vi "Results_file_Plotter.vi"() -> ()   [LabVIEW 2016]
uses:
  Anemometry/Anemometry Sub Vis/Data_plotting_vis/Plot_Slice.ctl
  Anemometry/Anemometry Sub Vis/Data_plotting_vis/Plotter_Mode.ctl
  Anemometry/Anemometry Sub Vis/Data_plotting_vis/Data_File_Type.ctl
  subVIs/PlotProperty.ctl
  Anemometry/Anemometry Sub Vis/File/Setup_Filetype.ctl
  Anemometry/Anemometry Sub Vis/Controls/Global_mode.ctl
  Anemometry/Anemometry Sub Vis/Data_plotting_vis/Error_bars_index.ctl
  Anemometry/Anemometry Sub Vis/Data_plotting_vis/Results_plotter_Global.vi
  Instance           1 28Saved   Results_file_Plotter .vi
  Anemometry/Anemometry Sub Vis/Globals/Constants_global.vi
  Anemometry/Anemometry Sub Vis/Globals/Trav_pos_global.vi
panel:
  out "Index when last displayed":i32
  out "Index when last plotted":i32
  in  "Tab Control":T1(tab)=enum."Cursor"
  in  "Template":path
  in  "Empty":bool
  in  "Result files to read":path[](array[path])
  in  "Add results file":bool
  in  "File Types to Read":T2
  in  "Dot Plot?":bool
  in  "Vector Plot?":bool
  out "2nd Add label":string
  out "First Add label":string
  in  "Additional X Values":dbl[](array[numeric]) format="%.2f"
  in  "Additional Y Values":dbl[](array[numeric]) format="%.2f"
  in  "Show Results Space Analysis":bool
  in  "Show Plot Space Analysis":bool
  in  "Multi Ordinate":i32[](listbox)
  in  "Multi Ordinate?":bool
  in  "Ordinate":u16(ring) items=["File", "Date", "Time", "Comments", "Uref", "Screens_Downstream of Heaters", "Spires", "Spires Used", "Roughness", "Roughness Used", "Roughness Elements 1st Row X(m)", "Start of Cooled Floor X(m)", "Chilled Water Temp", "Inlet_Temp Average", "Av Floor Temp", "Max deltaT", "X (mm)", "Y (mm)", "Z (mm)", "Z (m)", "U/Uref", "V/Uref", "W/Uref", "u^2/Uref^2", "v^2/Uref^2", "w^2/Uref^2", "uv/Uref^2", "-uw/Uref^2", "Corr wt", "Inlet Profile", "DeltaT", "t^2", "ut", "Corr ut", "wt", "Grad Ri", "Flux Ri", "B-V Freq N", "Inlet DeltaT", "DeltaT/DeltaTmax", "T thermistor", "dT/dZ", "dU/dZ", "Inlet Delta_Set", "u'/U", "w'/U", "W/U", "Location XY", "Location XZ", "U m/s", "V m/s", "W m/s", "u^2", "v^2", "w^2", "Speed/Uref", "T cw", "Flow Meas Time", "Profile", "t'/T", "t'", "uv", "uw", "EnFlo Lab Hygrometry Dew Point temp", "EnFlo Lab Hygrometry Dew Point temp_PN", "Multi Run Start Time", "T cw Offset A", "T cw Grad B", "LDA (U) Standard Error in Mean", "LDA (U) Standard Error in Variance", "LDA (V) Standard Error in Mean", "LDA (V) Standard Error in Variance", "LDA (W) Standard Error in Mean", "LDA (W) Standard Error in Variance", "U/Uref Err", "u^2/Uref^2 Err", "V/Uref Err", "v^2/Uref^2 Err", "W/Uref Err", "w^2/Uref^2 Err", "Inlet Temp", "Inlet Setpoint", "Inlet Temp Error", "Seconds since 1st Jan", "Uni Chilled Water Temp", "Raw Data Filename", "Inlet Temp Z=1450", "Inlet Temp Z=1350", "Inlet Temp Z=1250", "Inlet Temp Z=1150", "Inlet Temp Z=1050", "Inlet Temp Z=950", "Inlet Temp Z=850", "Inlet Temp Z=750", "Inlet Temp Z=650", "Inlet Temp Z=550", "Inlet Temp Z=450", "Inlet Temp Z=350", "Inlet Temp Z=250", "Inlet Temp Z=150", "Inlet Temp Z=50", "Inlet Setpoint Z=1450", "Inlet Setpoint Z=1350", "Inlet Setpoint Z=1250", "Inlet Setpoint Z=1150", "Inlet Setpoint Z=950", "Inlet Setpoint Z=850", "Inlet Setpoint Z=1050", "Inlet Setpoint Z=750", "Inlet Setpoint Z=650", "Inlet Setpoint Z=550", "Inlet Setpoint Z=450", "Inlet Setpoint Z=350", "Inlet Setpoint Z=250", "Inlet Setpoint Z=150", "Inlet Setpoint Z=50", "Temp Floor_Near 1", "Temp Floor_Far 1", "Temp Floor_Near 2", "Temp Floor_Far 2", "Temp Floor_Near 3", "Temp Floor_Far 3", "Temp Floor_Near 4", "Temp Floor_Far 4", "Temp Floor_Near 5", "Temp Floor_Far 5", "Temp Floor_Near 6", "Temp Floor_Far 6", "Temp Floor_Near 7", "Temp Floor_Far 7", "Temp Floor_Near 8", "Temp Floor_Far 8", "Temp Floor_Near 9", "Temp Floor_Far 9", "Temp Floor_Near 10", "Temp Floor_Far 10", "Temp Floor_Near 11", "Temp Floor_Far 11", "Temp Floor_Near 12", "Temp Floor_Far 12", "LDA (U) E(f)", "LDA (W) E(f)", "CW (T) f.E(f)", "LDA (U) f.E(f)", "LDA (W) f.E(f)", "Folder", "Inst", "EnFlo_Tunnel Usonic_Ref_3 Velocity", "EnFlo_Tunnel Usonic Y+ve Duct Velocity", "EnFlo_Tunnel Usonic Y-ve Duct Velocity", "EnFlo_Tunnel Shaft rpm", "U/Uref3", "U/U_y+ve", "U/U_y-ve", "EnFlo_Tunnel Inlet K_Factor", "LDA U SamplingRate", "LDA W SamplingRate", "EnFlo_Tunnel Chilled Water Valve Dem Pos", "EnFlo_Tunnel Temp Y+ve_Side_Top", "EnFlo_Tunnel Temp Y+ve_Side_Middle", "EnFlo_Tunnel Temp Y+ve_Side_Bottom", "EnFlo_Tunnel Temp Y-ve_Side_Top", "EnFlo_Tunnel Temp Y-ve_Side_Middle", "EnFlo_Tunnel Temp Y-ve_Side_Bottom", "EnFlo Lab labstrat1 Delta T", "University Outside Temp", "EnFlo Lab Hygrometry Rel Humidity", "EnFlo_Tunnel Temp LDA Probe", "Pre Inlet Average Temp", "Inlet Temp At LDA (U) Z", "Hydrosonic Transducer Setting", "EnFlo_Tunnel Pressure Static", "EnFlo_Tunnel Trav1 Pos Z", "EnFlo_Tunnel Trav1 Pos Y", "EnFlo_Tunnel Trav1 Pos X", "speed/Uref", "Turbine", "EnFlo_Tunnel Metadata Hub_1 Xpos", "X/D", "EnFlo_Tunnel Therm 25mm Below Cold Wire", "WT_RPM", "WT_rpm^2", "WT_rpmSkewness", "WT_rpmKurtosis", "WT_rpm'_%", "LDA Laser Green LDD current (A)", "LDA Laser Blue LDD current (A)", "Cold Wire Displacement_X_(mm)", "Aero_Tunnel Speed Meas Velocity", "LDA (U) Timescale Estimate Integrated to 25%", "LDA (W) Timescale Estimate Integrated to 25%", "Frequency (Hz)", "Green LDA (U) E(f)", "EnFlo_Tunnel Ref Pitot Velocity", "Upitot/Uref", "CW (T) Mean Voltage", "K Factor 1st Honeycomb", "K Factor 1st Screen", "K Factor 2nd_Screen", "K Factor 2nd Honeycomb Heaters Screen", "LDA (U) & LDA (W) Standard Error uw", "-uw/Uref^2 Err", "Multi Run Row Number", "EnFlo_Tunnel Exit Duct Top Temp", "EnFlo_Tunnel Exit Duct Temp", "Av Exit Duct Temp", "Heat Ex Div Valve Dem Pos", "EnFlo_Tunnel Exit Duct Dem Temp", "Inlet Temp St Deviation", "Inlet Door Heaters Dem Power%"]
  in  "Intensity Plot?":bool
  in  "Absisca":u16(ring) items=["File", "Date", "Time", "Comments", "Uref", "Screens_Downstream of Heaters", "Spires", "Spires Used", "Roughness", "Roughness Used", "Roughness Elements 1st Row X(m)", "Start of Cooled Floor X(m)", "Chilled Water Temp", "Inlet_Temp Average", "Av Floor Temp", "Max deltaT", "X (mm)", "Y (mm)", "Z (mm)", "Z (m)", "U/Uref", "V/Uref", "W/Uref", "u^2/Uref^2", "v^2/Uref^2", "w^2/Uref^2", "uv/Uref^2", "-uw/Uref^2", "Corr wt", "Inlet Profile", "DeltaT", "t^2", "ut", "Corr ut", "wt", "Grad Ri", "Flux Ri", "B-V Freq N", "Inlet DeltaT", "DeltaT/DeltaTmax", "T thermistor", "dT/dZ", "dU/dZ", "Inlet Delta_Set", "u'/U", "w'/U", "W/U", "Location XY", "Location XZ", "U m/s", "V m/s", "W m/s", "u^2", "v^2", "w^2", "Speed/Uref", "T cw", "Flow Meas Time", "Profile", "t'/T", "t'", "uv", "uw", "EnFlo Lab Hygrometry Dew Point temp", "EnFlo Lab Hygrometry Dew Point temp_PN", "Multi Run Start Time", "T cw Offset A", "T cw Grad B", "LDA (U) Standard Error in Mean", "LDA (U) Standard Error in Variance", "LDA (V) Standard Error in Mean", "LDA (V) Standard Error in Variance", "LDA (W) Standard Error in Mean", "LDA (W) Standard Error in Variance", "U/Uref Err", "u^2/Uref^2 Err", "V/Uref Err", "v^2/Uref^2 Err", "W/Uref Err", "w^2/Uref^2 Err", "Inlet Temp", "Inlet Setpoint", "Inlet Temp Error", "Seconds since 1st Jan", "Uni Chilled Water Temp", "Raw Data Filename", "Inlet Temp Z=1450", "Inlet Temp Z=1350", "Inlet Temp Z=1250", "Inlet Temp Z=1150", "Inlet Temp Z=1050", "Inlet Temp Z=950", "Inlet Temp Z=850", "Inlet Temp Z=750", "Inlet Temp Z=650", "Inlet Temp Z=550", "Inlet Temp Z=450", "Inlet Temp Z=350", "Inlet Temp Z=250", "Inlet Temp Z=150", "Inlet Temp Z=50", "Inlet Setpoint Z=1450", "Inlet Setpoint Z=1350", "Inlet Setpoint Z=1250", "Inlet Setpoint Z=1150", "Inlet Setpoint Z=950", "Inlet Setpoint Z=850", "Inlet Setpoint Z=1050", "Inlet Setpoint Z=750", "Inlet Setpoint Z=650", "Inlet Setpoint Z=550", "Inlet Setpoint Z=450", "Inlet Setpoint Z=350", "Inlet Setpoint Z=250", "Inlet Setpoint Z=150", "Inlet Setpoint Z=50", "Temp Floor_Near 1", "Temp Floor_Far 1", "Temp Floor_Near 2", "Temp Floor_Far 2", "Temp Floor_Near 3", "Temp Floor_Far 3", "Temp Floor_Near 4", "Temp Floor_Far 4", "Temp Floor_Near 5", "Temp Floor_Far 5", "Temp Floor_Near 6", "Temp Floor_Far 6", "Temp Floor_Near 7", "Temp Floor_Far 7", "Temp Floor_Near 8", "Temp Floor_Far 8", "Temp Floor_Near 9", "Temp Floor_Far 9", "Temp Floor_Near 10", "Temp Floor_Far 10", "Temp Floor_Near 11", "Temp Floor_Far 11", "Temp Floor_Near 12", "Temp Floor_Far 12", "LDA (U) E(f)", "LDA (W) E(f)", "CW (T) f.E(f)", "LDA (U) f.E(f)", "LDA (W) f.E(f)", "Folder", "Inst", "EnFlo_Tunnel Usonic_Ref_3 Velocity", "EnFlo_Tunnel Usonic Y+ve Duct Velocity", "EnFlo_Tunnel Usonic Y-ve Duct Velocity", "EnFlo_Tunnel Shaft rpm", "U/Uref3", "U/U_y+ve", "U/U_y-ve", "EnFlo_Tunnel Inlet K_Factor", "LDA U SamplingRate", "LDA W SamplingRate", "EnFlo_Tunnel Chilled Water Valve Dem Pos", "EnFlo_Tunnel Temp Y+ve_Side_Top", "EnFlo_Tunnel Temp Y+ve_Side_Middle", "EnFlo_Tunnel Temp Y+ve_Side_Bottom", "EnFlo_Tunnel Temp Y-ve_Side_Top", "EnFlo_Tunnel Temp Y-ve_Side_Middle", "EnFlo_Tunnel Temp Y-ve_Side_Bottom", "EnFlo Lab labstrat1 Delta T", "University Outside Temp", "EnFlo Lab Hygrometry Rel Humidity", "EnFlo_Tunnel Temp LDA Probe", "Pre Inlet Average Temp", "Inlet Temp At LDA (U) Z", "Hydrosonic Transducer Setting", "EnFlo_Tunnel Pressure Static", "EnFlo_Tunnel Trav1 Pos Z", "EnFlo_Tunnel Trav1 Pos Y", "EnFlo_Tunnel Trav1 Pos X", "speed/Uref", "Turbine", "EnFlo_Tunnel Metadata Hub_1 Xpos", "X/D", "EnFlo_Tunnel Therm 25mm Below Cold Wire", "WT_RPM", "WT_rpm^2", "WT_rpmSkewness", "WT_rpmKurtosis", "WT_rpm'_%", "LDA Laser Green LDD current (A)", "LDA Laser Blue LDD current (A)", "Cold Wire Displacement_X_(mm)", "Aero_Tunnel Speed Meas Velocity", "LDA (U) Timescale Estimate Integrated to 25%", "LDA (W) Timescale Estimate Integrated to 25%", "Frequency (Hz)", "Green LDA (U) E(f)", "EnFlo_Tunnel Ref Pitot Velocity", "Upitot/Uref", "CW (T) Mean Voltage", "K Factor 1st Honeycomb", "K Factor 1st Screen", "K Factor 2nd_Screen", "K Factor 2nd Honeycomb Heaters Screen", "LDA (U) & LDA (W) Standard Error uw", "-uw/Uref^2 Err", "Multi Run Row Number", "EnFlo_Tunnel Exit Duct Top Temp", "EnFlo_Tunnel Exit Duct Temp", "Av Exit Duct Temp", "Heat Ex Div Valve Dem Pos", "EnFlo_Tunnel Exit Duct Dem Temp", "Inlet Temp St Deviation", "Inlet Door Heaters Dem Power%"]
  in  "Job Directory":path
  in  "Save Averaged rows":bool
  in  "Save Surface Fit":bool
  in  "Output Filename":path
  in  "Save Data in Rows":bool
  in  "Save Plot data":bool
  in  "Header":string
  in  "Process Point":bool
  in  "Kill Point":bool
  out "Table":string[][](table)
  in  "ShowPix":bool
  in  "Post Process Plotted Data":bool
  in  "...using routine":string
  in  "Calculate new metadata":bool
  in  "Add /Edit metadata":bool
  in  "Delete Plotted data from file":bool
  in  "Raw DF in Orig Pos?":bool
  in  "Edit Raw Data Files?":bool
  in  "Save Setup":bool
  in  "Load Setup":bool
  in  "Save Setup Interval (s)":dbl=600.0
  out "Uadvec":dbl
  in  "Ordinate Name":string
  in  "Filter 6":u16(ring)
  in  "Add Inlet Temperature offset":bool
  in  "Plot EnFlo Tunnel Display":bool
  in  "SeriesColouring":T4={"PlotVariable"=enum."Symbol", "YellowSelector"=enum."Colour", "RedSelector"=enum."Shade"}
  in  "InterpolationStyle":T5(ring)=enum."Line"
  in  "TinyPoints?":bool
  in  "stop":bool
  out "Current":string="Graph Scales"
  in  "Single Series":i32[](listbox)=[0]
  in  "Edit Template File":bool
  out "nRows":i32
  in  "Filter Bins 2":i32[](listbox)=[0]
  in  "Filter 5":u16(ring) items=["Show All (33)", "03-Jan-17 (33)", "NOT 03-Jan-17 (0)"]
  in  "Filter 4":u16(ring) items=["Show All (33)", "BLANK (33)", "NOT BLANK (0)"]
  in  "Filter 3":u16(ring) items=["Show All (33)", "#DIV/0! (2)", "Single Measurement (31)", "NOT #DIV/0! (31)", "NOT Single Measurement (2)"]
  in  "Filter Array":u16[](array[ring])=[0, 0, 0, 0, 0, 0] items=["Don't Filter", "File", "Date", "Time", "Comments", "Uref", "Screens_Downstream of Heaters", "Spires", "Spires Used", "Roughness", "Roughness Used", "Roughness Elements 1st Row X(m)", "Start of Cooled Floor X(m)", "Chilled Water Temp", "Inlet_Temp Average", "Av Floor Temp", "Max deltaT", "X (mm)", "Y (mm)", "Z (mm)", "Z (m)", "U/Uref", "V/Uref", "W/Uref", "u^2/Uref^2", "v^2/Uref^2", "w^2/Uref^2", "uv/Uref^2", "-uw/Uref^2", "Corr wt", "Inlet Profile", "DeltaT", "t^2", "ut", "Corr ut", "wt", "Grad Ri", "Flux Ri", "B-V Freq N", "Inlet DeltaT", "DeltaT/DeltaTmax", "T thermistor", "dT/dZ", "dU/dZ", "Inlet Delta_Set", "u'/U", "w'/U", "W/U", "Location XY", "Location XZ", "U m/s", "V m/s", "W m/s", "u^2", "v^2", "w^2", "Speed/Uref", "T cw", "Flow Meas Time", "Profile", "t'/T", "t'", "uv", "uw", "EnFlo Lab Hygrometry Dew Point temp", "EnFlo Lab Hygrometry Dew Point temp_PN", "Multi Run Start Time", "T cw Offset A", "T cw Grad B", "LDA (U) Standard Error in Mean", "LDA (U) Standard Error in Variance", "LDA (V) Standard Error in Mean", "LDA (V) Standard Error in Variance", "LDA (W) Standard Error in Mean", "LDA (W) Standard Error in Variance", "U/Uref Err", "u^2/Uref^2 Err", "V/Uref Err", "v^2/Uref^2 Err", "W/Uref Err", "w^2/Uref^2 Err", "Inlet Temp", "Inlet Setpoint", "Inlet Temp Error", "Seconds since 1st Jan", "Uni Chilled Water Temp", "Raw Data Filename", "Inlet Temp Z=1450", "Inlet Temp Z=1350", "Inlet Temp Z=1250", "Inlet Temp Z=1150", "Inlet Temp Z=1050", "Inlet Temp Z=950", "Inlet Temp Z=850", "Inlet Temp Z=750", "Inlet Temp Z=650", "Inlet Temp Z=550", "Inlet Temp Z=450", "Inlet Temp Z=350", "Inlet Temp Z=250", "Inlet Temp Z=150", "Inlet Temp Z=50", "Inlet Setpoint Z=1450", "Inlet Setpoint Z=1350", "Inlet Setpoint Z=1250", "Inlet Setpoint Z=1150", "Inlet Setpoint Z=950", "Inlet Setpoint Z=850", "Inlet Setpoint Z=1050", "Inlet Setpoint Z=750", "Inlet Setpoint Z=650", "Inlet Setpoint Z=550", "Inlet Setpoint Z=450", "Inlet Setpoint Z=350", "Inlet Setpoint Z=250", "Inlet Setpoint Z=150", "Inlet Setpoint Z=50", "Temp Floor_Near 1", "Temp Floor_Far 1", "Temp Floor_Near 2", "Temp Floor_Far 2", "Temp Floor_Near 3", "Temp Floor_Far 3", "Temp Floor_Near 4", "Temp Floor_Far 4", "Temp Floor_Near 5", "Temp Floor_Far 5", "Temp Floor_Near 6", "Temp Floor_Far 6", "Temp Floor_Near 7", "Temp Floor_Far 7", "Temp Floor_Near 8", "Temp Floor_Far 8", "Temp Floor_Near 9", "Temp Floor_Far 9", "Temp Floor_Near 10", "Temp Floor_Far 10", "Temp Floor_Near 11", "Temp Floor_Far 11", "Temp Floor_Near 12", "Temp Floor_Far 12", "LDA (U) E(f)", "LDA (W) E(f)", "CW (T) f.E(f)", "LDA (U) f.E(f)", "LDA (W) f.E(f)", "Folder", "Inst", "EnFlo_Tunnel Usonic_Ref_3 Velocity", "EnFlo_Tunnel Usonic Y+ve Duct Velocity", "EnFlo_Tunnel Usonic Y-ve Duct Velocity", "EnFlo_Tunnel Shaft rpm", "U/Uref3", "U/U_y+ve", "U/U_y-ve", "EnFlo_Tunnel Inlet K_Factor", "LDA U SamplingRate", "LDA W SamplingRate", "EnFlo_Tunnel Chilled Water Valve Dem Pos", "EnFlo_Tunnel Temp Y+ve_Side_Top", "EnFlo_Tunnel Temp Y+ve_Side_Middle", "EnFlo_Tunnel Temp Y+ve_Side_Bottom", "EnFlo_Tunnel Temp Y-ve_Side_Top", "EnFlo_Tunnel Temp Y-ve_Side_Middle", "EnFlo_Tunnel Temp Y-ve_Side_Bottom", "EnFlo Lab labstrat1 Delta T", "University Outside Temp", "EnFlo Lab Hygrometry Rel Humidity", "EnFlo_Tunnel Temp LDA Probe", "Pre Inlet Average Temp", "Inlet Temp At LDA (U) Z", "Hydrosonic Transducer Setting", "EnFlo_Tunnel Pressure Static", "EnFlo_Tunnel Trav1 Pos Z", "EnFlo_Tunnel Trav1 Pos Y", "EnFlo_Tunnel Trav1 Pos X", "speed/Uref", "Turbine", "EnFlo_Tunnel Metadata Hub_1 Xpos", "X/D", "EnFlo_Tunnel Therm 25mm Below Cold Wire", "WT_RPM", "WT_rpm^2", "WT_rpmSkewness", "WT_rpmKurtosis", "WT_rpm'_%", "LDA Laser Green LDD current (A)", "LDA Laser Blue LDD current (A)", "Cold Wire Displacement_X_(mm)", "Aero_Tunnel Speed Meas Velocity", "LDA (U) Timescale Estimate Integrated to 25%", "LDA (W) Timescale Estimate Integrated to 25%", "Frequency (Hz)", "Green LDA (U) E(f)", "EnFlo_Tunnel Ref Pitot Velocity", "Upitot/Uref", "CW (T) Mean Voltage", "K Factor 1st Honeycomb", "K Factor 1st Screen", "K Factor 2nd_Screen", "K Factor 2nd Honeycomb Heaters Screen", "LDA (U) & LDA (W) Standard Error uw", "-uw/Uref^2 Err", "Multi Run Row Number", "EnFlo_Tunnel Exit Duct Top Temp", "EnFlo_Tunnel Exit Duct Temp", "Av Exit Duct Temp", "Heat Ex Div Valve Dem Pos", "EnFlo_Tunnel Exit Duct Dem Temp", "Inlet Temp St Deviation", "Inlet Door Heaters Dem Power%"]
  in  "Filter Bins 1":i32[](listbox)=[0]
  in  "Create picture Vi Name":string caption="Picture VI:"
  in  "Save Plot as jpg":bool
  in  "Reload Files":bool
  in  "color and symbol":bool
  out "Selected Row":i32
  out "Selected Row?":bool
  out "Warning!":string
  out "XY Plot":cluster{dbl[], dbl[]}[](graph)
  out "Edit Raw Data Header Info":bool
  out "Intensity Graph":dbl[][](graph)
  in  "Bkgnd Value":dbl
  in  "Update":bool
  in  "Plot Resolution":bool
  in  "Point Size":i32(slide)=1 scale=0.0..10.0
  in  "No of Contours":i32=20
  in  "Slice mode":T6
  in  "Z Ch Name":u16(ring) items=["File", "Date", "Time", "Comments", "Uref", "Screens_Downstream of Heaters", "Spires", "Spires Used", "Roughness", "Roughness Used", "Roughness Elements 1st Row X(m)", "Start of Cooled Floor X(m)", "Chilled Water Temp", "Inlet_Temp Average", "Av Floor Temp", "Max deltaT", "X (mm)", "Y (mm)", "Z (mm)", "Z (m)", "U/Uref", "V/Uref", "W/Uref", "u^2/Uref^2", "v^2/Uref^2", "w^2/Uref^2", "uv/Uref^2", "-uw/Uref^2", "Corr wt", "Inlet Profile", "DeltaT", "t^2", "ut", "Corr ut", "wt", "Grad Ri", "Flux Ri", "B-V Freq N", "Inlet DeltaT", "DeltaT/DeltaTmax", "T thermistor", "dT/dZ", "dU/dZ", "Inlet Delta_Set", "u'/U", "w'/U", "W/U", "Location XY", "Location XZ", "U m/s", "V m/s", "W m/s", "u^2", "v^2", "w^2", "Speed/Uref", "T cw", "Flow Meas Time", "Profile", "t'/T", "t'", "uv", "uw", "EnFlo Lab Hygrometry Dew Point temp", "EnFlo Lab Hygrometry Dew Point temp_PN", "Multi Run Start Time", "T cw Offset A", "T cw Grad B", "LDA (U) Standard Error in Mean", "LDA (U) Standard Error in Variance", "LDA (V) Standard Error in Mean", "LDA (V) Standard Error in Variance", "LDA (W) Standard Error in Mean", "LDA (W) Standard Error in Variance", "U/Uref Err", "u^2/Uref^2 Err", "V/Uref Err", "v^2/Uref^2 Err", "W/Uref Err", "w^2/Uref^2 Err", "Inlet Temp", "Inlet Setpoint", "Inlet Temp Error", "Seconds since 1st Jan", "Uni Chilled Water Temp", "Raw Data Filename", "Inlet Temp Z=1450", "Inlet Temp Z=1350", "Inlet Temp Z=1250", "Inlet Temp Z=1150", "Inlet Temp Z=1050", "Inlet Temp Z=950", "Inlet Temp Z=850", "Inlet Temp Z=750", "Inlet Temp Z=650", "Inlet Temp Z=550", "Inlet Temp Z=450", "Inlet Temp Z=350", "Inlet Temp Z=250", "Inlet Temp Z=150", "Inlet Temp Z=50", "Inlet Setpoint Z=1450", "Inlet Setpoint Z=1350", "Inlet Setpoint Z=1250", "Inlet Setpoint Z=1150", "Inlet Setpoint Z=950", "Inlet Setpoint Z=850", "Inlet Setpoint Z=1050", "Inlet Setpoint Z=750", "Inlet Setpoint Z=650", "Inlet Setpoint Z=550", "Inlet Setpoint Z=450", "Inlet Setpoint Z=350", "Inlet Setpoint Z=250", "Inlet Setpoint Z=150", "Inlet Setpoint Z=50", "Temp Floor_Near 1", "Temp Floor_Far 1", "Temp Floor_Near 2", "Temp Floor_Far 2", "Temp Floor_Near 3", "Temp Floor_Far 3", "Temp Floor_Near 4", "Temp Floor_Far 4", "Temp Floor_Near 5", "Temp Floor_Far 5", "Temp Floor_Near 6", "Temp Floor_Far 6", "Temp Floor_Near 7", "Temp Floor_Far 7", "Temp Floor_Near 8", "Temp Floor_Far 8", "Temp Floor_Near 9", "Temp Floor_Far 9", "Temp Floor_Near 10", "Temp Floor_Far 10", "Temp Floor_Near 11", "Temp Floor_Far 11", "Temp Floor_Near 12", "Temp Floor_Far 12", "LDA (U) E(f)", "LDA (W) E(f)", "CW (T) f.E(f)", "LDA (U) f.E(f)", "LDA (W) f.E(f)", "Folder", "Inst", "EnFlo_Tunnel Usonic_Ref_3 Velocity", "EnFlo_Tunnel Usonic Y+ve Duct Velocity", "EnFlo_Tunnel Usonic Y-ve Duct Velocity", "EnFlo_Tunnel Shaft rpm", "U/Uref3", "U/U_y+ve", "U/U_y-ve", "EnFlo_Tunnel Inlet K_Factor", "LDA U SamplingRate", "LDA W SamplingRate", "EnFlo_Tunnel Chilled Water Valve Dem Pos", "EnFlo_Tunnel Temp Y+ve_Side_Top", "EnFlo_Tunnel Temp Y+ve_Side_Middle", "EnFlo_Tunnel Temp Y+ve_Side_Bottom", "EnFlo_Tunnel Temp Y-ve_Side_Top", "EnFlo_Tunnel Temp Y-ve_Side_Middle", "EnFlo_Tunnel Temp Y-ve_Side_Bottom", "EnFlo Lab labstrat1 Delta T", "University Outside Temp", "EnFlo Lab Hygrometry Rel Humidity", "EnFlo_Tunnel Temp LDA Probe", "Pre Inlet Average Temp", "Inlet Temp At LDA (U) Z", "Hydrosonic Transducer Setting", "EnFlo_Tunnel Pressure Static", "EnFlo_Tunnel Trav1 Pos Z", "EnFlo_Tunnel Trav1 Pos Y", "EnFlo_Tunnel Trav1 Pos X", "speed/Uref", "Turbine", "EnFlo_Tunnel Metadata Hub_1 Xpos", "X/D", "EnFlo_Tunnel Therm 25mm Below Cold Wire", "WT_RPM", "WT_rpm^2", "WT_rpmSkewness", "WT_rpmKurtosis", "WT_rpm'_%", "LDA Laser Green LDD current (A)", "LDA Laser Blue LDD current (A)", "Cold Wire Displacement_X_(mm)", "Aero_Tunnel Speed Meas Velocity", "LDA (U) Timescale Estimate Integrated to 25%", "LDA (W) Timescale Estimate Integrated to 25%", "Frequency (Hz)", "Green LDA (U) E(f)", "EnFlo_Tunnel Ref Pitot Velocity", "Upitot/Uref", "CW (T) Mean Voltage", "K Factor 1st Honeycomb", "K Factor 1st Screen", "K Factor 2nd_Screen", "K Factor 2nd Honeycomb Heaters Screen", "LDA (U) & LDA (W) Standard Error uw", "-uw/Uref^2 Err", "Multi Run Row Number", "EnFlo_Tunnel Exit Duct Top Temp", "EnFlo_Tunnel Exit Duct Temp", "Av Exit Duct Temp", "Heat Ex Div Valve Dem Pos", "EnFlo_Tunnel Exit Duct Dem Temp", "Inlet Temp St Deviation", "Inlet Door Heaters Dem Power%"]
  in  "Y Ch Name":u16(ring) items=["File", "Date", "Time", "Comments", "Uref", "Screens_Downstream of Heaters", "Spires", "Spires Used", "Roughness", "Roughness Used", "Roughness Elements 1st Row X(m)", "Start of Cooled Floor X(m)", "Chilled Water Temp", "Inlet_Temp Average", "Av Floor Temp", "Max deltaT", "X (mm)", "Y (mm)", "Z (mm)", "Z (m)", "U/Uref", "V/Uref", "W/Uref", "u^2/Uref^2", "v^2/Uref^2", "w^2/Uref^2", "uv/Uref^2", "-uw/Uref^2", "Corr wt", "Inlet Profile", "DeltaT", "t^2", "ut", "Corr ut", "wt", "Grad Ri", "Flux Ri", "B-V Freq N", "Inlet DeltaT", "DeltaT/DeltaTmax", "T thermistor", "dT/dZ", "dU/dZ", "Inlet Delta_Set", "u'/U", "w'/U", "W/U", "Location XY", "Location XZ", "U m/s", "V m/s", "W m/s", "u^2", "v^2", "w^2", "Speed/Uref", "T cw", "Flow Meas Time", "Profile", "t'/T", "t'", "uv", "uw", "EnFlo Lab Hygrometry Dew Point temp", "EnFlo Lab Hygrometry Dew Point temp_PN", "Multi Run Start Time", "T cw Offset A", "T cw Grad B", "LDA (U) Standard Error in Mean", "LDA (U) Standard Error in Variance", "LDA (V) Standard Error in Mean", "LDA (V) Standard Error in Variance", "LDA (W) Standard Error in Mean", "LDA (W) Standard Error in Variance", "U/Uref Err", "u^2/Uref^2 Err", "V/Uref Err", "v^2/Uref^2 Err", "W/Uref Err", "w^2/Uref^2 Err", "Inlet Temp", "Inlet Setpoint", "Inlet Temp Error", "Seconds since 1st Jan", "Uni Chilled Water Temp", "Raw Data Filename", "Inlet Temp Z=1450", "Inlet Temp Z=1350", "Inlet Temp Z=1250", "Inlet Temp Z=1150", "Inlet Temp Z=1050", "Inlet Temp Z=950", "Inlet Temp Z=850", "Inlet Temp Z=750", "Inlet Temp Z=650", "Inlet Temp Z=550", "Inlet Temp Z=450", "Inlet Temp Z=350", "Inlet Temp Z=250", "Inlet Temp Z=150", "Inlet Temp Z=50", "Inlet Setpoint Z=1450", "Inlet Setpoint Z=1350", "Inlet Setpoint Z=1250", "Inlet Setpoint Z=1150", "Inlet Setpoint Z=950", "Inlet Setpoint Z=850", "Inlet Setpoint Z=1050", "Inlet Setpoint Z=750", "Inlet Setpoint Z=650", "Inlet Setpoint Z=550", "Inlet Setpoint Z=450", "Inlet Setpoint Z=350", "Inlet Setpoint Z=250", "Inlet Setpoint Z=150", "Inlet Setpoint Z=50", "Temp Floor_Near 1", "Temp Floor_Far 1", "Temp Floor_Near 2", "Temp Floor_Far 2", "Temp Floor_Near 3", "Temp Floor_Far 3", "Temp Floor_Near 4", "Temp Floor_Far 4", "Temp Floor_Near 5", "Temp Floor_Far 5", "Temp Floor_Near 6", "Temp Floor_Far 6", "Temp Floor_Near 7", "Temp Floor_Far 7", "Temp Floor_Near 8", "Temp Floor_Far 8", "Temp Floor_Near 9", "Temp Floor_Far 9", "Temp Floor_Near 10", "Temp Floor_Far 10", "Temp Floor_Near 11", "Temp Floor_Far 11", "Temp Floor_Near 12", "Temp Floor_Far 12", "LDA (U) E(f)", "LDA (W) E(f)", "CW (T) f.E(f)", "LDA (U) f.E(f)", "LDA (W) f.E(f)", "Folder", "Inst", "EnFlo_Tunnel Usonic_Ref_3 Velocity", "EnFlo_Tunnel Usonic Y+ve Duct Velocity", "EnFlo_Tunnel Usonic Y-ve Duct Velocity", "EnFlo_Tunnel Shaft rpm", "U/Uref3", "U/U_y+ve", "U/U_y-ve", "EnFlo_Tunnel Inlet K_Factor", "LDA U SamplingRate", "LDA W SamplingRate", "EnFlo_Tunnel Chilled Water Valve Dem Pos", "EnFlo_Tunnel Temp Y+ve_Side_Top", "EnFlo_Tunnel Temp Y+ve_Side_Middle", "EnFlo_Tunnel Temp Y+ve_Side_Bottom", "EnFlo_Tunnel Temp Y-ve_Side_Top", "EnFlo_Tunnel Temp Y-ve_Side_Middle", "EnFlo_Tunnel Temp Y-ve_Side_Bottom", "EnFlo Lab labstrat1 Delta T", "University Outside Temp", "EnFlo Lab Hygrometry Rel Humidity", "EnFlo_Tunnel Temp LDA Probe", "Pre Inlet Average Temp", "Inlet Temp At LDA (U) Z", "Hydrosonic Transducer Setting", "EnFlo_Tunnel Pressure Static", "EnFlo_Tunnel Trav1 Pos Z", "EnFlo_Tunnel Trav1 Pos Y", "EnFlo_Tunnel Trav1 Pos X", "speed/Uref", "Turbine", "EnFlo_Tunnel Metadata Hub_1 Xpos", "X/D", "EnFlo_Tunnel Therm 25mm Below Cold Wire", "WT_RPM", "WT_rpm^2", "WT_rpmSkewness", "WT_rpmKurtosis", "WT_rpm'_%", "LDA Laser Green LDD current (A)", "LDA Laser Blue LDD current (A)", "Cold Wire Displacement_X_(mm)", "Aero_Tunnel Speed Meas Velocity", "LDA (U) Timescale Estimate Integrated to 25%", "LDA (W) Timescale Estimate Integrated to 25%", "Frequency (Hz)", "Green LDA (U) E(f)", "EnFlo_Tunnel Ref Pitot Velocity", "Upitot/Uref", "CW (T) Mean Voltage", "K Factor 1st Honeycomb", "K Factor 1st Screen", "K Factor 2nd_Screen", "K Factor 2nd Honeycomb Heaters Screen", "LDA (U) & LDA (W) Standard Error uw", "-uw/Uref^2 Err", "Multi Run Row Number", "EnFlo_Tunnel Exit Duct Top Temp", "EnFlo_Tunnel Exit Duct Temp", "Av Exit Duct Temp", "Heat Ex Div Valve Dem Pos", "EnFlo_Tunnel Exit Duct Dem Temp", "Inlet Temp St Deviation", "Inlet Door Heaters Dem Power%"]
  in  "X Ch Name":u16(ring) items=["File", "Date", "Time", "Comments", "Uref", "Screens_Downstream of Heaters", "Spires", "Spires Used", "Roughness", "Roughness Used", "Roughness Elements 1st Row X(m)", "Start of Cooled Floor X(m)", "Chilled Water Temp", "Inlet_Temp Average", "Av Floor Temp", "Max deltaT", "X (mm)", "Y (mm)", "Z (mm)", "Z (m)", "U/Uref", "V/Uref", "W/Uref", "u^2/Uref^2", "v^2/Uref^2", "w^2/Uref^2", "uv/Uref^2", "-uw/Uref^2", "Corr wt", "Inlet Profile", "DeltaT", "t^2", "ut", "Corr ut", "wt", "Grad Ri", "Flux Ri", "B-V Freq N", "Inlet DeltaT", "DeltaT/DeltaTmax", "T thermistor", "dT/dZ", "dU/dZ", "Inlet Delta_Set", "u'/U", "w'/U", "W/U", "Location XY", "Location XZ", "U m/s", "V m/s", "W m/s", "u^2", "v^2", "w^2", "Speed/Uref", "T cw", "Flow Meas Time", "Profile", "t'/T", "t'", "uv", "uw", "EnFlo Lab Hygrometry Dew Point temp", "EnFlo Lab Hygrometry Dew Point temp_PN", "Multi Run Start Time", "T cw Offset A", "T cw Grad B", "LDA (U) Standard Error in Mean", "LDA (U) Standard Error in Variance", "LDA (V) Standard Error in Mean", "LDA (V) Standard Error in Variance", "LDA (W) Standard Error in Mean", "LDA (W) Standard Error in Variance", "U/Uref Err", "u^2/Uref^2 Err", "V/Uref Err", "v^2/Uref^2 Err", "W/Uref Err", "w^2/Uref^2 Err", "Inlet Temp", "Inlet Setpoint", "Inlet Temp Error", "Seconds since 1st Jan", "Uni Chilled Water Temp", "Raw Data Filename", "Inlet Temp Z=1450", "Inlet Temp Z=1350", "Inlet Temp Z=1250", "Inlet Temp Z=1150", "Inlet Temp Z=1050", "Inlet Temp Z=950", "Inlet Temp Z=850", "Inlet Temp Z=750", "Inlet Temp Z=650", "Inlet Temp Z=550", "Inlet Temp Z=450", "Inlet Temp Z=350", "Inlet Temp Z=250", "Inlet Temp Z=150", "Inlet Temp Z=50", "Inlet Setpoint Z=1450", "Inlet Setpoint Z=1350", "Inlet Setpoint Z=1250", "Inlet Setpoint Z=1150", "Inlet Setpoint Z=950", "Inlet Setpoint Z=850", "Inlet Setpoint Z=1050", "Inlet Setpoint Z=750", "Inlet Setpoint Z=650", "Inlet Setpoint Z=550", "Inlet Setpoint Z=450", "Inlet Setpoint Z=350", "Inlet Setpoint Z=250", "Inlet Setpoint Z=150", "Inlet Setpoint Z=50", "Temp Floor_Near 1", "Temp Floor_Far 1", "Temp Floor_Near 2", "Temp Floor_Far 2", "Temp Floor_Near 3", "Temp Floor_Far 3", "Temp Floor_Near 4", "Temp Floor_Far 4", "Temp Floor_Near 5", "Temp Floor_Far 5", "Temp Floor_Near 6", "Temp Floor_Far 6", "Temp Floor_Near 7", "Temp Floor_Far 7", "Temp Floor_Near 8", "Temp Floor_Far 8", "Temp Floor_Near 9", "Temp Floor_Far 9", "Temp Floor_Near 10", "Temp Floor_Far 10", "Temp Floor_Near 11", "Temp Floor_Far 11", "Temp Floor_Near 12", "Temp Floor_Far 12", "LDA (U) E(f)", "LDA (W) E(f)", "CW (T) f.E(f)", "LDA (U) f.E(f)", "LDA (W) f.E(f)", "Folder", "Inst", "EnFlo_Tunnel Usonic_Ref_3 Velocity", "EnFlo_Tunnel Usonic Y+ve Duct Velocity", "EnFlo_Tunnel Usonic Y-ve Duct Velocity", "EnFlo_Tunnel Shaft rpm", "U/Uref3", "U/U_y+ve", "U/U_y-ve", "EnFlo_Tunnel Inlet K_Factor", "LDA U SamplingRate", "LDA W SamplingRate", "EnFlo_Tunnel Chilled Water Valve Dem Pos", "EnFlo_Tunnel Temp Y+ve_Side_Top", "EnFlo_Tunnel Temp Y+ve_Side_Middle", "EnFlo_Tunnel Temp Y+ve_Side_Bottom", "EnFlo_Tunnel Temp Y-ve_Side_Top", "EnFlo_Tunnel Temp Y-ve_Side_Middle", "EnFlo_Tunnel Temp Y-ve_Side_Bottom", "EnFlo Lab labstrat1 Delta T", "University Outside Temp", "EnFlo Lab Hygrometry Rel Humidity", "EnFlo_Tunnel Temp LDA Probe", "Pre Inlet Average Temp", "Inlet Temp At LDA (U) Z", "Hydrosonic Transducer Setting", "EnFlo_Tunnel Pressure Static", "EnFlo_Tunnel Trav1 Pos Z", "EnFlo_Tunnel Trav1 Pos Y", "EnFlo_Tunnel Trav1 Pos X", "speed/Uref", "Turbine", "EnFlo_Tunnel Metadata Hub_1 Xpos", "X/D", "EnFlo_Tunnel Therm 25mm Below Cold Wire", "WT_RPM", "WT_rpm^2", "WT_rpmSkewness", "WT_rpmKurtosis", "WT_rpm'_%", "LDA Laser Green LDD current (A)", "LDA Laser Blue LDD current (A)", "Cold Wire Displacement_X_(mm)", "Aero_Tunnel Speed Meas Velocity", "LDA (U) Timescale Estimate Integrated to 25%", "LDA (W) Timescale Estimate Integrated to 25%", "Frequency (Hz)", "Green LDA (U) E(f)", "EnFlo_Tunnel Ref Pitot Velocity", "Upitot/Uref", "CW (T) Mean Voltage", "K Factor 1st Honeycomb", "K Factor 1st Screen", "K Factor 2nd_Screen", "K Factor 2nd Honeycomb Heaters Screen", "LDA (U) & LDA (W) Standard Error uw", "-uw/Uref^2 Err", "Multi Run Row Number", "EnFlo_Tunnel Exit Duct Top Temp", "EnFlo_Tunnel Exit Duct Temp", "Av Exit Duct Temp", "Heat Ex Div Valve Dem Pos", "EnFlo_Tunnel Exit Duct Dem Temp", "Inlet Temp St Deviation", "Inlet Door Heaters Dem Power%"]
  in  "Resolution":dbl=1.0 min=0.0 format="%.4f"
  out "Surface Area":dbl format="%^_6g"
  out "Surface Integral":dbl format="%^_6g"
  out "Surface Average":dbl format="%^#.6g"
  in  "Full_Res_Results_Folder":path
  out "Last used Template":path
  out "Cursor index":i32
  out "Choosen Path":path
  in  "VI Refnum Calculation":refnum<vi>
  out "Filetype":string[](array[string])
  out "Mode":T7
  out "Plotted rows only?":bool
  in  "type specifier VI Refnum (for type only) 2":refnum<vi>
  in  "type specifier VI Refnum (for type only)":refnum<vi>
  out "Accept Array":bool[][](array[boolean])
  out "Previous slice mode":T6
  out "Slice mode Change?":bool
  out "Non-Blank Rows":bool[](array[boolean])
  out "File Index":i32
  out "Tolerances":dbl[](array[numeric]) format="%.2f"
  in  "Results files choosen":path[](array[path])
  in  "Transpose":bool
  out "Plotted Series":bool[][](array[boolean])
  in  "Results file":path
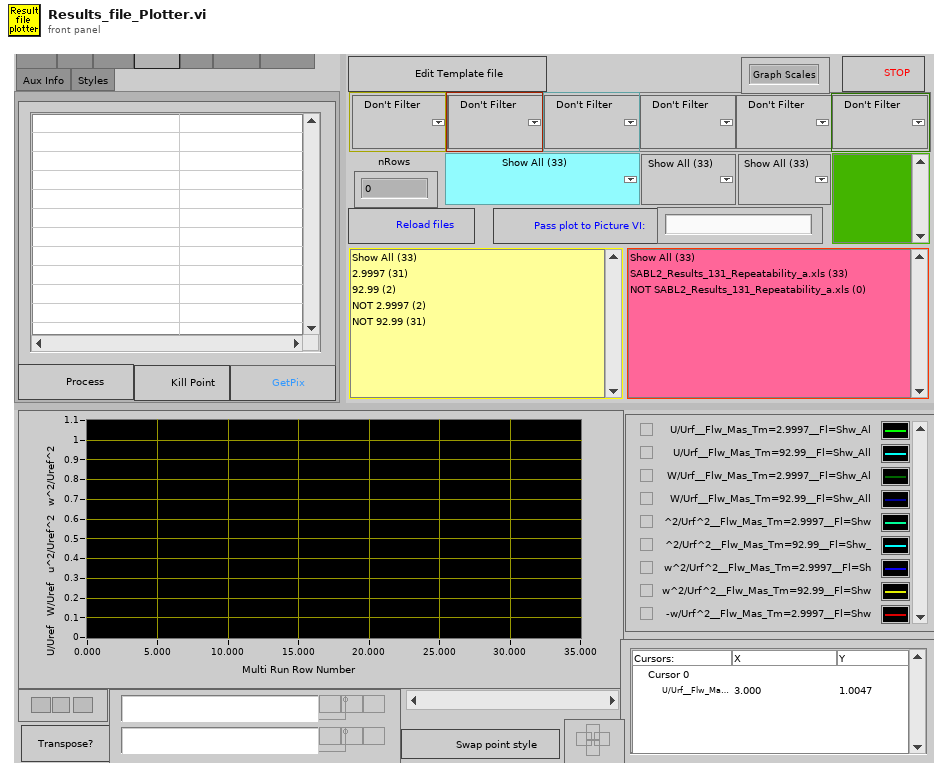
[diagram p1: front panel]
types:
  T1 = enum32{"Load ", "Plot ", "Save ", "Cursor", "Edit", "Setups", "Orphans", "Aux Info", "Styles"}
  T2 = typedef "Data_File_Type.ctl" = enum16{"Read All File Types", "Results Files Only", "Raw Data Files Only", "Calibration Files Only", "Gas Desk Files Only", "Old Results Files Only", "Tabulated Data Files Only"}
  T3 = typedef "PlotProperty.ctl" = enum16{"Colour", "Symbol", "Shade", "Size"}
  T4 = cluster{"PlotVariable":T3, "YellowSelector":T3, "RedSelector":T3}
  T5 = enum16{"Points", "StepLeft", "Line", "StepRight", "StepCentre", "StepEdge"}
  T6 = typedef "Plot_Slice.ctl" = enum16{"XY Slice (Plan)", "YX Slice (Plan)", "YZ Slice (Cross)", "ZY Slice (Cross)", "XZ Slice (Side)", "ZX Slice (Side)"}
  T7 = typedef "Plotter_Mode.ctl" = enum16{"Save file", "Delete unwanted rows", "Edit Values with constants", "Edit values per row", "Edit Raw Data file header", "Post Process Plotted Rows", "Plot EnFlo Tunnel Display", "Add Inlet Temperature Offset"}
  T8 = enum16{"Zero or one", "One", "Zero or more", "One or more"}
  T9 = enum32{"Load ", "Plot ", "Save ", "Cursor", "Edit", "Setups"}
  T10 = typedef "Global_mode.ctl" = enum16{"Read Global", "Load Global From File", "Write Global to File"}
  T11 = enum16{"Edit Existing Template File", "Create New Template File"}
  T12 = enum16{"Show only data summary", "Show data summary", "No data summary"}
  T13 = typedef "Setup_Filetype.ctl" = enum16{"Measurement Setups", "Calibration Setups", "General", "Results File Plotter Setups", "Speed Calib Tweaks"}
  T14 = typedef "All_Setup.ctl" = cluster{"Result files to read":path[], "Template":path, "Transpose":bool, "Additional X Values":dbl[], "Additional Y Values":dbl[], "Ordinate":u16, "Absisca":u16, "Filter Array":u16[], "color and symbol":bool, "Output Filename":path, "Jpg Vi Name":string, "Intensity Plot?":bool, "Multi Ordinate?":bool, "Filter Bins 1":i32[], "Filter Bins 2":i32[], "Multi Ordinate":i32[]}
  T15 = enum16{"Left Button", "Center Button", "Right Button", "Window Close"}
  T16 = enum32{"existing file", "new file", "new or existing file", "existing dir", "new dir", "new or existing dir", "existing file (use LLBs)", "new file (use LLBs)", "new or existing file (use LLBs)", "new or existing file or directory (use LLBs)"}
  T17 = typedef "Error_bars_index.ctl" = cluster{"Upper":i32, "Lower":i32, "St Error":i32}
  T18 = cluster{"Plot Color":u32, "Plot Interpolation":u8, "Point Style":u8, "Line Style":u8, "Fill/Pt. Color":u32, "Line Width":u8, "Bar Plot Style":u8, "Fill To":i16}[]
  T19 = cluster{"X Max":dbl, "Y Max ":dbl, "X Scale":cluster{"Xo":dbl, "delta X":dbl}, "Y Scale":cluster{"Xo":dbl, "delta X":dbl}, "X Values":dbl[], "Y Values":dbl[], "Z Max":dbl, "Z Min":dbl}
  T20 = typedef "Group_Binning.ctl" = cluster{"Index":i32, "Tolerance":dbl, "Precision":string}
  T21 = typedef "LVRectTypeDef.ctl" = cluster{"Left":i16, "Top":i16, "Right":i16, "Bottom":i16}
  T22 = typedef "LVPointTypeDef.ctl" = cluster{"Horizontal":i16, "Vertical":i16}
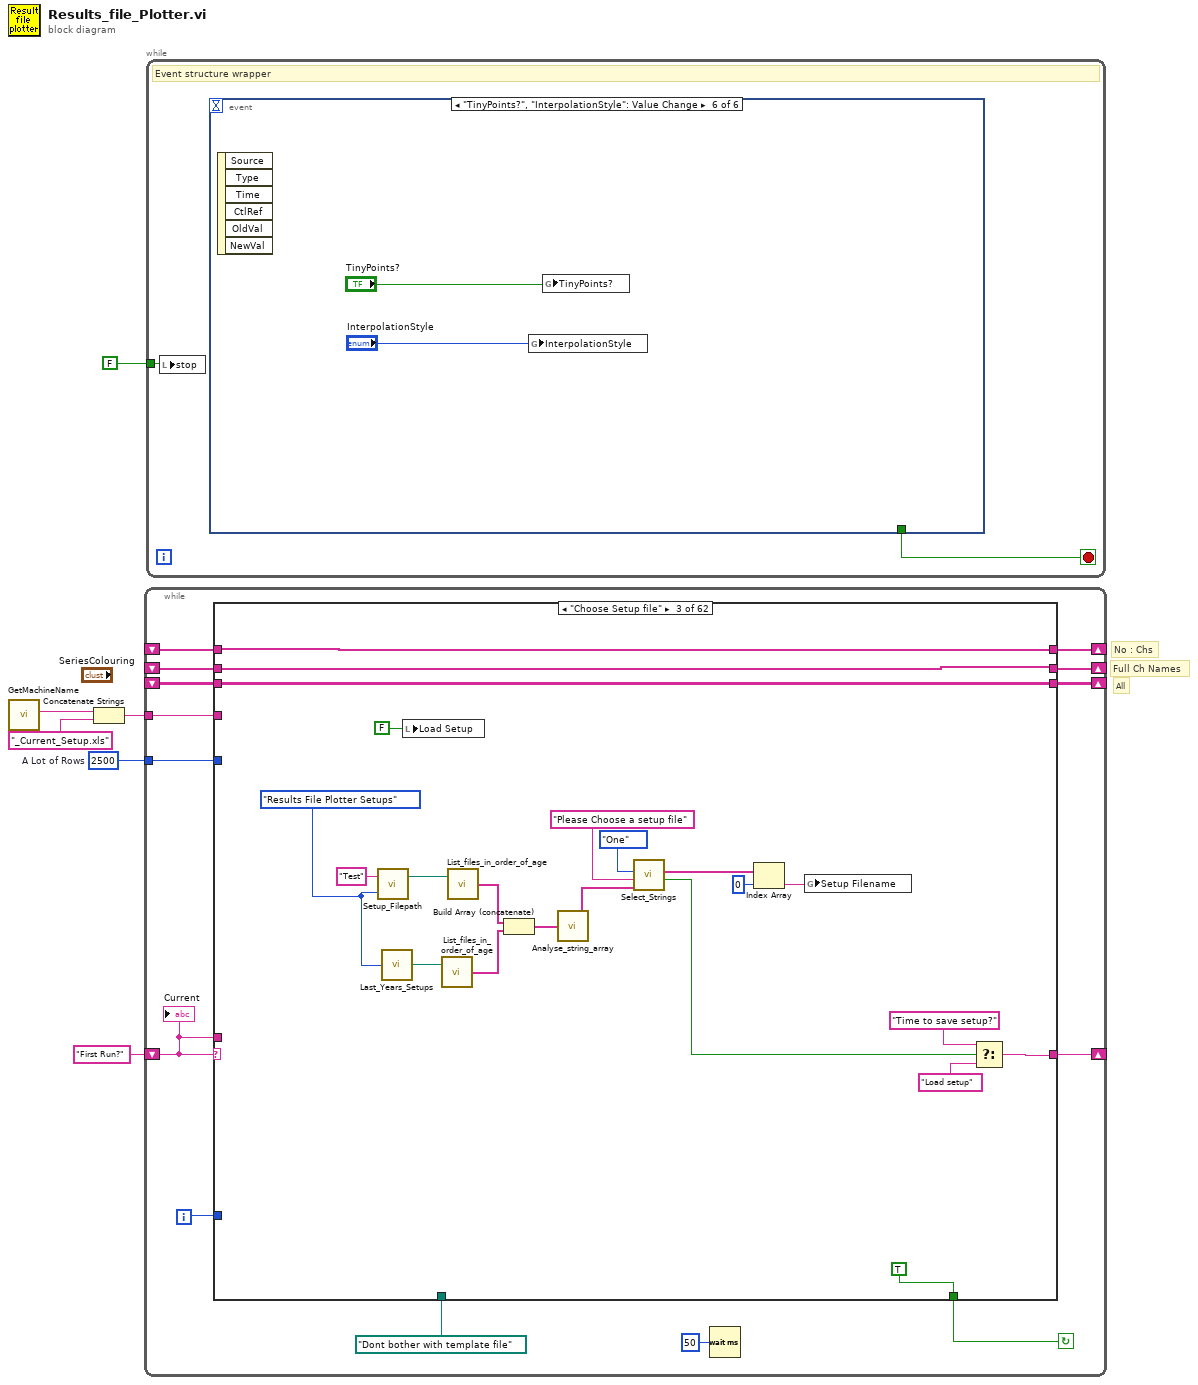
[diagram p0: block diagram]
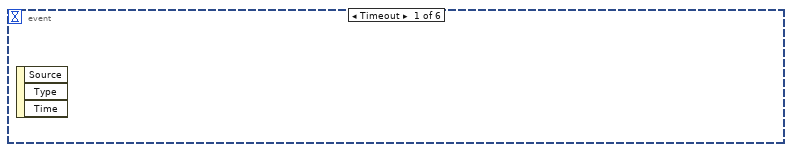
[diagram p2: hidden frame]
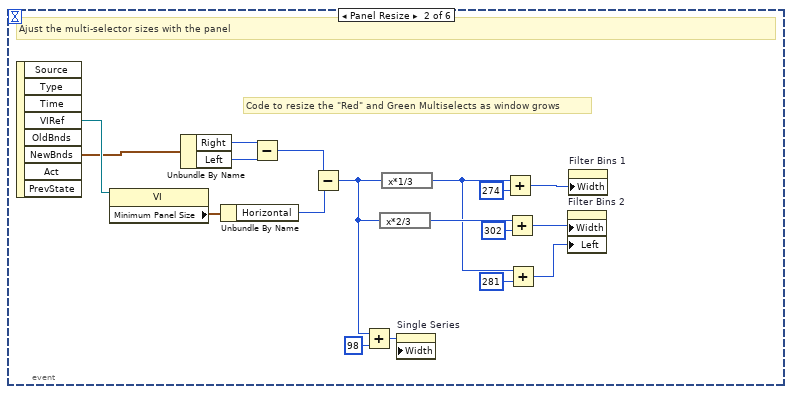
[diagram p3: hidden frame]
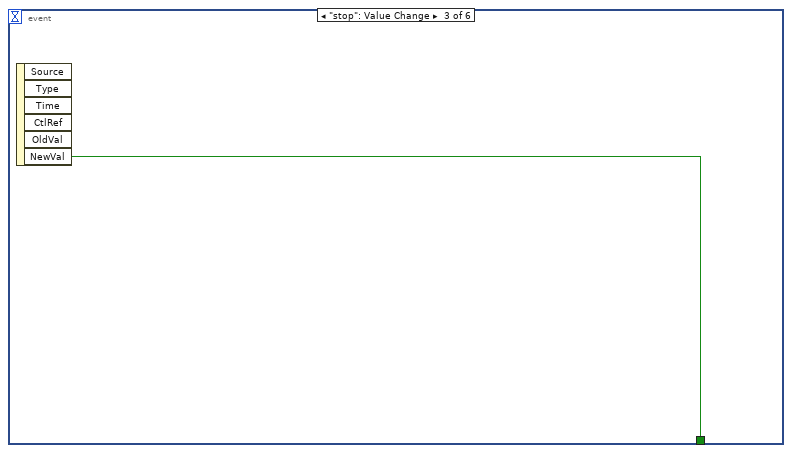
[diagram p4: hidden frame]
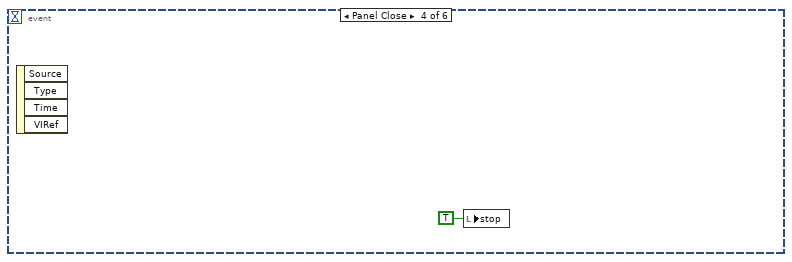
[diagram p5: hidden frame]
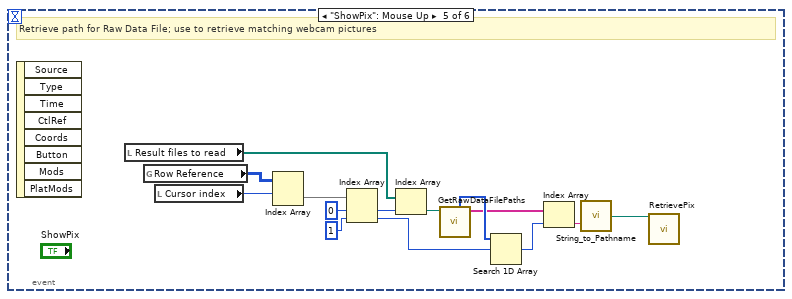
[diagram p6: hidden frame]
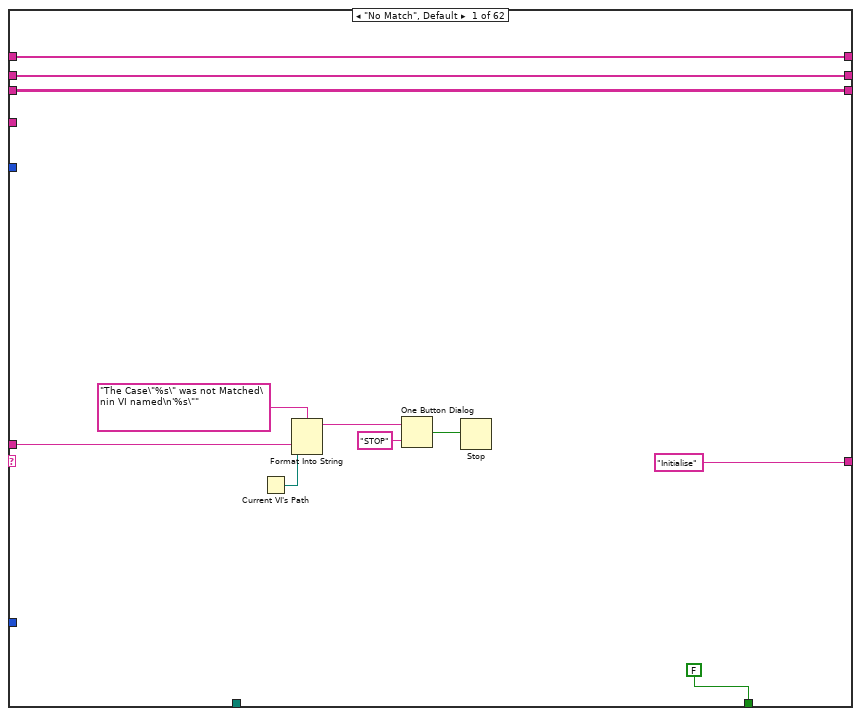
[diagram p7: hidden frame]
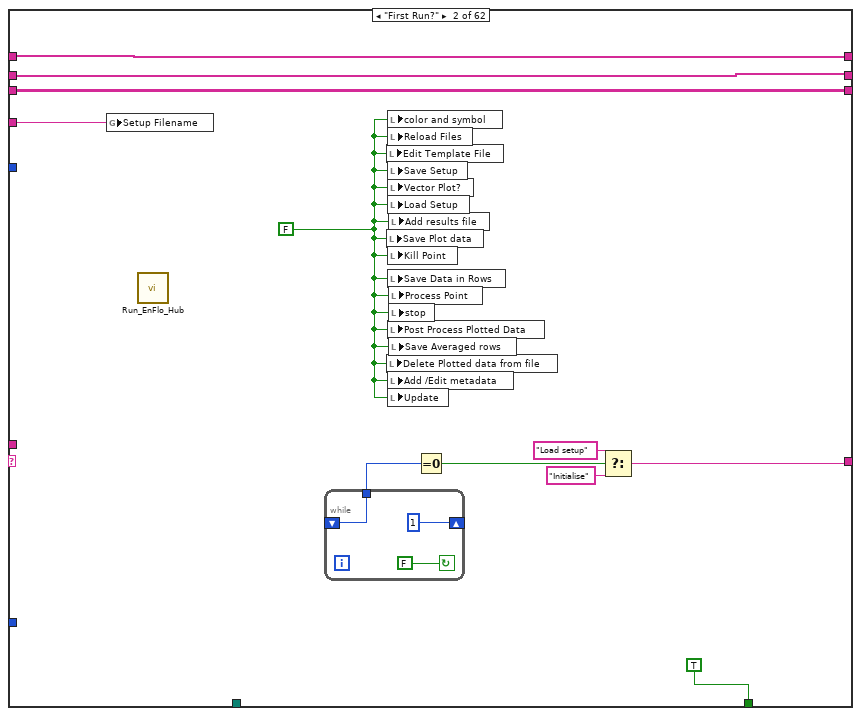
[diagram p8: hidden frame]
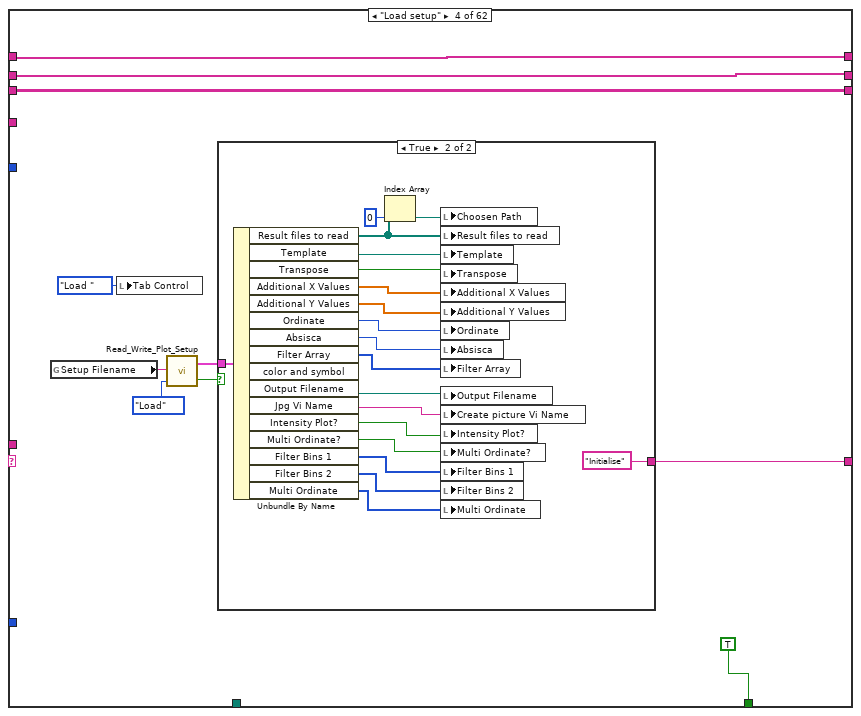
[diagram p9: hidden frame]
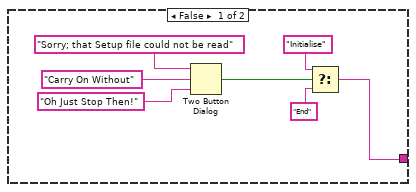
[diagram p10: hidden frame]
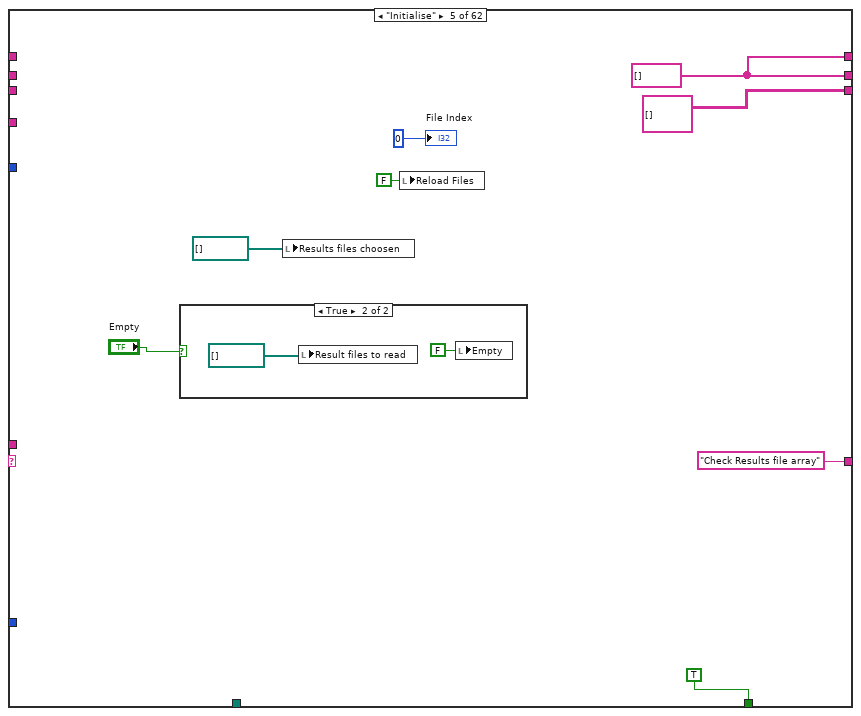
[diagram p11: hidden frame]
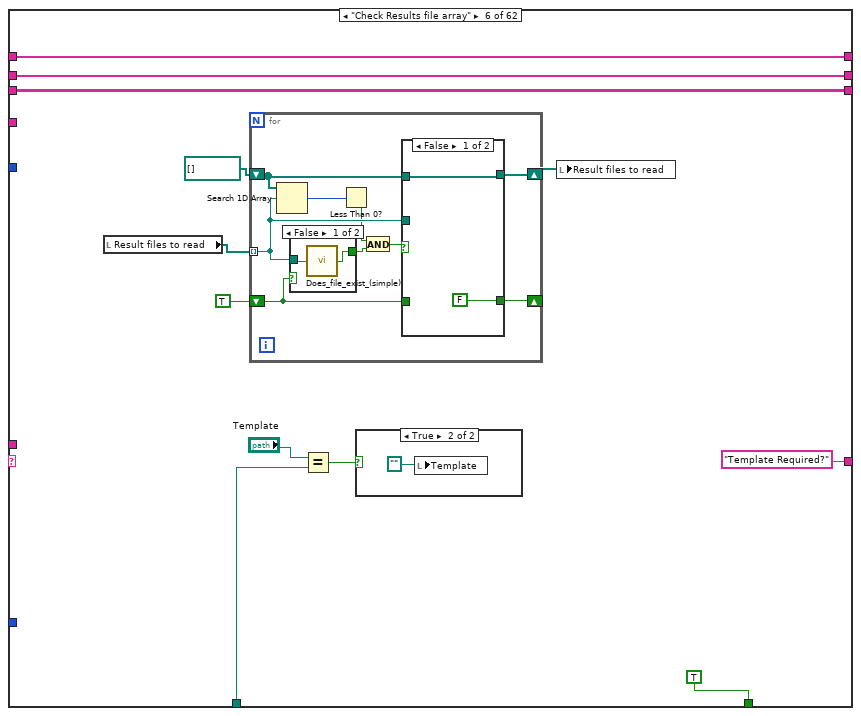
[diagram p13: hidden frame]
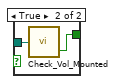
[diagram p15: hidden frame]
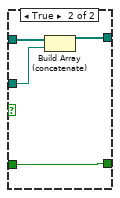
[diagram p16: hidden frame]
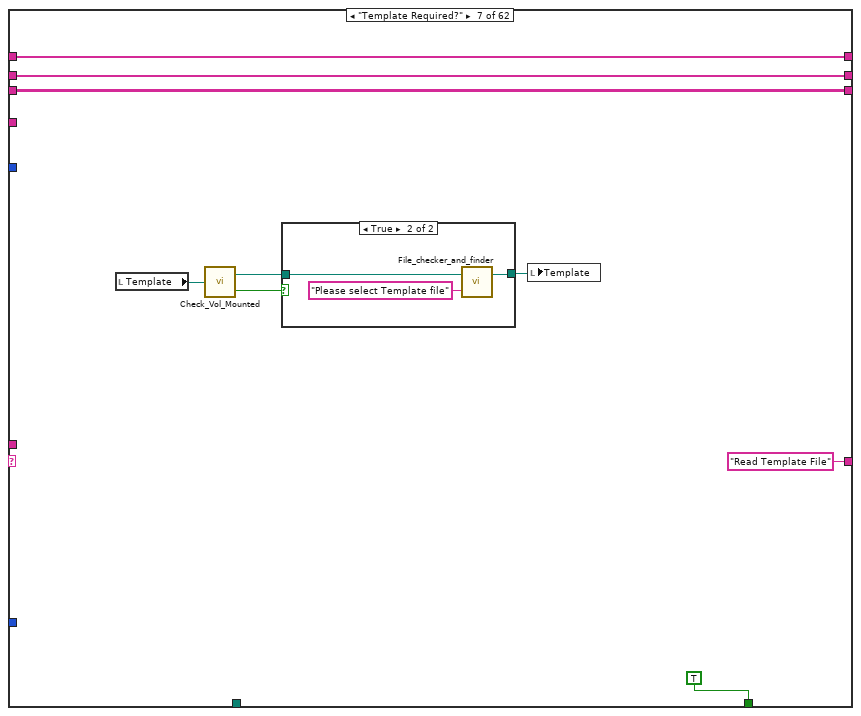
[diagram p17: hidden frame]
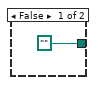
[diagram p18: hidden frame]
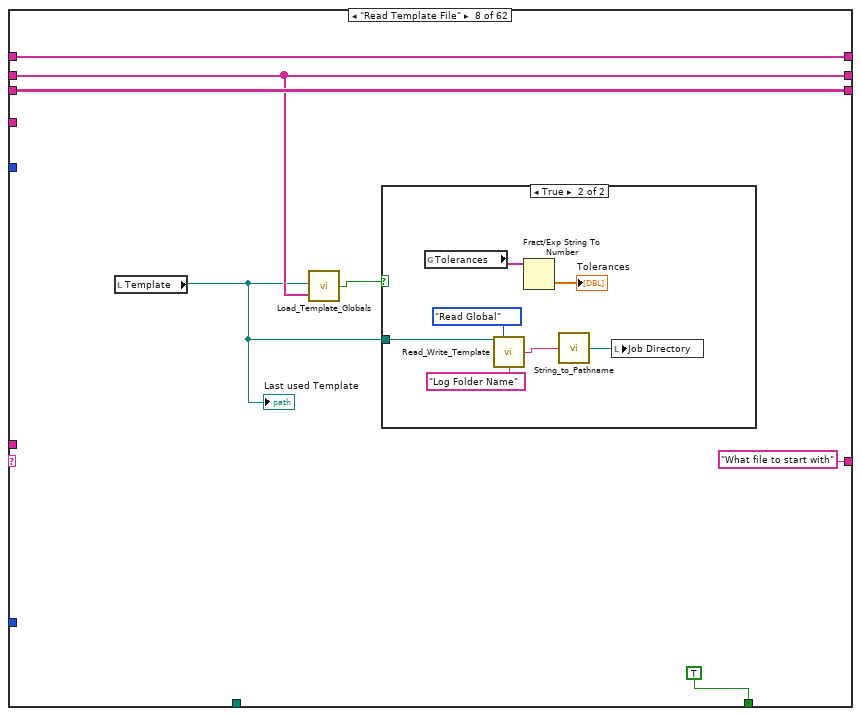
[diagram p19: hidden frame]
diagram:
  w5 = 2500  # A Lot of Rows
  # "No : Chs"
  # "Full Ch Names"
  # "All"
  n1 = call "GetMachineName.vi"() -> ("ComputerName"=w2:string)  [unwired: 11 in]
  n2 = Concatenate Strings(w2, "_Current_Setup.xls" ("Setup filename")) -> (w3:string)
  n3 = while {
    shift-left: _ -> [w13]
    shift-right: [w14] -> _
    shift-left: "First Run?" -> [w17]
    shift-right: [w10] -> _
    shift-left: _ -> [w15]
    shift-right: [w20] -> _
    shift-left: _ -> [w18]
    shift-right: [w11] -> _
    tunnel: w5 -> [w9]
    tunnel: w3 -> [w7]
    i -> [w12]
    stop <- w19 continue-if-true
    n4 = case shown="\"Choose Setup file\"" w17 {
      tunnel: w15 -> [w31 w41 w66 w76 _ w124 w152 w161 w182 w192 w204 w218 w249 w276 w299 w422 w444 w470 w495 w521 w575 w589 w626 w936 w1007 w1062 w1087 w1107 w1233 w1288 w1318 w1618 w1634 w1646 w1678 w1708 w1780 w1818 w1828 w1897 w1920 w1953 w1994 w2053 w2079 w2288 w2300 w2325 w2410 w2554 w2588 w2603 w2628 w2673 w2691 w2734 w2833 w2867 w3277 w3320 w3333 w3343]
      tunnel: [w31 w41 w66 w76 w109 w124 w152 w161 w182 w192 w204 w218 w249 w276 w297 w422 w444 w470 w495 w521 w575 w589 w626 w936 w1007 w1062 w1087 w1107 w1233 w1288 w1316 w1618 w1634 w1646 w1678 w1708 w1780 w1818 w1828 w1897 w1920 w1953 w1994 w2053 w2077 w2288 w2300 w2323 w2403 w2554 w2588 w2603 w2628 w2673 w2691 w2734 w2833 w2867 w3277 w3320 w3333 w3343] -> w20
      tunnel: ["Initialise" w34 w61 w69 "Check Results file array" ("t") "Template Required?" "Read Template File" "What file to start with" w173 w188 "Which file to read next" "Which file to read next" "Which file to read next" w272 w294 w413 "What is present?" "Ordinate Selector Type" w492 "Which rows are Non-Blank?" w568 "Create Selectors" w615 "Re Plot Data?" w1003 "Prepare Filter2 strings" "Plot Data" w1104 "Add Axis names" "Analyse Plot Space" w1319 "What to do next?" "What to do next?" ("t") "What to do next?" ("t") w1660 w1701 w1756 w1814 w1826 w1892 w1916 "Ordinate Selector Type" w1993 "Initialise" w2080 w2279 "Create Selectors" w2326 w2411 w2552 w2586 w2593 w2613 "Create Selectors" w2688 w2737 w2817 w2872 "Initialise" ("t") w3289 "Time to save setup?" ""] -> w10
      tunnel: [FALSE TRUE TRUE TRUE ("T button?") TRUE TRUE TRUE TRUE TRUE TRUE TRUE TRUE TRUE w267 w301 TRUE TRUE TRUE TRUE TRUE TRUE TRUE TRUE TRUE TRUE TRUE TRUE w1105 TRUE TRUE w1320 TRUE TRUE ("OK?") TRUE ("OK?") TRUE TRUE ("OK?") TRUE ("OK?") TRUE ("OK?") TRUE ("OK?") TRUE TRUE TRUE w1992 TRUE w2081 TRUE ("OK?") TRUE ("OK?") w2327 w2412 TRUE TRUE TRUE TRUE TRUE TRUE TRUE TRUE TRUE TRUE TRUE ("OK?") TRUE ("OK?") FALSE] -> w19
      tunnel: w18 -> [w30 w40 w65 w75 _ w123 w151 w163 w181 w191 w203 w217 w248 w275 w300 w418 w443 w471 w496 w522 w574 w587 w621 w938 w997 w1064 w1089 w1106 w1235 w1290 w1317 w1617 w1633 w1645 w1677 w1719 w1779 w1817 w1827 w1896 w1919 w1952 w1991 w2052 w2078 w2287 w2297 w2324 w2409 w2555 w2587 w2602 w2632 w2672 w2690 w2733 w2832 w2866 w3276 w3319 w3332 w3342]
      tunnel: w17 -> [w22 _ _ _ _ _ _ _ _ _ _ _ _ _ _ _ _ _ _ _ _ _ _ _ _ _ _ _ _ _ _ _ _ _ _ _ _ _ _ _ _ _ _ _ _ _ _ _ _ _ _ _ _ _ _ _ _ _ _ _ _ _]
      tunnel: path "Dont bother with template file" ("Template File") -> [_ _ _ _ _ w117 _ _ _ _ _ _ _ _ _ _ _ _ _ _ _ _ _ _ _ _ _ _ _ _ _ _ _ _ _ _ _ _ _ _ _ _ _ _ _ _ _ _ _ _ _ _ _ _ _ _ _ _ w3271 _ _ w3341]
      tunnel: [w21 w39 w64 w77 w109 w122 w150 w162 w179 w189 w201 w215 w246 w274 w296 w406 w442 w472 w494 w520 w566 w588 w619 w935 w999 w1055 w1082 w1103 w1227 w1283 w1312 w1614 w1635 w1647 w1676 w1709 w1781 w1819 w1829 w1895 w1918 w1951 w1990 w2051 w2071 w2289 w2305 w2317 w2406 w2564 w2589 w2604 w2629 w2674 w2692 w2738 w2834 w2873 w3278 w3321 w3334 w3344] -> w14
      tunnel: w13 -> [w21 w39 w64 w77 _ w122 w150 w162 w179 w189 w201 w215 w246 w274 w295 w406 w442 w472 w494 w520 w566 w588 w619 w935 w999 w1055 w1082 w1103 w1227 w1283 w1311 w1614 w1635 w1647 w1676 w1709 w1781 w1819 w1829 w1895 w1918 w1951 w1990 w2051 w2070 w2289 w2305 w2320 w2405 w2564 w2589 w2604 w2629 w2674 w2692 w2738 w2834 w2873 w3278 w3321 w3334 w3344]
      tunnel: w12 -> [_ _ _ _ _ _ _ _ _ _ _ _ _ _ _ _ _ _ _ _ _ _ _ _ _ _ _ w1102 _ _ _ _ _ _ _ _ _ _ w1825 _ _ _ _ _ _ _ _ _ _ _ _ _ _ _ _ _ _ _ _ _ _ _]
      tunnel: [w30 w40 w65 w75 string[][] [] w123 w151 w163 w181 w191 w203 w217 w248 w275 w298 w418 w443 w471 w496 w522 w574 w587 w621 w938 w997 w1064 w1089 w1106 w1235 w1290 w1315 w1617 w1633 w1645 w1677 w1719 w1779 w1817 w1827 w1896 w1919 w1952 w1991 w2052 w2076 w2287 w2297 w2322 w2402 w2555 w2587 w2602 w2632 w2672 w2690 w2733 w2832 w2866 w3276 w3319 w3332 w3342] -> w11
      tunnel: w9 -> [_ _ _ _ _ _ _ _ _ _ _ _ _ _ _ _ _ _ _ _ _ _ _ _ _ _ _ _ _ _ _ _ _ _ _ _ _ _ _ _ w1914 _ w1989 _ _ _ _ _ _ _ _ _ _ _ w2687 w2732 _ w2865 _ _ _ _]
      tunnel: w7 -> [_ w32 _ _ _ _ _ _ _ _ _ _ _ _ _ _ _ _ _ _ _ _ _ _ _ _ _ _ _ _ _ _ _ _ _ _ _ _ _ _ _ _ _ _ _ _ _ _ _ _ _ _ _ _ _ _ _ _ _ w3296 _ _]
      frame "No Match", Default {
        n5 = Current VI's Path() -> (path=w23:path)
        n6 = Format Into String(format string="The Case\"%s\" was not Matched\nin VI named\n'%s\"" ("Format String"), w22, w23) -> (resulting string=w26:string)  [unwired: 2 in, 1 out]
        n7 = One Button Dialog(message=w26, button name ("OK")="STOP") -> (true=w24:bool)
        n8 = Stop(stop? (T)=w24) -> ()
      }
      frame "First Run?" {
        w33 = FALSE ("Save Plot data")
        n9 = global write "Results_plotter_Global.vi" "Setup Filename"(w32) -> ()
        n10 = call "Run_EnFlo_Hub.vi"() -> ()  [unwired: 1 in, 7 out]
        n11 = while {
          shift-right: [1] -> _
          shift-left: _ -> [w44]
          tunnel: [w44] -> w36
          stop <- FALSE continue-if-true
        }
        n12 = local write "Edit Template File"(w33) -> ()
        n13 = local write "Save Plot data"(w33) -> ()
        n14 = local write "Delete Plotted data from file"(w33) -> ()
        n15 = local write "color and symbol"(w33) -> ()
        n16 = local write "Reload Files"(w33) -> ()
        n17 = local write "Save Setup"(w33) -> ()
        n18 = local write "Vector Plot?"(w33) -> ()
        n19 = local write "Load Setup"(w33) -> ()
        n20 = local write "Kill Point"(w33) -> ()
        n21 = local write "Save Data in Rows"(w33) -> ()
        n22 = local write "Post Process Plotted Data"(w33) -> ()
        n23 = local write "Add /Edit metadata"(w33) -> ()
        n24 = local write "Update"(w33) -> ()
        n25 = local write "Add results file"(w33) -> ()
        n26 = local write "Process Point"(w33) -> ()
        n27 = local write "stop"(w33) -> ()
        n28 = local write "Save Averaged rows"(w33) -> ()
        n29 = Equal To 0?(x=w36) -> (x = 0?=w35:bool)
        n30 = Select(t="Load setup", s=w35, f="Initialise") -> (s? t:f=w34:string)
      }
      frame "Choose Setup file" {
        w47 = Setup_Filetype."Results File Plotter Setups" ("Setup File Type")
        n31 = call "Setup_Filepath.vi"("Setup File Type"=w47, "Filename in"="Test") -> ("Directory"=w49:path)  [unwired: 1 out]
        n32 = call "Last_Years_Setups.vi"("Setup File Type"=w47) -> ("Directory"=w48:path)
        n33 = local write "Load Setup"(FALSE ("Save Setup")) -> ()
        n34 = call "List_files_in_order_of_age.vi"("Folder"=w48) -> ("file names"=w51:string[])  [unwired: 1 in]
        n35 = call "List_files_in_order_of_age.vi"("Folder"=w49) -> ("file names"=w50:string[])  [unwired: 1 in]
        n36 = Build Array (concatenate)(w50, w51) -> (w53:string[])
        n37 = call "Analyse_string_array.vi"("String array"=w53) -> ("Unique strings"=w46:string[])  [unwired: 1 in, 1 out]
        n38 = call "Select_Strings.vi"("Available Ch names"=w46, "Message"="Please Choose a setup file", "Selector mode"=T8."One") -> ("Cancel"=w55:bool, "Selected Channel Names"=w58:string[])  [unwired: 2 in, 2 out]
        n39 = Index Array(array=w58, index=0) -> (element=w56:string)
        n40 = global write "Results_plotter_Global.vi" "Setup Filename"(w56) -> ()
        n41 = Select(t="Time to save setup?", s=w55, f="Load setup") -> (s? t:f=w61:string)
      }
      frame "Load setup" {
        n42 = global read "Results_plotter_Global.vi" "Setup Filename"() -> (w72:string)
        n43 = local write "Tab Control"(T9."Load " ("Tab Control")) -> ()
        n44 = call "Read_Write_Plot_Setup.vi"("Mode"=enum16{"Load", "Save"}."Load", "Setup filename"=w72) -> ("OK?"=w70:bool, "Cluster 2"=w73:T14)  [unwired: 1 in]
        n45 = case shown="True" w70 {
          tunnel: w73 -> [_ w103]
          tunnel: [w80 "Initialise" ("t")] -> w69
          frame False {
            n46 = Two Button Dialog(message="Sorry; that Setup file could not be read", 1:"Oh Just Stop Then!" ("F button name (\"Cancel\")"), 2:"Carry On Without" ("T button name (\"OK\")")) -> (T button?=w78:bool)
            n47 = Select(t="Initialise", s=w78, f="End" ("t")) -> (s? t:f=w80:string)
          }
          frame True {
            n48 = Unbundle By Name(w103) -> ("Result files to read"=w88:path[], "Template"=w86:path, "Transpose"=w93:bool, "Additional X Values"=w94:dbl[], "Additional Y Values"=w95:dbl[], "Ordinate"=w96:u16, "Absisca"=w97:u16, "Filter Array"=w98:u16[], "Output Filename"=w99:path, "Jpg Vi Name"=w100:string, "Intensity Plot?"=w101:bool, "Multi Ordinate?"=w102:bool, "Filter Bins 1"=w92:i32[], "Filter Bins 2"=w91:i32[], "Multi Ordinate"=w90:i32[])  [unwired: 1 out]
            n49 = Index Array(array=w88, index=0) -> (element=w87:path)
            n50 = local write "Choosen Path"(w87) -> ()
            n51 = local write "Result files to read"(w88) -> ()
            n52 = local write "Template"(w86) -> ()
            n53 = local write "Transpose"(w93) -> ()
            n54 = local write "Additional X Values"(w94) -> ()
            n55 = local write "Additional Y Values"(w95) -> ()
            n56 = local write "Ordinate"(w96) -> ()
            n57 = local write "Absisca"(w97) -> ()
            n58 = local write "Filter Array"(w98) -> ()
            n59 = local write "Output Filename"(w99) -> ()
            n60 = local write "Create picture Vi Name"(w100) -> ()
            n61 = local write "Intensity Plot?"(w101) -> ()
            n62 = local write "Multi Ordinate?"(w102) -> ()
            n63 = local write "Filter Bins 1"(w92) -> ()
            n64 = local write "Filter Bins 2"(w91) -> ()
            n65 = local write "Multi Ordinate"(w90) -> ()
          }
        }
      }
      frame "Initialise" {
        w109 = string[] [] ("Channel names")
        n66 = case shown="True" "Empty" {
          frame False {
          }
          frame True {
            n67 = local write "Result files to read"(path[] [] ("Result files to read")) -> ()
            n68 = local write "Empty"(FALSE ("Empty")) -> ()
          }
        }
        n69 = local write "Results files choosen"(path[] [] ("Results file choosen")) -> ()
        n70 = local write "Reload Files"(FALSE ("Reload Files")) -> ()
        "File Index" <- 0
      }
      frame "Check Results file array" {
        n71 = local read "Result files to read"() -> (w121:path[])
        n72 = for {
          shift-right: [w135] -> w119
          shift-left: path[] [] -> [w134]
          tunnel: w121 -> [w133] mode=indexing
          shift-right: [w128] -> _
          shift-left: TRUE -> [w127]
          n73 = Search 1D Array(1D array=w134, element=w133) -> (index of element=w132:i32)  [unwired: 1 out]
          n74 = case shown="False" w127 {
            tunnel: w133 -> [w137 w139]
            tunnel: [w136 w138] -> w130
            frame False {
              n75 = call "Does_file_exist_(simple).vi"("Pathname"=w137) -> ("exists?"=w136:bool)
            }
            frame True {
              n76 = call "Check_Vol_Mounted.vi"("Filename"=w139) -> ("exists?"=w138:bool)  [unwired: 1 out]
            }
          }
          n77 = Less Than 0?(x=w132) -> (x < 0?=w129:bool)
          n78 = And(x=w129, y=w130) -> (x .and. y?=w131:bool)
          n79 = case shown="False" w131 {
            tunnel: w134 -> [w141 w145]
            tunnel: w133 -> [_ w144]
            tunnel: [w141 w143] -> w135
            tunnel: [FALSE w142] -> w128
            tunnel: w127 -> [_ w142]
            frame False {
            }
            frame True {
              n80 = Build Array (concatenate)(w145, w144) -> (w143:path[])
            }
          }
        }
        n81 = Equal?(x="Template", y=w117) -> (x = y?=w116:bool)
        n82 = case shown="True" w116 {
          frame False {
          }
          frame True {
            n83 = local write "Template"(path "") -> ()
          }
        }
        n84 = local write "Result files to read"(w119) -> ()
      }
      frame "Template Required?" {
        n85 = local read "Template"() -> (w149:path)
        n86 = call "Check_Vol_Mounted.vi"("Filename"=w149) -> ("Filename Out"=w148:path, "exists?"=w147:bool)
        n87 = case shown="True" w147 {
          tunnel: w148 -> [_ w157]
          tunnel: [path "" w156] -> w146
          frame False {
          }
          frame True {
            n88 = call "File_checker_and_finder.vi"("Promp if not found"="Please select Template file", "Filename In"=w157) -> ("Filename Out"=w156:path)  [unwired: 1 out]
          }
        }
        n89 = local write "Template"(w146) -> ()
      }
      frame "Read Template File" {
        n90 = local read "Template"() -> (w159:path)
        "Last used Template" <- w159
        n91 = call "Load_Template_Globals.vi"("Channel Names"=w161, "Template-read"=w159) -> ("Valid Template File?"=w160:bool)
        n92 = case shown="True" w160 {
          tunnel: w159 -> [_ w168]
          frame False {
          }
          frame True {
            n93 = global read "Results_plotter_Global.vi" "Tolerances"() -> (w171:string[])
            n94 = call "Read_Write_Template.vi"("Template File"=w168, "Mode"=Global_mode."Read Global", "Data type"="Log Folder Name" ("Variable name")) -> ("Single Value Out"=w166:string)  [unwired: 5 in, 7 out]
            n95 = Fract/Exp String To Number(string=w171) -> (number=→"Tolerances":dbl[])  [unwired: 4 out]
            n96 = call "String_to_Pathname.vi"("Input String"=w166) -> ("path"=w167:path)
            n97 = local write "Job Directory"(w167) -> ()
          }
        }
      }
      frame "What file to start with" {
        n98 = local read "Result files to read"() -> (w178:path[])
        n99 = Array Size(array=w178) -> (size(s)=w177:i32)
        n100 = Greater Than 0?(x=w177) -> (x > 0?=w174:bool)
        n101 = Select(t="Which file to read next", s=w174, f="More files options") -> (s? t:f=w173:string)
      }
      frame "More files options" {
        n102 = call <vilib>:"Three Button Dialog.vi"("Right Button Text (\"Cancel\")"="A entire Folder" ("F button name (\"Cancel\")"), "Center Button Text (\"No\")"="Selection of files in Folder" ("T button name (\"OK\")"), "Left Button Text (\"Yes\")"="A Data File" ("T button name (\"OK\")"), "message"="Where is the data to come from?") -> ("Which Button?"=w187:T15)  [unwired: 1 in, 6 out]
        n103 = case shown="\"Left Button\", Default" w187 {
          tunnel: ["Choose Results File" "Selection of files in Folder" "Choose a Folder"] -> w188
          frame "Left Button", Default {
          }
          frame "Center Button" {
          }
          frame "Right Button" {
          }
        }
      }
      frame "Choose Results File" {
        (unwired) T16."existing file" ("select mode (2)")
        n104 = local read "Choosen Path"() -> (w196:path)
        n105 = File Dialog(7:"Please Choose a Results File" ("Promp if not found"), 11:w196) -> (1:w198:bool, 3:w197:path)  [unwired: 1 in, 6 out]
        "Choosen Path" <- w197
        n106 = case shown="False" w198 {
          tunnel: w197 -> [w205 _]
          frame False {
            n107 = local read "Result files to read"() -> (w206:path[])
            n108 = Build Array (concatenate)(w206, w205) -> (w207:path[])
            n109 = local write "Result files to read"(w207) -> ()
          }
          frame True {
          }
        }
      }
      frame "Choose a Folder" {
        n110 = local read "Choosen Path"() -> (w209:path)
        n111 = File Dialog(7:"Please Choose the folder that contains the Results files to be plotted" ("prompt"), 11:w209) -> (3:w208:path)  [unwired: 1 in, 7 out]
        n112 = local write "Choosen Path"(w208) -> ()
        n113 = call "Get_folder_and_filenames.vi"("file path (dialog if empty)"=w208) -> ("Files"=w210:path[])  [unwired: 1 out]
        n114 = for {
          shift-right: [w229] -> w211
          shift-left: "Result files to read" -> [w228]
          tunnel: w210 -> [w226] mode=indexing
          n115 = Search 1D Array(1D array=w228, element=w226) -> (index of element=w227:i32)  [unwired: 1 out]
          n116 = Strip Path(path=w226) -> (name=w225:string)  [unwired: 1 out]
          n117 = Less Than 0?(x=w227) -> (x < 0?=w224:bool)
          n118 = call "Add_filename_suffix.vi"("Filename"=w225) -> ("Original Suffix"=w222:string)  [unwired: 1 in, 3 out]
          n119 = call "Match_Pat_Case_In.vi"("String to match"=".jpg" ("x"), "String"=w222) -> ("offset past match"=w220:i32)  [unwired: 1 in, 3 out]
          n120 = Less Than 0?(x=w220) -> (x < 0?=w219:bool)
          n121 = And(x=w224, y=w219) -> (x .and. y?=w223:bool)
          n122 = case shown="True" w223 {
            tunnel: w228 -> [w230 w233]
            tunnel: w226 -> [_ w232]
            tunnel: [w230 w231] -> w229
            frame False {
            }
            frame True {
              n123 = Build Array (concatenate)(w233, w232) -> (w231:path[])
            }
          }
        }
        n124 = local write "Result files to read"(w211) -> ()
      }
      frame "Selection of files in Folder" {
        n125 = local read "Choosen Path"() -> (w235:path)
        n126 = local read "Result files to read"() -> (w238:path[])
        n127 = File Dialog(7:"Please Choose the folder that contains the Results files to be plotted" ("prompt"), 11:w235) -> (3:w234:path)  [unwired: 1 in, 7 out]
        n128 = call "Get_folder_and_filenames.vi"("file path (dialog if empty)"=w234) -> ("Files"=w240:path[])  [unwired: 1 out]
        n129 = local write "Choosen Path"(w234) -> ()
        n130 = for {
          tunnel: w240 -> [w263] mode=indexing
          tunnel: [w262] -> w243 mode=indexing
          n131 = Strip Path(path=w263) -> (name=w262:string)  [unwired: 1 out]
        }
        n132 = call "Select_Strings.vi"("Available Ch names"=w243, "Message"="Please select the desired data files", "Selector mode"=T8."Zero or more") -> ("Ch Indicies Choosen"=w241:i32[])  [unwired: 2 in, 3 out]
        n133 = for {
          tunnel: w241 -> [w261] mode=indexing
          tunnel: w240 -> [w260]
          tunnel: [w259] -> w236 mode=indexing
          n134 = Index Array(array=w260, index=w261) -> (element=w259:path)
        }
        n135 = for {
          shift-right: [w254] -> w237
          shift-left: w238 -> [w253]
          tunnel: w236 -> [w252] mode=indexing
          n136 = Search 1D Array(1D array=w253, element=w252) -> (index of element=w251:i32)  [unwired: 1 out]
          n137 = Less Than 0?(x=w251) -> (x < 0?=w250:bool)
          n138 = case shown="True" w250 {
            tunnel: w253 -> [w255 w258]
            tunnel: w252 -> [_ w257]
            tunnel: [w255 w256] -> w254
            frame False {
            }
            frame True {
              n139 = Build Array (concatenate)(w258, w257) -> (w256:path[])
            }
          }
        }
        n140 = local write "Result files to read"(w237) -> ()
      }
      frame "Which file to read next" {
        n141 = local read "Result files to read"() -> (w273:path[])
        n142 = local read "File Index"() -> (w270:i32)
        n143 = Array Size(array=w273) -> (size(s)=w271:i32)
        n144 = Equal?(x=w271, y=w270) -> (x = y?=w269:bool)
        n145 = case shown="False" w269 {
          tunnel: w273 -> [w279 _]
          tunnel: [w280 "Load Selectors"] -> w272
          tunnel: w270 -> [w278 w292]
          tunnel: [w277 w292] -> w265
          frame False {
            n146 = Index Array(array=w279, index=w278) -> (element=w281:path)
            n147 = Search 1D Array(1D array="Results files choosen", element=w281) -> (index of element=w283:i32)  [unwired: 1 out]
            n148 = call "Add_filename_suffix.vi"() -> ()  [unwired: 2 in, 4 out]
            n149 = case shown="-1" w283 {
              tunnel: "Results files choosen" -> [_ w291]
              tunnel: w281 -> [w287 w290]
              tunnel: ["Which file to read next" "Load Data"] -> w280
              frame 0, Default {
                n150 = Format Into String(format string="The filename\n \"%s\"\n has already been chosen" ("Format String"), w287) -> (resulting string=w285:string)  [unwired: 2 in, 1 out]
                n151 = One Button Dialog(message=w285) -> ()  [unwired: 2 out]
              }
              frame -1 {
                n152 = Build Array (concatenate)(w291, w290) -> (w289:path[])
                n153 = local write "Results files choosen"(w289) -> ()
              }
            }
            n154 = local write "Results file"(w281) -> ()
            n155 = Increment(x=w278) -> (x+1=w277:i32)
          }
          frame True {
          }
        }
        n156 = local read "stop"() -> (w268:bool)
        n157 = Decrement(x=w265) -> (x-1=w264:i32)
        n158 = Build Array(w264) -> (w266:i32[])
        n159 = Not(x=w268) -> (.not. x?=w267:bool)
        n160 = local write "File Index"(w265) -> ()
        n161 = property on="Result files to read" class="Arr (strict)"("Index Values"=w266) -> ()  [unwired: 2 in, 2 out]
      }
      frame "Load Data" {
        n162 = stacked-sequence {
          seq-local: [w307 _] -> [_ w367]
          seq-local: [w306 _] -> [_ w372]
          seq-local: [w305 _] -> [_ w371]
          seq-local: [w303 _] -> [_ w370]
          tunnel: [TRUE _] -> w301
          tunnel: w300 -> [w321 w373]
          tunnel: w299 -> [w320 _]
          tunnel: [w319 _] -> w298
          tunnel: [w318 _] -> w297
          tunnel: [w317 _] -> w296
          tunnel: w295 -> [w316 _]
          tunnel: ["Which file to read next" _] -> w294
          frame #0 {
            w302 = TRUE  # Delete First Rows?
            w310 = TRUE  # Add Extra Channels?
            n163 = local read "Template"() -> (w314:path)
            n164 = call "Read_Data_file.vi"("Results file"="Results file", "Delete First Rows?"=w302, "Add Extra Channels?"=w310, "Template File"=w314, "Desired File Types"="File Types to Read") -> ("Row numbers"=w305:i32[], "Template File Out"=w311:path, "Filetype"=w306:string, "Results file Out"=w307:path, "Ch names Out"=w312:string[], "Channel Values Out"=w308:string[][])  [unwired: 1 in, 8 out]
            n165 = local write "Template"(w311) -> ()
            n166 = Array Size(array=w312) -> (size(s)=w313:i32)
            n167 = Greater Than 0?(x=w313) -> (x > 0?=w303:bool)
            n168 = case shown="True" w303 {
              tunnel: w321 -> [w323 w337]
              tunnel: w320 -> [w325 w332]
              tunnel: w308 -> [_ w330]
              tunnel: [w323 w328] -> w319
              tunnel: [w325 w326] -> w318
              tunnel: [w324 w327] -> w317
              tunnel: w316 -> [w324 _]
              tunnel: w312 -> [_ w331]
              frame False {
              }
              frame True {
                n169 = for {
                  tunnel: w330 -> [w339] mode=indexing
                  tunnel: [w338] -> w329 mode=indexing
                  n170 = for {
                    tunnel: w339 -> [w341] mode=indexing
                    tunnel: [w340] -> w338 mode=indexing
                    n171 = call "Fast_string_Replace.vi"("Replace match with:"="[", "Input String"=w341, "regular expression"="(") -> ("Output String"=w342:string)  [unwired: 2 out]
                    n172 = call "Fast_string_Replace.vi"("Replace match with:"="]", "Input String"=w342, "regular expression"=")") -> ("Output String"=w340:string)  [unwired: 2 out]
                  }
                }
                n173 = call "Merge_channel_names.vi"("Preferred Channel array"=w332, "Channel array"=w331) -> ("Merged Channels"=w326:string[], "Preferred Channels Changed?"=w334:bool, "Channel Array Changed?"=w335:bool)
                n174 = for {
                  tunnel: w326 -> [w364] mode=indexing
                  tunnel: [w361] -> w327 mode=indexing
                  n175 = call "Fast_string_Replace.vi"("Replace match with:"=" ", "Input String"=w364, "regular expression"=":") -> ("Output String"=w360:string)  [unwired: 2 out]
                  n176 = call "Fast_string_Replace.vi"("Replace match with:"=" ", "Input String"=w360, "regular expression"="  ") -> ("Output String"=w359:string)  [unwired: 2 out]
                  n177 = call <vilib>:"Trim Whitespace.vi"("string"=w359) -> ("trimmed string"=w361:string)  [unwired: 1 in]
                }
                n178 = case shown="True" w334 {
                  tunnel: w337 -> [w352 w354]
                  tunnel: w332 -> [_ w356]
                  tunnel: [w352 w353] -> w333
                  tunnel: w326 -> [_ w355]
                  frame False {
                  }
                  frame True {
                    n179 = call "Merge_2D_values.vi"("Values In"=w354, "Present Channels"=w356, "Desired Channels"=w355) -> ("Values Out"=w353:string[][])
                  }
                }
                n180 = case shown="True" w335 {
                  tunnel: [w347 w351] -> w336
                  tunnel: w331 -> [_ w350]
                  tunnel: w329 -> [w347 w349]
                  tunnel: w326 -> [_ w348]
                  frame False {
                  }
                  frame True {
                    n181 = call "Merge_2D_values.vi"("Values In"=w349, "Present Channels"=w350, "Desired Channels"=w348) -> ("Values Out"=w351:string[][])
                  }
                }
                n182 = global write "Results_plotter_Global.vi" "Channel names"(w327) -> ()
                n183 = global write "Results_plotter_Global.vi" "Full Ch Names"(w326) -> ()
                n184 = Build Array (concatenate)(w333, w336) -> (w328:string[][])
                n185 = global write "Results_plotter_Global.vi" "All Data"(w328) -> ()
              }
            }
          }
          frame #1 {
            n186 = local read "File Index"() -> (w369:i32)
            n187 = Decrement(x=w369) -> (x-1=w368:i32)
            n188 = local read "Result files to read"() -> (w366:path[])
            n189 = case shown="True" w370 {
              tunnel: w373 -> [_ w386]
              tunnel: w372 -> [_ w384]
              tunnel: w371 -> [_ w382]
              tunnel: w368 -> [w374 w380]
              tunnel: w367 -> [_ w379]
              tunnel: w366 -> [w376 w381]
              tunnel: [w375 w378] -> w365
              frame False {
                n190 = Delete From Array(array=w376, length=1, index=w374) -> (array with subset deleted=w375:path[])  [unwired: 1 out]
                n191 = local write "File Index"(w374) -> ()
              }
              frame True {
                n192 = Array Size(array=w386) -> (size(s)=w388:i32[])
                n193 = Index Array(array=w388, index=0 ("Index")) -> (element=w385:i32)
                n194 = for {
                  tunnel: w380 -> [w405]
                  tunnel: [w404] -> w390 mode=indexing
                  tunnel: w385 -> [w401]
                  tunnel: w382 -> [w400] mode=indexing
                  i -> [w402]
                  n195 = Add(x=w402, y=w401) -> (x+y=w403:i32)
                  n196 = Build Array(w405, w400, w403) -> (w404:i32[])
                }
                n197 = case shown="1, Default" w380 {
                  tunnel: w390 -> [w393 w398]
                  tunnel: [w393 w397] -> w389
                  tunnel: w384 -> [w392 w396]
                  tunnel: [w391 w394] -> w383
                  frame 0 {
                    n198 = Build Array(w392) -> (w391:string[])
                  }
                  frame 1, Default {
                    n199 = global read "Results_plotter_Global.vi" "Row Reference"() -> (w399:i32[][])
                    n200 = local read "Filetype"() -> (w395:string[])
                    n201 = Build Array (concatenate)(w395, w396) -> (w394:string[])
                    n202 = Build Array (concatenate)(w399, w398) -> (w397:i32[][])
                  }
                }
                "Filetype" <- w383
                n203 = Replace Array Subset(array=w381, new element=w379, index=w380) -> (w378:path[])
                n204 = global write "Results_plotter_Global.vi" "Row Reference"(w389) -> ()
              }
            }
            n205 = local write "Result files to read"(w365) -> ()
          }
        }
      }
      frame "Load Selectors" {
        n206 = while {
          shift-right: [w426] -> w411
          shift-left: _ -> [w428]
          tunnel: [w428] -> w410
          tunnel: w406 -> [w426]
          stop <- FALSE continue-if-true
        }
        n207 = Array Size(array=w418) -> (size(s)=w417:i32[])
        n208 = local read "Tolerances"() -> (w414:dbl[])
        n209 = Index Array(array=w417, index=0 ("Index")) -> (element=→"nRows":i32)
        n210 = Equal?(x=w411, y=w410) -> (x = y?=w409:bool)
        n211 = Build Array (concatenate)("Don't Filter" ("Input Element"), w406) -> (w423:string[])
        n212 = Array Size(array=w406) -> (size(s)=w420:i32)
        n213 = Array Size(array=w414) -> (size(s)=w419:i32)
        n214 = property on="Multi Ordinate" class="LstBox (strict)"("Item Names"=w406) -> ()  [unwired: 2 in, 2 out]
        n215 = property on="Z Ch Name" class="Ring (strict)"("Strings []"=w406) -> ()  [unwired: 2 in, 2 out]
        n216 = property on="Y Ch Name" class="Ring (strict)"("Strings []"=w406) -> ()  [unwired: 2 in, 2 out]
        n217 = property on="X Ch Name" class="Ring (strict)"("Strings []"=w406) -> ()  [unwired: 2 in, 2 out]
        n218 = property on="X Axis" class="Ring (strict)"("Strings []"=w406) -> ()  [unwired: 2 in, 2 out]
        n219 = property on="Ordinate" class="Ring (strict)"("Strings []"=w406) -> ()  [unwired: 2 in, 2 out]
        n220 = property on="Filter on column 1:" class="Ring (strict)"("Strings []"=w423) -> ()  [unwired: 2 in, 2 out]
        n221 = Not Equal?(x=w420, y=w419) -> (x != y?=w421:bool)
        n222 = case shown="True" w421 {
          tunnel: w420 -> [_ w435]
          tunnel: w419 -> [_ w434]
          tunnel: w414 -> [_ w431]
          frame False {
          }
          frame True {
            n223 = Subtract(x=w435, y=w434) -> (x-y=w433:i32)
            n224 = Initialize Array(1.0 ("Element Data"), w433) -> (w430:dbl[])
            n225 = Build Array (concatenate)(w431, w430) -> (w429:dbl[])
            n226 = local write "Tolerances"(w429) -> ()
          }
        }
        n227 = global write "Results_plotter_Global.vi" "First Loop"(TRUE) -> ()
        n228 = Select(t="What is present?", s=w409, f="Set Axis Channels") -> (s? t:f=w413:string)
      }
      frame "Set Axis Channels" {
        n229 = Array Size(array=w442) -> (size(s)=w441:i32)
        n230 = Build Array("X" ("regular expression"), "Y" ("regular expression"), "Z" ("regular expression")) -> (w436:string[])
        n231 = Decrement(x=w441) -> (x-1=w440:i32)
        n232 = for {
          tunnel: w442 -> [w454]
          tunnel: w440 -> [w453]
          tunnel: w436 -> [w452] mode=indexing
          i -> [w448]
          n233 = while {
            tunnel: w454 -> [w468] mode=indexing
            tunnel: w453 -> [w467]
            tunnel: w452 -> [w465]
            tunnel: [w458] -> w451
            tunnel: [w463] -> w450
            i -> [w463]
            stop <- w466 continue-if-true
            n234 = call "Match_Pat_Case_In.vi"("String to match"=w465, "String"=w468) -> ("offset past match"=w462:i32)  [unwired: 1 in, 3 out]
            n235 = In Range and Coerce(upper limit=4, x=w462, lower limit=0) -> (In Range?=w459:bool)  [unwired: 1 out]
            n236 = Less?(x=w463, y=w467) -> (x < y?=w464:bool)
            n237 = Not(x=w459) -> (.not. x?=w458:bool)
            n238 = And(x=w458, y=w464) -> (x .and. y?=w466:bool)
          }
          n239 = Select(t=0, s=w451, f=w450) -> (s? t:f=w447:i32)
          n240 = case shown="1" w448 {
            tunnel: w447 -> [w455 w456 w457]
            frame 0, Default {
              n241 = local write "X Ch Name"(w455) -> ()
            }
            frame 1 {
              n242 = local write "Y Ch Name"(w456) -> ()
            }
            frame 2 {
              n243 = local write "Z Ch Name"(w457) -> ()
            }
          }
        }
      }
      frame "What is present?" {
        n244 = case shown="True" "Show Results Space Analysis" {
          tunnel: w472 -> [_ w476]
          tunnel: w471 -> [_ w475]
          frame False {
          }
          frame True {
            n245 = stacked-sequence {
              tunnel: w476 -> [w480]
              tunnel: w475 -> [w479]
              frame #0 {
                w477 = FALSE  # Summarise All
                n246 = call "Summarise.vi"("Channel Names"=w480, "Data"=w479, "Summarise All"=w477) -> ("Summary"=w478:string[][])  [unwired: 2 in]
                n247 = call "Results_Space_Analysis.vi"("Table"=w478) -> ()
              }
            }
          }
        }
      }
      frame "Ordinate Selector Type" {
        n248 = while {
          tunnel: [w499] -> w490
          shift-left: _ -> [w499]
          shift-right: ["Slice mode"] -> w491
          stop <- FALSE continue-if-true
          "Previous slice mode" <- w499
        }
        n249 = Not(x="Multi Ordinate?") -> (.not. x?=w485:bool)
        n250 = property on="Multi Ordinate" class="LstBox (strict)"("Visible"="Multi Ordinate?") -> ()  [unwired: 2 in, 2 out]
        n251 = property on="Ordinate Name" class="Str"("Visible"="Multi Ordinate?") -> ()  [unwired: 2 in, 2 out]
        n252 = property on="Ordinate" class="Ring (strict)"("Visible"=w485) -> ()  [unwired: 2 in, 2 out]
        n253 = property on="First Add label" class="Str"("Visible"=w485) -> ()  [unwired: 2 in, 2 out]
        n254 = property on="2nd Add label" class="Str"("Visible"=w485) -> ()  [unwired: 2 in, 2 out]
        n255 = property on="Additional Y Values" class="Arr (strict)"("Visible"=w485) -> ()  [unwired: 2 in, 2 out]
        n256 = property on="Additional X Values" class="Arr (strict)"("Visible"=w485) -> ()  [unwired: 2 in, 2 out]
        n257 = Not Equal?(x=w491, y=w490) -> (x != y?=w482:bool)
        n258 = local read "Intensity Plot?"() -> (w489:bool)
        n259 = Or(x=w482, y="Update") -> (x .or. y?=w483:bool)
        n260 = global read "Results_plotter_Global.vi" "First Loop"() -> (w486:bool)
        n261 = case shown="False" "Multi Ordinate?" {
          frame False {
            n262 = Build Array("Ordinate") -> (w501:u16[])
            n263 = local write "Multi Ordinate"(w501) -> ()
          }
          frame True {
          }
        }
        n264 = Compound Arithmetic op=AND(invert w486, w483, w489) -> (w488:bool)
        "Slice mode Change?" <- w488
        n265 = Select(t="Change Slice mode", s=w488, f="Which rows are Non-Blank?") -> (s? t:f=w492:string)
      }
      frame "Change Slice mode" {
        n266 = local read "Previous slice mode"() -> (w505:T6)
        n267 = local read "Slice mode"() -> (w519:T6)
        n268 = case shown="\"YX Slice (Plan)\"" w519 {
          tunnel: [w531 w536 w543 w548 w555 w561] -> w518
          tunnel: "Y Ch Name" -> [w529 w536 w543 w549 w554 w559]
          tunnel: "X Ch Name" -> [w531 w535 w542 w547 w555 w560]
          tunnel: [w530 w537 w542 w547 w554 w559] -> w509
          tunnel: "Z Ch Name" -> [w530 w537 w541 w548 w553 w561]
          tunnel: [w529 w535 w541 w549 w553 w560] -> w507
          tunnel: w505 -> [w528 w533 w539 w545 w552 w557]
          tunnel: [w526 w532 w538 w544 w551 w556] -> w504
          frame "XY Slice (Plan)" {
            n269 = Equal?(x=Plot_Slice."YX Slice (Plan)" ("Previous slice mode"), y=w528) -> (x = y?=w526:bool)
          }
          frame "YX Slice (Plan)" {
            n270 = Equal?(x=Plot_Slice."XY Slice (Plan)" ("Previous slice mode"), y=w533) -> (x = y?=w532:bool)
          }
          frame "YZ Slice (Cross)" {
            n271 = Equal?(x=Plot_Slice."ZY Slice (Cross)" ("Previous slice mode"), y=w539) -> (x = y?=w538:bool)
          }
          frame "ZY Slice (Cross)" {
            n272 = Equal?(x=Plot_Slice."YZ Slice (Cross)" ("Previous slice mode"), y=w545) -> (x = y?=w544:bool)
          }
          frame "XZ Slice (Side)" {
            n273 = Equal?(x=Plot_Slice."ZX Slice (Side)" ("Previous slice mode"), y=w552) -> (x = y?=w551:bool)
          }
          frame "ZX Slice (Side)" {
            n274 = Equal?(x=Plot_Slice."XZ Slice (Side)" ("Previous slice mode"), y=w557) -> (x = y?=w556:bool)
          }
        }
        n275 = case shown="True" w504 {
          frame False {
          }
          frame True {
            n276 = local read "Transpose"() -> (w525:bool)
            n277 = Not(x=w525) -> (.not. x?=w524:bool)
            n278 = local write "Transpose"(w524) -> ()
          }
        }
        n279 = local write "Update"(FALSE ("Update")) -> ()
        n280 = Increment(x=w509) -> (x+1=w512:u16)
        n281 = Increment(x=w507) -> (x+1=w511:u16)
        n282 = local read "Filter Array"() -> (w516:u16[])
        n283 = Array Subset(array=w516, index=2 ("Array Index")) -> (w514:u16[])  [unwired: 1 in]
        n284 = Build Array (concatenate)(w512, w511, w514) -> (w513:u16[])
        n285 = local write "Filter Array"(w513) -> ()
        n286 = local write "Absisca"(w518) -> ()
      }
      frame "Which rows are Non-Blank?" {
        n287 = while {
          tunnel: [w578] -> w572
          tunnel: [w579] -> w573
          shift-left: _ -> [w580]
          shift-right: [w581] -> w565
          shift-left: _ -> [w583]
          shift-right: [w582] -> _
          stop <- FALSE continue-if-true
          n288 = local read "Multi Ordinate"() -> (w581:i32[])
          n289 = local read "Absisca"() -> (w582:u16)
          n290 = Equal?(x=w582, y=w583) -> (x = y?=w579:bool)
          n291 = Equal?(x=w581, y=w580) -> (x = y?=w578:bool)
        }
        n292 = global read "Results_plotter_Global.vi" "First Loop"() -> (w567:bool)
        n293 = Compound Arithmetic op=AND(invert w567, w573, w572) -> (w571:bool)
        n294 = Array Size(array=w565) -> (size(s)=w564:i32)
        n295 = Greater?(x=w564, y=1) -> (0:w562:bool)
        n296 = global write "Results_plotter_Global.vi" "Multi Ordinate?"(w562) -> ()
        n297 = Select(t="Create Selectors", s=w571, f="Evaluate Blank Rows") -> (s? t:f=w568:string)
      }
      frame "Evaluate Blank Rows" {
        n298 = local read "Multi Ordinate"() -> (w585:i32[])
        n299 = local read "Absisca"() -> (w586:u16)
        n300 = for {
          tunnel: w587 -> [w593] mode=indexing
          tunnel: w586 -> [w596]
          tunnel: w585 -> [w595]
          tunnel: [w592] -> w584 mode=indexing
          n301 = Index Array(array=w593, index=w596) -> (element=w597:string)
          n302 = call "Convert_to_number.vi"("string"=w597) -> ("Number"=w598:dbl)  [unwired: 1 out]
          n303 = Not A Number/Path/Refnum?(number/path/refnum=w598) -> (NaN/Path/Refnum?=w594:bool)
          n304 = case shown="False" w594 {
            tunnel: w595 -> [w602 _]
            tunnel: w593 -> [w601 _]
            tunnel: [w599 FALSE] -> w592
            frame False {
              n305 = for {
                tunnel: w602 -> [w608] mode=indexing
                tunnel: w601 -> [w606]
                tunnel: [w603] -> w600 mode=indexing
                n306 = Index Array(array=w606, index=w608) -> (element=w607:string)
                n307 = call "Convert_to_number.vi"("string"=w607) -> ("Number"=w605:dbl)  [unwired: 1 out]
                n308 = Not A Number/Path/Refnum?(number/path/refnum=w605) -> (NaN/Path/Refnum?=w604:bool)
                n309 = Not(x=w604) -> (.not. x?=w603:bool)
              }
              n310 = Or Array Elements(Boolean array=w600) -> (logical OR=w599:bool)
            }
            frame True {
            }
          }
        }
        "Non-Blank Rows" <- w584
      }
      frame "Create Selectors" {
        n311 = local read "Non-Blank Rows"() -> (w613:bool[])
        n312 = local read "Tolerances"() -> (w611:dbl[])
        n313 = global read "Results_plotter_Global.vi" "Precision"() -> (w610:string[])
        n314 = Array Size(array=w621) -> (size(s)=w620:i32[])
        n315 = Index Array(array=w620, index=0 ("Index")) -> (element=w623:i32)
        n316 = for {
          tunnel: w621 -> [w639]
          tunnel: "Filter Array" -> [w631] mode=indexing
          shift-right: [w638] -> w612
          shift-left: _ -> [w636]
          tunnel: w623 -> [w637]
          tunnel: [w634] -> w618 mode=indexing
          tunnel: w613 -> [w633]
          tunnel: w611 -> [w632]
          tunnel: w610 -> [w629]
          i -> [w635]
          n317 = Decrement(x=w631) -> (x-1=w628:u16)
          n318 = Index Array(array=w629, index=w628) -> (element=w627:string)
          n319 = Index Array(array=w632, index=w628) -> (element=w630:dbl)
          n320 = case shown="1" w635 {
            tunnel: w639 -> [w652 w688 w729 w770 w811 w854 w895]
            tunnel: w631 -> [w651 w687 w728 w769 w810 w853 w894]
            tunnel: w630 -> [w650 w686 w727 w768 w809 w852 w893]
            tunnel: [w649 w685 w726 w767 w808 w851 w892] -> w638
            tunnel: w637 -> [w647 w684 w725 w766 w807 w850 w891]
            tunnel: w636 -> [_ w683 w724 w765 w806 w849 w890]
            tunnel: w635 -> [w646 w682 w721 w762 w803 w848 w887]
            tunnel: [w642 w677 w720 w761 w802 w843 w886] -> w634
            tunnel: w633 -> [w641 w676 w719 w760 w801 w842 w885]
            tunnel: w627 -> [w640 w675 w718 w759 w800 w841 w884]
            frame 0, Default {
              n321 = case shown="1, Default" w651 {
                tunnel: w652 -> [w658 w668]
                tunnel: w651 -> [w659 w667]
                tunnel: w650 -> [_ w674]
                tunnel: [w654 w671] -> w649
                tunnel: "Filter Bins 1" -> [_ w672]
                tunnel: [string[] [] ("Write Attribute") w673] -> w648
                tunnel: w647 -> [w656 _]
                tunnel: w646 -> [w662 w670]
                tunnel: [i32[] [0] ("Filter Bins Out") w669] -> w644
                tunnel: [TRUE ("Unchanged?") w666] -> w642
                tunnel: w641 -> [_ w665]
                tunnel: w640 -> [_ w664]
                frame 0 {
                  n322 = call "Create_filter_points.vi"("Channel to Filter On"=w659, "Index"=w662, "Ch Values In"=w658) -> ()  [unwired: 4 in, 4 out]
                  n323 = Initialize Array(TRUE, w656) -> (w655:bool[])
                  n324 = Build Array(w655) -> (w654:bool[][])
                }
                frame 1, Default {
                  n325 = call "Create_filter_points.vi"("Non-Blank Rows"=w665, "Precision"=w664, "Channel to Filter On"=w667, "Tolerance"=w674, "Index"=w670, "Filter Bins 1"=w672, "Ch Values In"=w668) -> ("Unchanged?"=w666:bool, "Accept array"=w671:bool[][], "Filter Bins Out"=w669:i32[], "Bin Names"=w673:string[])
                }
              }
              n326 = Equal?(x="Filter Bins 1", y=w644) -> (x = y?=w643:bool)
              n327 = case shown="False" w643 {
                tunnel: w644 -> [w653 _]
                frame False {
                  n328 = local write "Filter Bins 1"(w653) -> ()
                }
                frame True {
                }
              }
              n329 = property on="Filter bins 1" class="LstBox (strict)"("Item Names"=w648) -> ()  [unwired: 2 in, 2 out]
            }
            frame 1 {
              n330 = case shown="0" w687 {
                tunnel: w688 -> [_ w700]
                tunnel: w687 -> [w691 w699]
                tunnel: w686 -> [_ w707]
                tunnel: [w695 w703] -> w685
                tunnel: "Filter Bins 2" -> [_ w705]
                tunnel: [string[] [] ("Write Attribute") w709] -> w681
                tunnel: w684 -> [_ _]
                tunnel: w683 -> [w695 w708]
                tunnel: w682 -> [w694 w706]
                tunnel: [i32[] [0] ("Filter Bins Out") w701] -> w680
                tunnel: [TRUE ("Unchanged?") w698] -> w677
                tunnel: w676 -> [_ w697]
                tunnel: w675 -> [_ w696]
                frame 0 {
                  n331 = call "Create_filter_points.vi"("Channel to Filter On"=w691, "Index"=w694) -> ()  [unwired: 5 in, 4 out]
                }
                frame 1, Default {
                  n332 = call "Create_filter_points.vi"("Non-Blank Rows"=w697, "Precision"=w696, "Channel to Filter On"=w699, "Tolerance"=w707, "Index"=w706, "Filter Bins 1"=w705, "Ch Values In"=w700) -> ("Unchanged?"=w698:bool, "Accept array"=w704:bool[][], "Filter Bins Out"=w701:i32[], "Bin Names"=w709:string[])
                  n333 = for {
                    tunnel: w708 -> [w714]
                    tunnel: w704 -> [w713] mode=indexing
                    shift-right: [w710] -> w703
                    shift-left: bool[][] [] -> [w712]
                    n334 = for {
                      tunnel: w713 -> [w717]
                      tunnel: w714 -> [w716] mode=indexing
                      tunnel: [w715] -> _ mode=indexing
                      tunnel: [w715] -> w711 mode=indexing
                      n335 = And(x=w717, y=w716) -> (x .and. y?=w715:bool[])
                    }
                    n336 = Build Array (concatenate)(w712, w711) -> (w710:bool[][])
                  }
                }
              }
              n337 = Equal?(x="Filter Bins 2", y=w680) -> (x = y?=w678:bool)
              n338 = case shown="False" w678 {
                tunnel: w680 -> [w689 _]
                frame False {
                  n339 = local write "Filter Bins 2"(w689) -> ()
                }
                frame True {
                }
              }
              n340 = property on="Filter Bins 2" class="LstBox (strict)"("Item Names"=w681) -> ()  [unwired: 2 in, 2 out]
            }
            frame 2 {
              n341 = case shown="0" w728 {
                tunnel: w729 -> [_ w739]
                tunnel: w728 -> [w732 w740]
                tunnel: w727 -> [_ w751]
                tunnel: [w735 w752] -> w726
                tunnel: "Filter 3" -> [_ w743]
                tunnel: [string[] [] ("Write Attribute") w754] -> w722
                tunnel: w725 -> [_ _]
                tunnel: w724 -> [w735 w753]
                tunnel: w721 -> [w734 w746]
                tunnel: [TRUE ("Unchanged?") w738] -> w720
                tunnel: w719 -> [_ w737]
                tunnel: w718 -> [_ w736]
                frame 0 {
                  n342 = call "Create_filter_points.vi"("Channel to Filter On"=w732, "Index"=w734) -> ()  [unwired: 5 in, 4 out]
                  n343 = local write "Filter 3"(0) -> ()
                }
                frame 1, Default {
                  n344 = Build Array(w743) -> (w750:u16[])
                  n345 = call "Create_filter_points.vi"("Non-Blank Rows"=w737, "Precision"=w736, "Channel to Filter On"=w740, "Tolerance"=w751, "Index"=w746, "Filter Bins 1"=w750, "Ch Values In"=w739) -> ("Unchanged?"=w738:bool, "Accept array"=w748:bool[][], "Filter Bins Out"=w744:i32[], "Bin Names"=w754:string[])
                  n346 = Index Array(array=w744, index=0 ("Index")) -> (element=w741:i32)
                  n347 = Index Array(array=w748, index (row)=0 ("Index")) -> (element=w747:bool[])  [unwired: 1 in]
                  n348 = Equal?(x=w743, y=w741) -> (x = y?=w742:bool)
                  n349 = case shown="True" w742 {
                    tunnel: w741 -> [w755 _]
                    frame False {
                      n350 = local write "Filter 3"(w755) -> ()
                    }
                    frame True {
                    }
                  }
                  n351 = for {
                    tunnel: w747 -> [w758]
                    tunnel: w753 -> [w757] mode=indexing
                    tunnel: [w756] -> w752 mode=indexing
                    n352 = And(x=w758, y=w757) -> (x .and. y?=w756:bool[])
                  }
                }
              }
              n353 = property on="Filter 3" class="Ring (strict)"("Strings []"=w722) -> ()  [unwired: 2 in, 2 out]
            }
            frame 3 {
              n354 = case shown="1, Default" w769 {
                tunnel: w770 -> [_ w781]
                tunnel: w769 -> [w773 w780]
                tunnel: w768 -> [_ w792]
                tunnel: [w776 w793] -> w767
                tunnel: "Filter 4" -> [_ w784]
                tunnel: [string[] [] ("Write Attribute") w795] -> w763
                tunnel: w766 -> [_ _]
                tunnel: w765 -> [w776 w794]
                tunnel: w762 -> [w775 w787]
                tunnel: [TRUE ("Unchanged?") w779] -> w761
                tunnel: w760 -> [_ w778]
                tunnel: w759 -> [_ w777]
                frame 0 {
                  n355 = call "Create_filter_points.vi"("Channel to Filter On"=w773, "Index"=w775) -> ()  [unwired: 5 in, 4 out]
                  n356 = local write "Filter 4"(0) -> ()
                }
                frame 1, Default {
                  n357 = Build Array(w784) -> (w791:u16[])
                  n358 = call "Create_filter_points.vi"("Non-Blank Rows"=w778, "Precision"=w777, "Channel to Filter On"=w780, "Tolerance"=w792, "Index"=w787, "Filter Bins 1"=w791, "Ch Values In"=w781) -> ("Unchanged?"=w779:bool, "Accept array"=w789:bool[][], "Filter Bins Out"=w785:i32[], "Bin Names"=w795:string[])
                  n359 = Index Array(array=w785, index=0 ("Index")) -> (element=w783:i32)
                  n360 = Equal?(x=w784, y=w783) -> (x = y?=w782:bool)
                  n361 = Index Array(array=w789, index (row)=0 ("Index")) -> (element=w788:bool[])  [unwired: 1 in]
                  n362 = case shown="False" w782 {
                    tunnel: w783 -> [w796 _]
                    frame False {
                      n363 = local write "Filter 4"(w796) -> ()
                    }
                    frame True {
                    }
                  }
                  n364 = for {
                    tunnel: w788 -> [w799]
                    tunnel: w794 -> [w798] mode=indexing
                    tunnel: [w797] -> w793 mode=indexing
                    n365 = And(x=w799, y=w798) -> (x .and. y?=w797:bool[])
                  }
                }
              }
              n366 = property on="Filter 4" class="Ring (strict)"("Strings []"=w763) -> ()  [unwired: 2 in, 2 out]
            }
            frame 4 {
              n367 = case shown="1, Default" w810 {
                tunnel: w811 -> [_ w822]
                tunnel: w810 -> [w814 w821]
                tunnel: w809 -> [_ w833]
                tunnel: [w817 w834] -> w808
                tunnel: "Filter 5" -> [_ w824]
                tunnel: [string[] [] ("Write Attribute") w836] -> w804
                tunnel: w807 -> [_ _]
                tunnel: w806 -> [w817 w835]
                tunnel: w803 -> [w816 w828]
                tunnel: [TRUE ("Unchanged?") w820] -> w802
                tunnel: w801 -> [_ w819]
                tunnel: w800 -> [_ w818]
                frame 0 {
                  n368 = call "Create_filter_points.vi"("Channel to Filter On"=w814, "Index"=w816) -> ()  [unwired: 5 in, 4 out]
                  n369 = local write "Filter 5"(0) -> ()
                }
                frame 1, Default {
                  n370 = Build Array(w824) -> (w832:u16[])
                  n371 = call "Create_filter_points.vi"("Non-Blank Rows"=w819, "Precision"=w818, "Channel to Filter On"=w821, "Tolerance"=w833, "Index"=w828, "Filter Bins 1"=w832, "Ch Values In"=w822) -> ("Unchanged?"=w820:bool, "Accept array"=w830:bool[][], "Filter Bins Out"=w826:i32[], "Bin Names"=w836:string[])
                  n372 = Index Array(array=w826, index=0 ("Index")) -> (element=w825:i32)
                  n373 = Equal?(x=w824, y=w825) -> (x = y?=w823:bool)
                  n374 = Index Array(array=w830, index (row)=0 ("Index")) -> (element=w829:bool[])  [unwired: 1 in]
                  n375 = case shown="False" w823 {
                    tunnel: w825 -> [w837 _]
                    frame False {
                      n376 = local write "Filter 5"(w837) -> ()
                    }
                    frame True {
                    }
                  }
                  n377 = for {
                    tunnel: w829 -> [w840]
                    tunnel: w835 -> [w839] mode=indexing
                    tunnel: [w838] -> w834 mode=indexing
                    n378 = And(x=w840, y=w839) -> (x .and. y?=w838:bool[])
                  }
                }
              }
              n379 = property on="Filter 5" class="Ring (strict)"("Strings []"=w804) -> ()  [unwired: 2 in, 2 out]
            }
            frame 5 {
              n380 = case shown="1, Default" w853 {
                tunnel: w854 -> [_ w871]
                tunnel: w853 -> [w857 w870]
                tunnel: w852 -> [_ w875]
                tunnel: [w861 w862] -> w851
                tunnel: "Single Series" -> [_ w873]
                tunnel: [string[] [] ("Write Attribute") w877] -> w847
                tunnel: w850 -> [_ _]
                tunnel: w849 -> [w861 w876]
                tunnel: w848 -> [w860 w874]
                tunnel: [i32[] [0] ("Filter Bins Out") w872] -> w846
                tunnel: [TRUE ("Unchanged?") w869] -> w843
                tunnel: w842 -> [_ w868]
                tunnel: w841 -> [_ w867]
                frame 0 {
                  n381 = call "Create_filter_points.vi"("Channel to Filter On"=w857, "Index"=w860) -> ()  [unwired: 5 in, 4 out]
                }
                frame 1, Default {
                  n382 = call "Create_filter_points.vi"("Non-Blank Rows"=w868, "Precision"=w867, "Channel to Filter On"=w870, "Tolerance"=w875, "Index"=w874, "Filter Bins 1"=w873, "Ch Values In"=w871) -> ("Unchanged?"=w869:bool, "Accept array"=w864:bool[][], "Filter Bins Out"=w872:i32[], "Bin Names"=w877:string[])
                  n383 = Index Array(array=w864, index (row)=0 ("Index")) -> (element=w865:bool[])  [unwired: 1 in]
                  n384 = for {
                    shift-right: [w878] -> w863
                    shift-left: w865 -> [w880]
                    tunnel: w864 -> [w879] mode=indexing
                    n385 = Or(x=w879, y=w880) -> (x .or. y?=w878:bool[])
                  }
                  n386 = for {
                    tunnel: w863 -> [w883]
                    tunnel: w876 -> [w882] mode=indexing
                    tunnel: [w881] -> w862 mode=indexing
                    n387 = And(x=w883, y=w882) -> (x .and. y?=w881:bool[])
                  }
                }
              }
              n388 = Equal?(x="Single Series", y=w846) -> (x = y?=w844:bool)
              n389 = case shown="False" w844 {
                tunnel: w846 -> [w855 _]
                frame False {
                  n390 = local write "Single Series"(w855) -> ()
                }
                frame True {
                }
              }
              n391 = property on="Single Series" class="LstBox (strict)"("Item Names"=w847) -> ()  [unwired: 2 in, 2 out]
            }
            frame 6 {
              n392 = case shown="1, Default" w894 {
                tunnel: w895 -> [_ w906]
                tunnel: w894 -> [w898 w905]
                tunnel: w893 -> [_ w913]
                tunnel: [w901 w918] -> w892
                tunnel: "Filter 6" -> [_ w908]
                tunnel: [string[] [] ("Write Attribute") w920] -> w888
                tunnel: w891 -> [_ _]
                tunnel: w890 -> [w901 w919]
                tunnel: w887 -> [w900 w912]
                tunnel: [TRUE ("Unchanged?") w904] -> w886
                tunnel: w885 -> [_ w903]
                tunnel: w884 -> [_ w902]
                frame 0 {
                  n393 = call "Create_filter_points.vi"("Channel to Filter On"=w898, "Index"=w900) -> ()  [unwired: 5 in, 4 out]
                  n394 = local write "Filter 6"(0) -> ()
                }
                frame 1, Default {
                  n395 = Build Array(w908) -> (w914:u16[])
                  n396 = call "Create_filter_points.vi"("Non-Blank Rows"=w903, "Precision"=w902, "Channel to Filter On"=w905, "Tolerance"=w913, "Index"=w912, "Filter Bins 1"=w914, "Ch Values In"=w906) -> ("Unchanged?"=w904:bool, "Accept array"=w916:bool[][], "Filter Bins Out"=w910:i32[], "Bin Names"=w920:string[])
                  n397 = Index Array(array=w910, index=0 ("Index")) -> (element=w909:i32)
                  n398 = Equal?(x=w908, y=w909) -> (x = y?=w907:bool)
                  n399 = Index Array(array=w916, index (row)=0 ("Index")) -> (element=w915:bool[])  [unwired: 1 in]
                  n400 = case shown="False" w907 {
                    tunnel: w909 -> [w921 _]
                    frame False {
                      n401 = local write "Filter 6"(w921) -> ()
                    }
                    frame True {
                    }
                  }
                  n402 = for {
                    tunnel: w915 -> [w924]
                    tunnel: w919 -> [w923] mode=indexing
                    tunnel: [w922] -> w918 mode=indexing
                    n403 = And(x=w924, y=w923) -> (x .and. y?=w922:bool[])
                  }
                }
              }
              n404 = property on="Filter 6" class="Ring (strict)"("Strings []"=w888) -> ()  [unwired: 2 in, 2 out]
            }
          }
        }
        "Accept Array" <- w612
        n405 = And Array Elements(Boolean array=w618) -> (logical AND=w617:bool)
        n406 = Select(t="Select all for Filter 2", s=w617, f="Create Selectors") -> (s? t:f=w615:string)
      }
      frame "Select all for Filter 2" {
        n407 = local read "Slice mode Change?"() -> (w934:bool)
        n408 = property on="Filter bins 1" class="LstBox (strict)"() -> ("Item Names"=w930:string[], "Top Row"=w929:i32)  [unwired: 2 in, 2 out]
        n409 = case shown="True" w934 {
          frame False {
          }
          frame True {
            n410 = property on="Filter Bins 2" class="LstBox (strict)"() -> ("Item Names"=w950:string[])  [unwired: 2 in, 2 out]
            n411 = Array Size(array=w950) -> (size(s)=w949:i32)
            n412 = Build Array("Blanks", "Numeric", "Non Numeric", "Non Blanks", "Show All" ("Input Element")) -> (w943:string[])
            n413 = local read "Filter Bins 1"() -> (w952:i32[])
            n414 = while {
              tunnel: w950 -> [w965] mode=indexing
              tunnel: w949 -> [w968]
              shift-right: [w959] -> w941
              shift-left: i32[] [] -> [w960]
              tunnel: w943 -> [w962]
              i -> [w961]
              stop <- w966 stop-if-true
              n415 = String Subset(string=w965, length (rest)=4 ("length (rest)")) -> (substring=w970:string)  [unwired: 1 out]
              n416 = Match Pattern(string=w965, regular expression=" (") -> (before substring=w963:string)  [unwired: 4 out]
              n417 = Search 1D Array(1D array=w962, element=w963) -> (index of element=w958:i32)  [unwired: 1 out]
              n418 = Equal?(x="NOT ", y=w970) -> (x = y?=w957:bool)
              n419 = Equal?(x=w968, y=w961) -> (x = y?=w967:bool)
              n420 = Less Than 0?(x=w958) -> (x < 0?=w956:bool)
              n421 = Or(x=w957, y=w967) -> (x .or. y?=w966:bool)
              n422 = Compound Arithmetic op=AND(w956, invert w957) -> (w955:bool)
              n423 = case shown="False" w955 {
                tunnel: w961 -> [_ w975]
                tunnel: w960 -> [w972 w974]
                tunnel: [w972 w973] -> w959
                frame False {
                }
                frame True {
                  n424 = Build Array (concatenate)(w974, w975) -> (w973:i32[])
                }
              }
            }
            n425 = Array Size(array=w952) -> (size(s)=w954:i32)
            n426 = case shown="1" w954 {
              tunnel: [w976 w979] -> w953
              tunnel: w952 -> [_ w978]
              tunnel: i32[] [1] ("Filter Bins 1") -> [w976 w977]
              frame 0, Default {
              }
              frame 1 {
                n427 = Index Array(array=w978, index=0 ("Index")) -> (element=w981:i32)
                n428 = Greater Than 0?(x=w981) -> (x > 0?=w980:bool)
                n429 = Select(t=w978, s=w980, f=w977) -> (s? t:f=w979:i32[])
              }
            }
            n430 = local write "Filter Bins 1"(w953) -> ()
            n431 = local write "Filter Bins 2"(w941) -> ()
          }
        }
        n432 = Array Size(array=w930) -> (size(s)=w931:i32)
        n433 = Less?(x=w931, y=w929) -> (x < y?=w932:bool)
        n434 = case shown="True" w932 {
          frame False {
          }
          frame True {
            n435 = property on="Filter bins 1" class="LstBox (strict)"("Top Row"=0 ("Active Row:Active Row Number")) -> ()  [unwired: 2 in, 2 out]
          }
        }
        n436 = property on="Filter Bins 2" class="LstBox (strict)"() -> ("Item Names"=w928:string[], "Top Row"=w926:i32)  [unwired: 2 in, 2 out]
        n437 = Array Size(array=w928) -> (size(s)=w927:i32)
        n438 = Less?(x=w927, y=w926) -> (x < y?=w925:bool)
        n439 = case shown="True" w925 {
          frame False {
          }
          frame True {
            n440 = property on="Filter Bins 2" class="LstBox (strict)"("Top Row"=0 ("Active Row:Active Row Number")) -> ()  [unwired: 2 in, 2 out]
          }
        }
      }
      frame "Re Plot Data?" {
        n441 = while {
          tunnel: [w1029] -> w992
          shift-left: _ -> [w1031]
          shift-right: [w1030] -> _
          tunnel: [w1034] -> w998
          shift-left: _ -> [w1032]
          shift-right: [w1033] -> _
          tunnel: [w1038] -> w1000
          shift-left: _ -> [w1037]
          shift-right: [w1036] -> w985
          tunnel: [w1039] -> w1001
          shift-left: _ -> [w1041]
          shift-right: [w1040] -> _
          tunnel: [w1043] -> w1002
          shift-left: _ -> [w1042]
          shift-right: [w1035] -> _
          tunnel: [w1044] -> w1004
          tunnel: [w1045] -> w1005
          shift-left: _ -> [w1046]
          shift-right: [w1047] -> _
          shift-left: _ -> [w1049]
          shift-right: [w1048] -> _
          tunnel: [w1050] -> w986
          shift-left: _ -> [w1051]
          shift-right: [w1052] -> _
          tunnel: [w1027] -> w995
          shift-right: [w1024] -> _
          shift-left: _ -> [w1023]
          tunnel: [w1026] -> w994
          shift-right: [w1022] -> _
          shift-left: _ -> [w1025]
          tunnel: [w1019] -> w993
          shift-right: [w1020] -> _
          shift-left: _ -> [w1021]
          shift-right: [w1017] -> _
          shift-left: _ -> [w1018]
          tunnel: [w1016] -> w988
          stop <- FALSE continue-if-true
          n442 = local read "Ordinate Name"() -> (w1017:string)
          n443 = local read "Additional X Values"() -> (w1024:dbl[])
          n444 = local read "Additional Y Values"() -> (w1022:dbl[])
          n445 = local read "Intensity Plot?"() -> (w1036:bool)
          n446 = local read "color and symbol"() -> (w1020:bool)
          n447 = local read "Accept Array"() -> (w1052:bool[][])
          n448 = local read "No of Contours"() -> (w1033:i32)
          n449 = local read "Point Size"() -> (w1030:i32)
          n450 = local read "Multi Ordinate"() -> (w1047:i32[])
          n451 = local read "Resolution"() -> (w1040:dbl)
          n452 = local read "Transpose"() -> (w1035:bool)
          n453 = local read "Absisca"() -> (w1048:u16)
          n454 = Equal?(x=w1017, y=w1018) -> (x = y?=w1016:bool)
          n455 = Equal?(x=w1035, y=w1042) -> (x = y?=w1043:bool)
          n456 = Equal?(x=w1020, y=w1021) -> (x = y?=w1019:bool)
          n457 = Equal?(x=w1033, y=w1032) -> (x = y?=w1034:bool)
          n458 = Equal?(x=w1030, y=w1031) -> (x = y?=w1029:bool)
          n459 = Equal?(x=w1040, y=w1041) -> (x = y?=w1039:bool)
          n460 = Equal?(x=w1024, y=w1023) -> (x = y?=w1027:bool)
          n461 = Equal?(x=w1022, y=w1025) -> (x = y?=w1026:bool)
          n462 = Equal?(x=w1048, y=w1049) -> (x = y?=w1045:bool)
          n463 = Equal?(x=w1052, y=w1051) -> (x = y?=w1050:bool)
          n464 = Equal?(x=w1036, y=w1037) -> (x = y?=w1038:bool)
          n465 = Equal?(x=w1047, y=w1046) -> (x = y?=w1044:bool)
        }
        n466 = global read "Results_plotter_Global.vi" "First Loop"() -> (w996:bool)
        n467 = while {
          shift-right: [w1015] -> _
          shift-left: _ -> [w1014]
          shift-right: [w1012] -> _
          shift-left: _ -> [w1013]
          tunnel: [w1011] -> w991
          tunnel: [w1010] -> w990
          stop <- FALSE continue-if-true
          n468 = local read "Filter Bins 1"() -> (w1012:i32[])
          n469 = local read "Filter Bins 2"() -> (w1015:i32[])
          n470 = Equal?(x=w1012, y=w1013) -> (x = y?=w1010:bool)
          n471 = Equal?(x=w1015, y=w1014) -> (x = y?=w1011:bool)
        }
        n472 = Not(x=w985) -> (.not. x?=w983:bool)
        n473 = property on="Resolution" class="DigNum (strict)"("Visible"=w985) -> ()  [unwired: 2 in, 2 out]
        n474 = property on="Bkgnd Value" class="DigNum (strict)"("Visible"=w985) -> ()  [unwired: 2 in, 2 out]
        n475 = property on="Intensity Graph" class="IntGraph (strict)"("Visible"=w985) -> ()  [unwired: 2 in, 2 out]
        n476 = property on="XY Plot" class="XYGraph (strict)"("Visible"=w983) -> ()  [unwired: 2 in, 2 out]
        n477 = property on="color and symbol" class="Bool (strict)"("Visible"=w983) -> ()  [unwired: 2 in, 2 out]
        n478 = Compound Arithmetic op=AND(w991, w990) -> (w989:bool)
        n479 = Compound Arithmetic op=AND(w988, w989, w992, w993, w998, w1001, w1002, w1005, w1004, w986, w1000, w995, w994, invert w996) -> (w984:bool)
        n480 = Select(t="What to do next?", s=w984, f="Prepare for Plotting") -> (s? t:f=w1003:string)
      }
      frame "Prepare for Plotting" {
        n481 = local read "Filter Array"() -> (w1061:u16[])
        n482 = local read "Multi Ordinate"() -> (w1056:i32[])
        n483 = Index Array(array=w1061, index=0 ("Index")) -> (element=w1058:u16)
        n484 = Equal To 0?(x=w1058) -> (x = 0?=w1059:bool)
        n485 = for {
          tunnel: w1056 -> [w1067] mode=indexing
          tunnel: [w1066] -> w1054 mode=indexing
          tunnel: w1055 -> [w1065]
          n486 = Index Array(array=w1065, index=w1067) -> (element=w1066:string)
        }
        n487 = case shown="False" w1059 {
          tunnel: w1058 -> [w1073 _]
          tunnel: w1055 -> [w1071 _]
          tunnel: [w1068 string[] []] -> w1053
          frame False {
            n488 = Decrement(x=w1073) -> (x-1=w1072:u16)
            n489 = local read "Filter Bins 1"() -> (w1075:i32[])
            n490 = property on="Filter bins 1" class="LstBox (strict)"() -> ("Item Names"=w1074:string[])  [unwired: 2 in, 2 out]
            n491 = Index Array(array=w1071, index=w1072) -> (element=w1069:string)
            n492 = for {
              tunnel: w1075 -> [w1078] mode=indexing
              tunnel: w1074 -> [w1077]
              tunnel: [w1076] -> w1070 mode=indexing
              n493 = Index Array(array=w1077, index=w1078) -> (element=w1076:string)
            }
            n494 = Build Array (concatenate)(w1069, w1070) -> (w1068:string[])
          }
          frame True {
          }
        }
        n495 = global write "Results_plotter_Global.vi" "Ordinate Strings"(w1054) -> ()
        n496 = global write "Results_plotter_Global.vi" "Filter 1 Strings"(w1053) -> ()
      }
      frame "Prepare Filter2 strings" {
        n497 = local read "Filter Array"() -> (w1086:u16[])
        n498 = Index Array(array=w1086, index=1 ("Index")) -> (element=w1083:u16)
        n499 = Equal To 0?(x=w1083) -> (x = 0?=w1084:bool)
        n500 = case shown="False" w1084 {
          tunnel: w1083 -> [w1095 _]
          tunnel: w1082 -> [w1093 _]
          tunnel: [w1090 string[] []] -> w1080
          frame False {
            n501 = Decrement(x=w1095) -> (x-1=w1094:u16)
            n502 = local read "Filter Bins 2"() -> (w1097:i32[])
            n503 = property on="Filter Bins 2" class="LstBox (strict)"() -> ("Item Names"=w1096:string[])  [unwired: 2 in, 2 out]
            n504 = Index Array(array=w1093, index=w1094) -> (element=w1091:string)
            n505 = for {
              tunnel: w1097 -> [w1100] mode=indexing
              tunnel: w1096 -> [w1099]
              tunnel: [w1098] -> w1092 mode=indexing
              n506 = Index Array(array=w1099, index=w1100) -> (element=w1098:string)
            }
            n507 = Build Array (concatenate)(w1091, w1092) -> (w1090:string[])
          }
          frame True {
          }
        }
        n508 = global write "Results_plotter_Global.vi" "Filter 2 Strings"(w1080) -> ()
      }
      frame "Plot Data" {
        n509 = stacked-sequence {
          seq-local: [w1112 _ _] -> [_ w1184 _]
          seq-local: [w1111 _ _] -> [_ w1183 _]
          tunnel: w1106 -> [_ w1193 _]
          tunnel: [_ TRUE _] -> w1105
          tunnel: [_ _ w1211] -> w1104
          tunnel: w1103 -> [w1113 _ _]
          frame #0 {
            w1108 = T17 {"Upper"=0, "Lower"=0, "St Error"=0}  # Error_bars_index
            w1109 = -1 ("Upper")
            n510 = global read "Results_plotter_Global.vi" "Ordinate Strings"() -> (w1112:string[])
            n511 = Bundle By Name(cluster=w1108, "Upper"=w1109, "Lower"=w1109, "St Error"=w1109) -> (w1110:T17)
            n512 = for {
              tunnel: w1112 -> [w1116] mode=indexing
              tunnel: w1113 -> [w1118]
              tunnel: [w1117] -> w1111 mode=indexing
              tunnel: w1110 -> [w1114]
              n513 = String Length(string=w1116) -> (length=w1115:i32)
              n514 = for {
                tunnel: w1116 -> [w1123]
                tunnel: w1118 -> [w1120] mode=indexing
                shift-right: [w1126] -> w1117
                shift-left: w1114 -> [w1125]
                tunnel: w1115 -> [w1121]
                i -> [w1119]
                n515 = String Subset(string=w1120, length (rest)=w1121) -> (substring=w1122:string)  [unwired: 1 out]
                n516 = Equal?(x=w1122, y=w1123) -> (x = y?=w1124:bool)
                n517 = case shown="True" w1124 {
                  tunnel: [w1131 w1178] -> w1126
                  tunnel: w1119 -> [w1130 _]
                  tunnel: w1125 -> [w1129 w1178]
                  tunnel: w1121 -> [w1128 _]
                  tunnel: w1120 -> [w1127 _]
                  frame True {
                    n518 = stacked-sequence {
                      seq-local: [w1132 _ _] -> [_ w1151 _]
                      seq-local: [_ w1150 _] -> [_ _ w1165]
                      tunnel: [_ _ w1164] -> w1131
                      tunnel: w1130 -> [w1145 w1159 w1173]
                      tunnel: w1129 -> [w1144 _ _]
                      tunnel: w1128 -> [w1143 w1158 w1172]
                      tunnel: w1127 -> [w1142 w1157 w1171]
                      frame #0 {
                        n519 = String Subset(string=w1142, offset (0)=w1143) -> (substring=w1137:string)  [unwired: 1 out]
                        n520 = call <vilib>:"Trim Whitespace.vi"("string"=w1137) -> ("trimmed string"=w1135:string)  [unwired: 1 in]
                        n521 = Equal?(x=w1135, y="Err") -> (x = y?=w1139:bool)
                        n522 = Equal?(x=w1135, y="err") -> (x = y?=w1136:bool)
                        n523 = Equal?(x=w1135, y="St Error") -> (x = y?=w1133:bool)
                        n524 = Compound Arithmetic op=OR(w1139, w1136, w1133) -> (w1138:bool)
                        n525 = case shown="True" w1138 {
                          tunnel: [w1146 w1149] -> w1132
                          tunnel: w1145 -> [w1147 _]
                          tunnel: w1144 -> [w1148 w1149]
                          frame True {
                            n526 = Bundle By Name(cluster=w1148, "St Error"=w1147) -> (w1146:T17)
                          }
                          frame False {
                          }
                        }
                      }
                      frame #1 {
                        n527 = String Subset(string=w1157, offset (0)=w1158) -> (substring=w1156:string)  [unwired: 1 out]
                        n528 = call <vilib>:"Trim Whitespace.vi"("string"=w1156) -> ("trimmed string"=w1155:string)  [unwired: 1 in]
                        n529 = To Lower Case(string=w1155) -> (all lower case string=w1153:string)
                        n530 = Match Pattern(string=w1153, regular expression="upper") -> (offset past match=w1152:i32)  [unwired: 1 in, 3 out]
                        n531 = case shown="Default" w1152 {
                          tunnel: [w1160 w1163] -> w1150
                          tunnel: w1159 -> [w1161 _]
                          tunnel: w1151 -> [w1162 w1163]
                          frame Default {
                            n532 = Bundle By Name(cluster=w1162, "Upper"=w1161) -> (w1160:T17)
                          }
                          frame -1 {
                          }
                        }
                      }
                      frame #2 {
                        n533 = String Subset(string=w1171, offset (0)=w1172) -> (substring=w1170:string)  [unwired: 1 out]
                        n534 = call <vilib>:"Trim Whitespace.vi"("string"=w1170) -> ("trimmed string"=w1169:string)  [unwired: 1 in]
                        n535 = To Lower Case(string=w1169) -> (all lower case string=w1167:string)
                        n536 = Match Pattern(string=w1167, regular expression="lower") -> (offset past match=w1166:i32)  [unwired: 1 in, 3 out]
                        n537 = case shown="Default" w1166 {
                          tunnel: [w1174 w1177] -> w1164
                          tunnel: w1173 -> [w1175 _]
                          tunnel: w1165 -> [w1176 w1177]
                          frame Default {
                            n538 = Bundle By Name(cluster=w1176, "Lower"=w1175) -> (w1174:T17)
                          }
                          frame -1 {
                          }
                        }
                      }
                    }
                  }
                  frame False {
                  }
                }
              }
            }
          }
          frame #1 {
            n539 = global read "Results_plotter_Global.vi" "Filter 1 Strings"() -> (w1179:string[])
            n540 = global read "Results_plotter_Global.vi" "Filter 2 Strings"() -> (w1180:string[])
            n541 = local read "Accept Array"() -> (w1195:bool[][])
            n542 = local read "Multi Ordinate?"() -> (w1189:bool)
            n543 = Select(t=5, s=w1189, f=2 ("y")) -> (s? t:f=w1187:i32)
            n544 = global write "Results_plotter_Global.vi" "Ordinate"("Multi Ordinate") -> ()
            n545 = global write "Results_plotter_Global.vi" "Absisca"("Absisca") -> ()
            n546 = global write "Results_plotter_Global.vi" "Transpose"("Transpose") -> ()
            n547 = while {
              shift-right: [w1198] -> w1192
              shift-left: _ -> [w1199]
              tunnel: "color and symbol" -> [w1200]
              tunnel: w1187 -> [w1196]
              stop <- FALSE continue-if-true
              n548 = case shown="True" w1200 {
                tunnel: w1199 -> [w1207 w1209]
                tunnel: [w1206 w1209] -> w1198
                tunnel: w1196 -> [w1201 _]
                frame True {
                  n549 = Add(x=w1207, y=1) -> (x+y=w1204:i32)
                  n550 = local write "color and symbol"(FALSE ("color and symbol")) -> ()
                  n551 = Greater?(x=w1204, y=w1201) -> (0:w1205:bool)
                  n552 = Select(t=0, s=w1205, f=w1204) -> (s? t:f=w1206:i32)
                }
                frame False {
                }
              }
            }
            n553 = call "Plot_XY_data.vi"("Channel Values"=w1193, "Ordinate Strings"=w1184, "Swap color and symbol"=w1192, "Error bar ch index"=w1183, "Accept Array"=w1195, "Filter 1 Strings"=w1179, "Filter 2 Strings"=w1180, "Ordinate"="Multi Ordinate", "Absisca"="Absisca", "Transpose"="Transpose") -> ("Accept Array Out"=→"Plotted Series":bool[][])  [unwired: 5 out]
          }
          frame #2 {
            n554 = Select(t="Intensity plot", s="Intensity Plot?", f="Add Legend and scales") -> (s? t:f=w1211:string)
            n555 = property on="Surface Area" class="DigNum (strict)"("Visible"="Intensity Plot?") -> ()  [unwired: 2 in, 2 out]
            n556 = property on="Surface Integral" class="DigNum (strict)"("Visible"="Intensity Plot?") -> ()  [unwired: 2 in, 2 out]
            n557 = property on="Surface Average" class="DigNum (strict)"("Visible"="Intensity Plot?") -> ()  [unwired: 2 in, 2 out]
            n558 = property on="X Ch Name" class="Ring (strict)"("Visible"="Intensity Plot?") -> ()  [unwired: 2 in, 2 out]
            n559 = property on="Y Ch Name" class="Ring (strict)"("Visible"="Intensity Plot?") -> ()  [unwired: 2 in, 2 out]
            n560 = property on="Z Ch Name" class="Ring (strict)"("Visible"="Intensity Plot?") -> ()  [unwired: 2 in, 2 out]
            n561 = property on="Point Size" class="Slide (strict)"("Visible"="Intensity Plot?") -> ()  [unwired: 2 in, 2 out]
            n562 = property on="No of Contours" class="DigNum (strict)"("Visible"="Intensity Plot?") -> ()  [unwired: 2 in, 2 out]
            n563 = property on="Slice mode" class="Enum (strict)"("Visible"="Intensity Plot?") -> ()  [unwired: 2 in, 2 out]
            n564 = property on="Plot Resolution" class="Bool (strict)"("Visible"="Intensity Plot?") -> ()  [unwired: 2 in, 2 out]
            n565 = property on="Update" class="Bool (strict)"("Visible"="Intensity Plot?") -> ()  [unwired: 2 in, 2 out]
          }
        }
        "Index when last plotted" <- w1102
      }
      frame "Add Legend and scales" {
        n566 = global read "Results_plotter_Global.vi" "Point info"() -> (w1225:T18)
        n567 = global read "Results_plotter_Global.vi" "Legend"() -> (w1226:string[])
        n568 = local read "Transpose"() -> (w1217:bool)
        n569 = global read "Results_plotter_Global.vi" "XY Graph Cluster"() -> (→"XY Plot":cluster{dbl[], dbl[]}[])
        n570 = global read "Results_plotter_Global.vi" "Plot Index values"() -> (w1220:dbl[][])
        n571 = for {
          tunnel: w1226 -> [w1257] mode=indexing
          tunnel: w1225 -> [w1266] mode=indexing
          tunnel: [w1267] -> w1230
          i -> [w1267]
          n572 = String Length(string=w1257) -> (length=w1263:i32)
          n573 = Subtract(x=w1263, y=2) -> (x-y=w1261:i32)
          n574 = String Subset(string=w1257, length (rest)=w1261) -> (substring=w1255:string)  [unwired: 1 out]
          n575 = call "Abbreviate_string.vi"("Input String"=w1255, "Max String Length"=35) -> ("Output String"=w1254:string)
          n576 = Unbundle By Name(w1266) -> ("Point Style"=w1265:u8, "Fill/Pt. Color"=w1264:u32, "Plot Interpolation"=w1252:u8)
          n577 = call "Fast_string_Replace.vi"("Replace match with:"="_", "Input String"=w1254, "regular expression"=" ") -> ("Output String"=w1258:string)  [unwired: 1 in, 1 out]
          n578 = property on="XY Plot" class="XYGraph (strict)"("Active Plot"=w1267, "Plot.Plot Name"=w1258, "Plot.Point Style"=w1265, "Plot.Fill/Point Color"=w1264, "Plot.Plot Color"=w1264, "LegAutosize"=FALSE ("Legend:Autosize"), "Plot.Plot Interpolation"=w1252) -> ()  [unwired: 2 in, 2 out]
        }
        n579 = Select(t=1 ("index (row)"), s=w1217, f=0 ("index (row)")) -> (s? t:f=w1214:i32)
        n580 = Index Array(array=w1220, index (row)=w1214) -> (element=w1219:dbl[])  [unwired: 1 in]
        n581 = Array Max & Min(array=w1219) -> (max value=w1218:dbl)  [unwired: 3 out]
        n582 = Greater?(x=w1218, y=2680560000.0) -> (0:w1222:bool)
        n583 = case shown="False" w1222 {
          tunnel: [w1237 u8 7 ("X Scale.Format & Precision:Precision")] -> w1221
          tunnel: w1218 -> [w1243 _]
          frame False {
            n584 = Absolute Value(x=w1243) -> (abs(x)=w1236:dbl)
            n585 = In Range and Coerce(upper limit=100000.0 ("y"), x=w1236, lower limit=0.0001) -> (In Range?=w1240:bool)  [unwired: 1 out]
            n586 = Select(t=u8 0 ("f"), s=w1240, f=u8 1) -> (s? t:f=w1237:u8)
          }
          frame True {
          }
        }
        n587 = Increment(x=w1230) -> (x+1=w1229:i32)
        n588 = for {
          N: 10 -> [_]
          tunnel: w1229 -> [w1250]
          i -> [w1251]
          w1247 = u32 0
          n589 = Add(x=w1250, y=w1251) -> (x+y=w1249:i32)
          n590 = property on="XY Plot" class="XYGraph (strict)"("Active Plot"=w1249, "Plot.Plot Name"="" ("Write Attribute"), "Plot.Plot Color"=w1247, "Plot.Fill/Point Color"=w1247, "LegAutosize"=FALSE ("Legend:Autosize"), "PlotVisCheckbox"=TRUE ("Legend:Plot Visibility Checkbox Visible")) -> ()  [unwired: 2 in, 2 out]
        }
        n591 = local write "Warning!"("") -> ()
        n592 = property on="XY Plot" class="XYGraph (strict)"("X Scale.Format & Precision:Format"=w1221) -> ()  [unwired: 2 in, 2 out]
      }
      frame "Add Axis names" {
        n593 = local read "Multi Ordinate"() -> (w1282:i32[])
        n594 = for {
          tunnel: w1282 -> [w1299] mode=indexing
          shift-right: [w1296] -> w1275
          shift-left: "" -> [w1295]
          tunnel: w1283 -> [w1298]
          tunnel: [w1291] -> w1274
          i -> [w1291]
          n595 = Index Array(array=w1298, index=w1299) -> (element=w1297:string)
          n596 = String Length(string=w1295) -> (length=w1294:i32)
          n597 = Less?(x=w1294, y=40) -> (x < y?=w1292:bool)
          n598 = case shown="True" w1292 {
            tunnel: w1297 -> [_ w1304]
            tunnel: [w1300 w1303] -> w1296
            tunnel: w1295 -> [w1300 w1301]
            frame False {
            }
            frame True {
              n599 = Concatenate Strings(w1301, w1304, "   ") -> (w1303:string)
            }
          }
        }
        n600 = Greater Than 0?(x=w1274) -> (x > 0?=w1272:bool)
        n601 = local read "Transpose"() -> (w1285:bool)
        n602 = local read "Absisca"() -> (w1286:u16)
        n603 = Index Array(array=w1283, index=w1286) -> (element=w1284:string)
        n604 = String Length(string=w1275) -> (length=w1278:i32)
        n605 = Empty String/Path?(string/path="Ordinate Name") -> (empty?=w1273:bool)
        n606 = Subtract(x=w1278, y=3) -> (x-y=w1276:i32)
        n607 = Compound Arithmetic op=AND(invert w1273, w1272) -> (w1271:bool)
        n608 = String Subset(string=w1275, length (rest)=w1276) -> (substring=w1270:string)  [unwired: 1 out]
        n609 = Select(t="Ordinate Name", s=w1271, f=w1270) -> (s? t:f=w1268:string)
        n610 = case shown="False" w1285 {
          tunnel: [w1305 w1308] -> w1281
          tunnel: w1268 -> [w1306 w1308]
          tunnel: [w1306 w1307] -> w1280
          tunnel: w1284 -> [w1305 w1307]
          frame False {
          }
          frame True {
          }
        }
        n611 = global write "Results_plotter_Global.vi" "X Axis Name"(w1281) -> ()
        n612 = global write "Results_plotter_Global.vi" "Y Axis Name"(w1280) -> ()
        n613 = global write "Results_plotter_Global.vi" "Value plotted Name"(w1268) -> ()
        n614 = property on="XY Plot" class="XYGraph (strict)"("X Scale.Name Label.Text"=w1281, "Y Scale.Name Label.Text"=w1280) -> ()  [unwired: 2 in, 2 out]
      }
      frame "Intensity plot" {
        # "Max"
        # "Min"
        n615 = global read "Results_plotter_Global.vi" "XY Graph Cluster"() -> (w1309:cluster{dbl[], dbl[]}[])
        n616 = local read "Tolerances"() -> (w1314:dbl[])
        n617 = local read "Absisca"() -> (w1313:u16)
        n618 = local read "Transpose"() -> (w1310:bool)
        n619 = stacked-sequence {
          seq-local: [w1327 _ _ _ _ _ _ _ _ _ _ _ _ _] -> [_ _ _ w1392 w1399 _ w1426 _ _ _ _ _ _ _]
          seq-local: [_ w1343 _ _ _ _ _ _ _ _ _ _ _ _] -> [_ _ _ _ w1398 _ w1425 _ _ _ _ _ _ _]
          seq-local: [_ _ w1375 _ _ _ _ _ _ _ _ _ _ _] -> [_ _ _ _ _ _ w1434 _ _ _ _ _ _ _]
          seq-local: [_ _ _ _ _ _ w1436 _ _ _ _ _ _ _] -> [_ _ _ _ _ _ _ _ _ w1469 _ _ _ _]
          seq-local: [_ _ _ _ _ _ w1435 _ _ _ _ _ _ _] -> [_ _ _ _ _ _ _ _ _ w1470 _ _ _ _]
          seq-local: [_ w1339 _ _ _ _ _ _ _ _ _ _ _ _] -> [_ _ _ _ _ _ _ _ _ _ w1534 _ _ _]
          seq-local: [_ _ _ w1390 _ _ _ _ _ _ _ _ _ _] -> [_ _ _ _ w1397 _ w1430 _ _ _ _ _ _ _]
          seq-local: [_ _ _ _ _ _ _ _ _ _ _ _ w1560 _] -> [_ _ _ _ _ _ _ _ _ _ _ _ _ w1610]
          seq-local: [_ _ _ _ _ _ _ _ _ _ _ _ w1559 _] -> [_ _ _ _ _ _ _ _ _ _ _ _ _ w1611]
          seq-local: [_ _ _ w1389 _ _ _ _ _ _ _ _ _ _] -> [_ _ _ _ _ w1412 _ _ _ _ _ _ _ _]
          seq-local: [_ _ _ _ _ _ _ _ _ _ _ _ w1557 _] -> [_ _ _ _ _ _ _ _ _ _ _ _ _ w1603]
          seq-local: [_ _ _ _ _ _ w1418 _ _ _ _ _ _ _] -> [_ _ _ _ _ _ _ w1447 _ _ _ _ _ _]
          tunnel: [_ _ _ TRUE _ _ _ _ _ _ _ _ _ _] -> w1320
          tunnel: [_ _ _ _ _ _ _ _ _ _ _ _ _ "Analyse Plot Space"] -> w1319
          tunnel: w1317 -> [w1324 _ _ _ _ _ _ _ _ _ _ _ _ _]
          tunnel: w1318 -> [w1325 _ w1376 _ _ _ _ _ _ _ w1515 _ _ _]
          tunnel: [w1325 _ _ _ _ _ _ _ _ _ _ _ _ _] -> w1316
          tunnel: [w1324 _ _ _ _ _ _ _ _ _ _ _ _ _] -> w1315
          tunnel: w1314 -> [w1329 _ _ _ _ _ _ _ _ _ _ _ _ _]
          tunnel: w1309 -> [w1328 _ _ w1394 _ _ _ _ _ _ _ _ _ _]
          tunnel: w1313 -> [w1326 _ _ _ _ _ _ _ _ _ w1531 _ _ _]
          tunnel: w1310 -> [w1323 _ _ w1391 _ _ w1438 _ _ _ w1529 _ _ _]
          tunnel: [_ w1344 _ _ _ _ _ _ _ _ _ _ _ _] -> w1312
          tunnel: w1311 -> [_ w1344 _ _ _ _ _ _ _ _ w1516 _ _ _]
          frame #0 {
            n620 = Not(x=w1323) -> (.not. x?=w1322:bool)
            n621 = for {
              tunnel: w1328 -> [w1338] mode=indexing
              tunnel: w1322 -> [w1335]
              shift-right: [w1333] -> w1330
              shift-left: dbl[] [] -> [w1334]
              n622 = Unbundle(w1338) -> (w1337:dbl[], w1336:dbl[])
              n623 = Select(t=w1337, s=w1335, f=w1336) -> (s? t:f=w1332:dbl[])
              n624 = Build Array (concatenate)(w1334, w1332) -> (w1333:dbl[])
            }
            n625 = Index Array(array=w1329, index=w1326) -> (element=w1321:dbl)
            n626 = call "Numeric_bins.vi"("Values"=w1330, "Tolerance"=w1321) -> ("Bin Centres"=w1327:dbl[])  [unwired: 2 out]
          }
          frame #1 {
            n627 = local read "Filter Bins 2"() -> (w1345:i32[])
            n628 = local read "Filter Bins 1"() -> (w1347:i32[])
            n629 = Array Size(array=w1345) -> (size(s)=w1349:i32)
            n630 = Array Size(array=w1347) -> (size(s)=w1350:i32)
            n631 = Greater Or Equal?(x=w1350, y=w1349) -> (x >= y?=w1348:bool)
            n632 = case shown="False" w1348 {
              tunnel: w1347 -> [_ w1372]
              tunnel: [w1368 w1372] -> w1346
              tunnel: [w1369 w1371] -> w1341
              tunnel: w1345 -> [w1368 _]
              tunnel: [1 0] -> w1339
              frame False {
                n633 = property on="Filter Bins 2" class="LstBox (strict)"() -> ("Item Names"=w1369:string[])  [unwired: 2 in, 2 out]
              }
              frame True {
                n634 = property on="Filter Bins 1" class="LstBox (strict)"() -> ("Item Names"=w1371:string[])  [unwired: 2 in, 2 out]
              }
            }
            n635 = Array Size(array=w1341) -> (size(s)=w1340:i32)
            n636 = for {
              tunnel: w1346 -> [w1355] mode=indexing
              tunnel: w1341 -> [w1361]
              shift-right: [w1358] -> w1343
              shift-left: dbl[] [] -> [w1359]
              tunnel: w1340 -> [w1354]
              n637 = Index Array(array=w1361, index=w1355) -> (element=w1357:string)
              n638 = Less?(x=w1355, y=w1354) -> (x < y?=w1353:bool)
              n639 = Match Pattern(string=w1357, regular expression=" (0)") -> (offset past match=w1356:i32)  [unwired: 4 out]
              n640 = Less Than 0?(x=w1356) -> (x < 0?=w1352:bool)
              n641 = And(x=w1352, y=w1353) -> (x .and. y?=w1351:bool)
              n642 = case shown="True" w1351 {
                tunnel: w1359 -> [w1362 w1366]
                tunnel: [w1362 w1365] -> w1358
                tunnel: w1357 -> [_ w1364]
                frame False {
                }
                frame True {
                  n643 = Fract/Exp String To Number(string=w1364) -> (number=w1363:dbl)  [unwired: 4 out]
                  n644 = Build Array (concatenate)(w1366, w1363) -> (w1365:dbl[])
                }
              }
            }
          }
          frame #2 {
            n645 = local read "Template"() -> (w1374:path)
            n646 = call "Valid_Path.vi"("Filename"=w1374) -> ("Valid Path?"=w1373:bool)
            n647 = case shown="True" w1373 {
              tunnel: w1374 -> [_ w1386]
              tunnel: w1376 -> [_ w1385]
              tunnel: [nan w1382] -> w1375
              frame False {
              }
              frame True {
                n648 = local read "Multi Ordinate"() -> (w1381:i32[])
                n649 = call "Read_Write_Template.vi"("Template File"=w1386, "Mode"=Global_mode."Read Global", "Channel names In"=w1385, "Data type"="Minimum Value") -> ("1D Info Out"=w1384:string[])  [unwired: 4 in, 7 out]
                n650 = Index Array(array=w1381, index=0 ("Index")) -> (element=w1380:i32)
                n651 = Index Array(array=w1384, index=w1380) -> (element=w1383:string)
                n652 = Fract/Exp String To Number(string=w1383, default (0 dbl)=nan) -> (number=w1382:dbl)  [unwired: 3 out]
              }
            }
          }
          frame #3 {
            n653 = call "Grid_Data.vi"("Transpose"=w1391, "XY Graph"=w1394, "Bin Centres"=w1392) -> ("No of Duplicates"=w1389:i32, "Grided data"=w1390:dbl[][])
          }
          frame #4 {
            n654 = for {
              tunnel: w1399 -> [w1404]
              tunnel: w1398 -> [w1403] mode=indexing
              tunnel: w1397 -> [w1402] mode=indexing
              shift-right: [w1400] -> w1395
              shift-left: dbl[][] [] -> [w1401]
              n655 = for {
                tunnel: w1404 -> [w1410] mode=indexing
                tunnel: w1403 -> [w1405]
                tunnel: w1402 -> [w1409] mode=indexing
                shift-right: [w1406] -> w1400
                shift-left: w1401 -> [w1408]
                n656 = Build Array(w1410, w1405, w1409) -> (w1407:dbl[])
                n657 = Build Array (concatenate)(w1408, w1407) -> (w1406:dbl[][])
              }
            }
            n658 = global write "Results_plotter_Global.vi" "Intensity Plot data in rows"(w1395) -> ()
          }
          frame #5 {
            n659 = case shown="1, Default" w1412 {
              tunnel: w1412 -> [_ w1416]
              tunnel: ["" w1414] -> w1411
              frame 0 {
              }
              frame 1, Default {
                n660 = Format Into String(format string="%d duplicate points have been averaged together!", w1416) -> (resulting string=w1414:string)  [unwired: 2 in, 1 out]
              }
            }
            "Warning!" <- w1411
          }
          frame #6 {
            n661 = call "Insert_extra_rows_and_col.vi"("Row Values In"=w1425, "Additional Row Values"="Additional X Values", "Column Values In"=w1426, "Data In"=w1430, "Additional Column Values"="Additional Y Values") -> ("Row Values Out"=w1427:dbl[], "Column Values Out"=w1428:dbl[], "Data Out"=w1429:dbl[][])  [unwired: 2 out]
            n662 = Select(t="Resolution", s="Plot Resolution", f=0.0) -> (s? t:f=w1420:dbl)
            n663 = call "2D_interpolation.vi"("X Axis Current"=w1428, "Min Z Value In"=w1434, "Y axis Current"=w1427, "Bkgnd Value"="Bkgnd Value", "Plot In"=w1429, "Increment Value"=w1420, "Transpose"=w1438, "Point Size"="Point Size") -> ("min Z value"=w1436:dbl, "max Z value"=w1435:dbl, "Increment Value Out"=w1424:dbl, "Axis info"=w1418:T19, "Plot Out"=→"Intensity Graph":dbl[][], "Raw Interpolation"=w1417:dbl[][])  [unwired: 2 out]
            n664 = global write "Results_plotter_Global.vi" "Raw Interpolation"(w1417) -> ()
            n665 = local write "Resolution"(w1424) -> ()
          }
          frame #7 {
            n666 = Unbundle By Name(w1447) -> ("X Max"=w1446:dbl, "Y Max"=w1445:dbl, "X Scale"=w1444:cluster{"Xo":dbl, "delta X":dbl}, "Y Scale"=w1443:cluster{"Xo":dbl, "delta X":dbl}, "X Values"=w1442:dbl[], "Y Values"=w1441:dbl[], "Z Max"=w1440:dbl, "Z Min"=w1439:dbl)
            n667 = global write "Results_plotter_Global.vi" "X Scale"(w1444) -> ()
            n668 = global write "Results_plotter_Global.vi" "X Values"(w1442) -> ()
            n669 = global write "Results_plotter_Global.vi" "Y Values"(w1441) -> ()
            n670 = global write "Results_plotter_Global.vi" "Y Scale"(w1443) -> ()
            n671 = global write "Results_plotter_Global.vi" "Y Max"(w1445) -> ()
            n672 = global write "Results_plotter_Global.vi" "Z Max"(w1440) -> ()
            n673 = global write "Results_plotter_Global.vi" "Z Min"(w1439) -> ()
            n674 = global write "Results_plotter_Global.vi" "X Max"(w1446) -> ()
          }
          frame #8 {
            n675 = global read "Results_plotter_Global.vi" "X Scale"() -> (w1455:cluster{"Xo":dbl, "delta X":dbl})
            n676 = global read "Results_plotter_Global.vi" "Y Scale"() -> (w1451:cluster{"Xo":dbl, "delta X":dbl})
            n677 = global read "Results_plotter_Global.vi" "Y Max"() -> (w1452:dbl)
            n678 = global read "Results_plotter_Global.vi" "X Max"() -> (w1453:dbl)
            n679 = Unbundle By Name(w1451) -> ("Xo"=w1450:dbl)
            n680 = Unbundle By Name(w1455) -> ("Xo"=w1454:dbl)
            n681 = Subtract(x=w1452, y=w1450) -> (x-y=w1456:dbl)
            n682 = Subtract(x=w1453, y=w1454) -> (x-y=w1465:dbl)
            n683 = Greater?(x=w1465, y=5.0) -> (0:w1463:bool)
            n684 = Greater?(x=w1456, y=5.0) -> (0:w1458:bool)
            n685 = Select(t=u8 0 ("Write Attribute"), s=w1463, f=u8 3) -> (s? t:f=w1449:u8)
            n686 = Select(t=u8 0 ("Write Attribute"), s=w1458, f=u8 3) -> (s? t:f=w1448:u8)
            n687 = property on="Intensity Graph" class="IntGraph (strict)"("X Scale.Offset and Multiplier"=w1455, "X Scale.Range:Maximum"=w1453, "Y Scale.Offset and Multiplier"=w1451, "Y Scale.Range:Maximum"=w1452, "X Scale.Format & Precision:Precision"=w1449, "Y Scale.Format & Precision:Precision"=w1448) -> ()  [unwired: 2 in, 2 out]
          }
          frame #9 {
            n688 = Greater Than 0?(x=w1470) -> (x > 0?=w1467:bool)
            n689 = Less Than 0?(x=w1469) -> (x < 0?=w1468:bool)
            n690 = And(x=w1467, y=w1468) -> (x .and. y?=w1466:bool)
            n691 = case shown="False" w1466 {
              tunnel: w1470 -> [w1499 w1513]
              tunnel: [w1507 w1511] -> w1472
              tunnel: w1469 -> [w1495 w1508]
              frame True {
                (unwired) u32 3743
                (unwired) u32 16721152
                n692 = Absolute Value(x=w1495) -> (abs(x)=w1494:dbl)
                n693 = Absolute Value(x=w1499) -> (abs(x)=w1501:dbl)
                n694 = Absolute Value(x=w1495) -> (abs(x)=w1502:dbl)
                n695 = Max & Min(x=w1501, y=w1502) -> (max(x,y)=w1497:dbl)  [unwired: 1 out]
                n696 = Divide(x=w1494, y=w1497) -> (x/y=w1488:dbl)
                n697 = Subtract(x=1.0, y=w1488) -> (x-y=w1487:dbl)
                n698 = Multiply(x=w1487, y=u32 255) -> (x*y=w1493:dbl)
                n699 = To Unsigned Long Integer(number=w1493) -> (unsigned 32bit integer=w1477:u32)
                n700 = Multiply(x=w1477, y=u32 256) -> (x*y=w1479:u32)
                n701 = Multiply(x=w1477, y=u32 65536) -> (x*y=w1476:u32)
                n702 = Compound Arithmetic op=ADD(w1476, w1479, u32 255) -> (w1475:u32)
                n703 = Bundle("min Z value"=w1495, w1475) -> (w1504:cluster{"min Z value":dbl, u32})  [unwired: 1 out]
                n704 = Divide(x=w1499, y=w1497) -> (x/y=w1492:dbl)
                n705 = Bundle("max Z value"=0.0, u32 16777215) -> (w1503:cluster{"max Z value":dbl, u32})  [unwired: 1 out]
                n706 = Subtract(x=1.0, y=w1492) -> (x-y=w1490:dbl)
                n707 = Multiply(x=w1490, y=u32 255) -> (x*y=w1486:dbl)
                n708 = To Unsigned Long Integer(number=w1486) -> (unsigned 32bit integer=w1473:u32)
                n709 = Multiply(x=w1473, y=u32 256) -> (x*y=w1483:u32)
                n710 = Compound Arithmetic op=ADD(w1473, w1483, u32 16711680) -> (w1474:u32)
                n711 = Bundle("max Z value"=w1499, w1474) -> (w1506:cluster{"max Z value":dbl, u32})  [unwired: 1 out]
                n712 = Build Array(w1506, w1504) -> (w1505:cluster{"min Z value":dbl, u32}[])
                n713 = Build Array (concatenate)(w1505, w1503) -> (w1507:cluster{"max Z value":dbl, u32}[])
              }
              frame False {
                n714 = Bundle("max Z value"=w1513, u32 16721152) -> (w1510:cluster{"max Z value":dbl, u32})  [unwired: 1 out]
                n715 = Bundle("min Z value"=w1508, u32 3743) -> (w1509:cluster{"min Z value":dbl, u32})  [unwired: 1 out]
                n716 = Build Array(w1510, w1509) -> (w1511:cluster{"min Z value":dbl, u32}[])
              }
            }
            n717 = property on="Intensity Graph" class="IntGraph (strict)"("Ignore Array"=FALSE ("Write Attribute"), "Z Scale.Marker Values[]"=w1472) -> ()  [unwired: 2 in, 2 out]
          }
          frame #10 {
            n718 = local read "Filter Array"() -> (w1533:u16[])
            n719 = Index Array(array=w1533, index=w1534) -> (element=w1532:u16)
            n720 = Decrement(x=w1532) -> (x-1=w1530:u16)
            n721 = local read "Multi Ordinate"() -> (w1520:i32[])
            n722 = Index Array(array=w1516, index=w1530) -> (element=w1524:string)
            n723 = Index Array(array=w1516, index=w1531) -> (element=w1523:string)
            n724 = case shown="False" w1529 {
              tunnel: [w1536 w1538] -> w1522
              tunnel: w1524 -> [w1536 w1537]
              tunnel: w1523 -> [w1535 w1538]
              tunnel: [w1535 w1537] -> w1521
              frame False {
              }
              frame True {
              }
            }
            n725 = Index Array(array=w1520, index=0) -> (element=w1518:i32)
            n726 = Index Array(array=w1515, index=w1518) -> (element=w1517:string)
            n727 = global write "Results_plotter_Global.vi" "Value plotted Name"(w1517) -> ()
            n728 = property on="Intensity Graph" class="IntGraph (strict)"("X Scale.Name Label.Text"=w1521, "Y Scale.Name Label.Text"=w1522) -> ()  [unwired: 2 in, 2 out]
            n729 = global write "Results_plotter_Global.vi" "Y Axis Name"(w1521) -> ()
            n730 = global write "Results_plotter_Global.vi" "X Axis Name"(w1522) -> ()
            n731 = Format Into String(format string="Add %s values", w1524) -> (resulting string=→"First Add label":string)  [unwired: 2 in, 1 out]
            n732 = Format Into String(format string="Add %s values", w1523) -> (resulting string=→"2nd Add label":string)  [unwired: 2 in, 1 out]
          }
          frame #11 {
            n733 = property on="Intensity Graph" class="IntGraph (strict)"() -> ("Color Table"=w1540:u32[])  [unwired: 2 in, 2 out]
            n734 = Increment(x="No of Contours") -> (x+1=w1541:i32)
            n735 = Divide(x=255, y=w1541) -> (x/y=w1545:dbl)
            n736 = To Long Integer(number=w1545) -> (32bit integer=w1544:i32)
            n737 = for {
              tunnel: w1544 -> [w1553]
              tunnel: [w1550] -> w1539 mode=indexing
              tunnel: w1540 -> [w1549] mode=indexing
              tunnel: u32 0 -> [w1548]
              i -> [w1554]
              n738 = Increment(x=w1554) -> (x+1=w1551:i32)
              n739 = Quotient & Remainder(x=w1551, y=w1553) -> (x-y*floor(x/y)=w1552:i32)  [unwired: 1 out]
              n740 = case shown="0" w1552 {
                tunnel: [w1555 w1556] -> w1550
                tunnel: w1549 -> [_ w1556]
                tunnel: w1548 -> [w1555 _]
                frame 0 {
                }
                frame 1, Default {
                }
              }
            }
            n741 = property on="Intensity Graph" class="IntGraph (strict)"("Ignore Array"=TRUE ("Write Attribute"), "Color Table"=w1539) -> ()  [unwired: 2 in, 2 out]
          }
          frame #12 {
            n742 = global read "Results_plotter_Global.vi" "Raw Interpolation"() -> (w1558:dbl[][])
            n743 = Add Array Elements(numeric array=w1558) -> (sum=w1557:dbl)
            n744 = Array Size(array=w1558) -> (size(s)=w1568:i32[])
            n745 = Decrement(x=w1568) -> (x-1=w1566:i32[])
            n746 = Index Array(array=w1566, index=0) -> (element=w1567:i32)
            n747 = Index Array(array=w1566, index=1) -> (element=w1563:i32)
            n748 = for {
              N: w1567 -> [_]
              tunnel: w1558 -> [w1576]
              tunnel: w1563 -> [w1575]
              shift-right: [w1571] -> w1560
              shift-left: 0.0 -> [w1572]
              shift-right: [w1570] -> w1559
              shift-left: 0 -> [w1569]
              i -> [w1574]
              n749 = Increment(x=w1574) -> (x+1=w1573:i32)
              n750 = for {
                N: w1575 -> [_]
                tunnel: w1576 -> [w1585]
                tunnel: w1574 -> [w1590]
                tunnel: w1573 -> [w1588]
                shift-right: [w1581] -> w1571
                shift-left: w1572 -> [w1580]
                shift-right: [w1577] -> w1570
                shift-left: w1569 -> [w1578]
                i -> [w1589]
                n751 = Increment(x=w1589) -> (x+1=w1587:i32)
                n752 = Index Array(array=w1585, index (row)=w1590, index (col)=w1587) -> (element=w1586:dbl)
                n753 = Index Array(array=w1585, index (row)=w1588, index (col)=w1587) -> (element=w1583:dbl)
                n754 = Index Array(array=w1585, index (row)=w1590, index (col)=w1589) -> (element=w1591:dbl)
                n755 = Index Array(array=w1585, index (row)=w1588, index (col)=w1589) -> (element=w1584:dbl)
                n756 = Compound Arithmetic op=ADD(w1591, w1586, w1584, w1583) -> (w1579:dbl)
                n757 = Not A Number/Path/Refnum?(number/path/refnum=w1579) -> (NaN/Path/Refnum?=w1582:bool)
                n758 = case shown="False" w1582 {
                  tunnel: [w1595 w1599] -> w1581
                  tunnel: w1580 -> [w1597 w1599]
                  tunnel: w1579 -> [w1596 _]
                  tunnel: [w1594 w1598] -> w1577
                  tunnel: w1578 -> [w1593 w1598]
                  frame False {
                    n759 = Add(x=w1596, y=w1597) -> (x+y=w1595:dbl)
                    n760 = Add(x=1, y=w1593) -> (x+y=w1594:i32)
                  }
                  frame True {
                  }
                }
              }
            }
          }
          frame #13 {
            n761 = local read "Resolution"() -> (w1612:dbl)
            n762 = Divide(x=w1610, y=4.0) -> (x/y=w1608:dbl)
            n763 = Multiply(x=w1612, y=w1612) -> (x*y=w1604:dbl)
            n764 = Multiply(x=w1604, y=w1603) -> ()  [unwired: 1 out]
            n765 = Multiply(x=w1604, y=w1611) -> (x*y=w1605:dbl)
            "Surface Area" <- w1605
            n766 = Multiply(x=w1604, y=w1608) -> (x*y=w1601:dbl)
            "Surface Integral" <- w1601
            n767 = global write "Results_plotter_Global.vi" "Surface Area"(w1605) -> ()
            n768 = global write "Results_plotter_Global.vi" "Surface Integral"(w1601) -> ()
            n769 = Divide(x=16666667, y=w1601) -> (x/y=→"Uadvec":dbl)
            n770 = Divide(x=w1601, y=w1605) -> (x/y=→"Surface Average":dbl)
          }
        }
      }
      frame "Analyse Plot Space" {
        n771 = case shown="True" "Show Plot Space Analysis" {
          tunnel: w1617 -> [_ w1627]
          tunnel: w1614 -> [_ w1626]
          frame False {
          }
          frame True {
            w1623 = TRUE  # Summarise All
            n772 = global read "Results_plotter_Global.vi" "Plot Index values"() -> (w1621:dbl[][])
            n773 = Index Array(array=w1621, index (row)=2) -> (element=w1620:dbl[])  [unwired: 1 in]
            n774 = To Long Integer(number=w1620) -> (32bit integer=w1619:i32[])
            n775 = for {
              tunnel: w1619 -> [w1630] mode=indexing
              tunnel: w1627 -> [w1629]
              tunnel: [w1628] -> w1624 mode=indexing
              n776 = Index Array(array=w1629, index (row)=w1630) -> (element=w1628:string[])  [unwired: 1 in]
            }
            n777 = call "Summarise.vi"("Channel Names"=w1626, "Data"=w1624, "Summarise All"=w1623) -> ("Summary"=w1625:string[][])  [unwired: 2 in]
            n778 = call "Plot_Space_Analysis.vi"("Table"=w1625) -> ()
          }
        }
      }
      frame "Vector Plot" {
        n779 = flat-sequence {
          tunnel: w1635 -> [w1640]
          tunnel: w1633 -> [w1639]
          frame #0 {
            n780 = local read "Job Directory"() -> (w1638:path)
            n781 = Build Path(base path=w1638, name or relative path="Vectors") -> (appended path=w1637:path)
            n782 = local read "Template"() -> (w1641:path)
            n783 = call "Vector_Plotting.vi"("JobVectorDirectory"=w1637, "Data"=w1639, "Template Filename"=w1641, "Channel Names"=w1640) -> ()  [unwired: 1 in]
          }
          frame #1 {
            n784 = local write "Vector Plot?"(FALSE ("Vector Plot?")) -> ()
          }
        }
      }
      frame "Coloured Dot Plot" {
        n785 = flat-sequence {
          tunnel: w1647 -> [w1652]
          tunnel: w1645 -> [w1651]
          frame #0 {
            n786 = local read "Job Directory"() -> (w1650:path)
            n787 = Build Path(base path=w1650, name or relative path="Dot_Plot") -> (appended path=w1649:path)
            n788 = local read "Template"() -> (w1653:path)
            n789 = call "Coloured_Dot_Plotting.vi"("JobVectorDirectory"=w1649, "Data"=w1651, "Template Filename"=w1653, "Channel Names"=w1652) -> ()  [unwired: 1 in]
          }
          frame #1 {
            n790 = local write "Dot Plot?"(FALSE ("Vector Plot?")) -> ()
          }
        }
      }
      frame "What to do next?" {
        # "Should probably be Event-ified"
        n791 = property on="XY Plot" class="XYGraph (strict)"() -> ("YScale.Maximum"=w1656:dbl, "YScale.Minimum"=w1657:dbl, "XScale.Maximum"=w1658:dbl, "XScale.Minimum"=w1659:dbl)  [unwired: 2 in, 2 out]
        n792 = global write "Results_plotter_Global.vi" "First Loop"(FALSE) -> ()
        n793 = case shown="False" "Add results file" {
          tunnel: [w1693 "More files options"] -> w1674
          tunnel: "Edit Template File" -> [w1684 _]
          frame False {
            n794 = Select(t="Edit template file", s=w1684, f="What to do next 2nd?") -> (s? t:f=w1682:string)
            n795 = Or(x="Save Plot data", y="Save Surface Fit") -> (x .or. y?=w1686:bool)
            n796 = Select(t="Save Plot Data", s=w1686, f=w1682) -> (s? t:f=w1689:string)
            n797 = Select(t="Create Plot summary", s="Save Plot as jpg", f=w1689) -> (s? t:f=w1680:string)
            n798 = Select(t="Save Data in Rows", s="Save Data in Rows", f=w1680) -> (s? t:f=w1693:string)
          }
          frame True {
            n799 = local write "Add results file"(FALSE) -> ()
          }
        }
        n800 = global write "Results_plotter_Global.vi" "Y plot min"(w1657) -> ()
        n801 = global write "Results_plotter_Global.vi" "X plot min"(w1659) -> ()
        n802 = global write "Results_plotter_Global.vi" "Y plot max"(w1656) -> ()
        n803 = global write "Results_plotter_Global.vi" "X plot max"(w1658) -> ()
        n804 = local read "Warning!"() -> (w1671:string)
        n805 = Select(t="Save Setup", s="stop", f=w1674) -> (s? t:f=w1665:string)
        n806 = Empty String/Path?(string/path=w1671) -> (empty?=w1670:bool)
        n807 = Not(x=w1670) -> (.not. x?=w1669:bool)
        n808 = Select(t="Vector Plot", s="Vector Plot?", f=w1665) -> (s? t:f=w1661:string)
        n809 = property on="Warning!" class="Str"("Visible"=w1669, "Blinking"=w1669) -> ()  [unwired: 2 in, 2 out]
        n810 = Select(t="Coloured Dot Plot", s="Dot Plot?", f=w1661) -> (s? t:f=w1660:string)
      }
      frame "What to do next 2nd?" {
        n811 = local read "Empty"() -> (w1717:bool)
        n812 = local read "Last used Template"() -> (w1705:path)
        n813 = local read "Template"() -> (w1697:path)
        n814 = Select(t="Empty Results file array", s=w1717, f="What to do next 3rd?") -> (s? t:f=w1700:string)
        n815 = global write "Results_plotter_Global.vi" "Template"(w1697) -> ()
        n816 = Not Equal?(x=w1705, y=w1697) -> (x != y?=w1704:bool)
        n817 = local read "Selected Row"() -> (w1696:i32)
        n818 = Select(t="What type of row averaging?", s="Save Averaged rows", f=w1700) -> (s? t:f=w1712:string)
        n819 = case shown="True" "Delete Plotted data from file" {
          tunnel: [w1747 "Full Res file manipulator" ("t")] -> w1710
          tunnel: w1712 -> [w1747 _]
          frame False {
          }
          frame True {
            n820 = local write "Plotted rows only?"(TRUE ("Save Plotted rows only?")) -> ()
            n821 = local write "Mode"(Plotter_Mode."Delete unwanted rows" ("Mode")) -> ()
          }
        }
        n822 = case shown="True" "Add /Edit metadata" {
          tunnel: [w1722 w1739] -> w1702
          tunnel: w1710 -> [w1723 w1740]
          tunnel: w1708 -> [_ w1738]
          tunnel: "Reload Files" -> [w1724 _]
          tunnel: [string[] [] ("New Chs Out") w1734] -> w1699
          tunnel: [string[][] [] w1733] -> w1698
          tunnel: w1696 -> [_ w1729]
          frame False {
            n823 = Select(t="Initialise", s=w1724, f=w1723) -> (s? t:f=w1722:string)
          }
          frame True {
            n824 = local read "Result files to read"() -> (w1735:path[])
            n825 = call "Edit_Channel_Panel.vi"("All Channel names"=w1738, "Result files to read"=w1735, "Selected Row"=w1729) -> ("New Values Out"=w1746:string[], "New Chs Out"=w1734:string[], "Cancel Out"=w1737:bool, "Edit Raw Data Header Info Out"=w1731:bool, "Plotted rows only?"=w1745:bool, "Selected Row?"=→"Selected Row?":bool, "Edit Raw data files?"=w1727:bool, "Raw data files in Orig Positions?"=w1726:bool, "Mode"=w1743:T7)  [unwired: 4 out]
            "Edit Raw Data Header Info" <- w1731
            n826 = local write "Edit Raw Data Files?"(w1727) -> ()
            n827 = Array Size(array=w1734) -> (size(s)=w1742:i32)
            n828 = local write "Raw DF in Orig Pos?"(w1726) -> ()
            n829 = Build Array(w1746) -> (w1733:string[][])
            n830 = local write "Add /Edit metadata"(FALSE ("Add /Edit metadata")) -> ()
            n831 = Greater Than 0?(x=w1742) -> (x > 0?=w1732:bool)
            n832 = local write "Plotted rows only?"(w1745) -> ()
            n833 = Or(x=w1731, y=w1732) -> (x .or. y?=w1730:bool)
            n834 = local write "Mode"(w1743) -> ()
            n835 = Compound Arithmetic op=AND(invert w1737, w1730) -> (w1736:bool)
            n836 = Select(t="Full Res file manipulator", s=w1736, f=w1740) -> (s? t:f=w1739:string)
          }
        }
        n837 = global write "Results_plotter_Global.vi" "New Chs In"(w1699) -> ()
        n838 = global write "Results_plotter_Global.vi" "New Values In"(w1698) -> ()
        n839 = Select(t="Initialise", s=w1704, f=w1702) -> (s? t:f=w1701:string)
      }
      frame "What to do next 3rd?" {
        n840 = local read "Show Results Space Analysis"() -> (w1768:bool)
        n841 = local read "Show Plot Space Analysis"() -> (w1767:bool)
        n842 = while {
          shift-right: [w1795] -> _
          shift-left: _ -> [w1794]
          shift-left: _ -> [w1793]
          shift-left: _ -> [w1792]
          tunnel: w1768 -> [w1795]
          shift-right: [w1800] -> _
          shift-left: _ -> [w1799]
          shift-left: _ -> [w1798]
          shift-left: _ -> [w1797]
          tunnel: w1767 -> [w1800]
          tunnel: [w1796] -> w1766
          tunnel: [w1791] -> w1765
          stop <- TRUE stop-if-true
          n843 = Compound Arithmetic op=AND(w1795, w1794, w1793, w1792) -> (w1791:bool)
          n844 = Compound Arithmetic op=AND(w1800, w1799, w1798, w1797) -> (w1796:bool)
        }
        n845 = local read "Index when last displayed"() -> (w1755:i32)
        n846 = local read "Index when last plotted"() -> (w1754:i32)
        n847 = global write "Results_plotter_Global.vi" "Plot EnFlo Tunnel Display"("Plot EnFlo Tunnel Display") -> ()
        n848 = Select(t="Run Calculation Routine", s="Calculate new metadata", f="What to do next 4th?") -> (s? t:f=w1774:string)
        n849 = case shown="True" w1766 {
          frame False {
          }
          frame True {
            n850 = Open VI Reference(vi path="Plot_Space_Analysis.vi" ("VI path")) -> (vi reference=w1812:refnum<vi>, error out=w1811:errorcluster)  [unwired: 1 in, 4 out]
            n851 = property class="VI"(reference=w1812, error in=w1811) -> (reference out=w1810:refnum<vi>, error out=w1809:errorcluster, "Front Panel Window:Open"=w1807:bool)
            n852 = local write "Show Plot Space Analysis"(w1807) -> ()
            n853 = Close Reference(reference=w1810, error in (no error)=w1809) -> ()  [unwired: 1 out]
          }
        }
        n854 = case shown="True" w1765 {
          frame False {
          }
          frame True {
            n855 = Open VI Reference(vi path="Results_Space_Analysis.vi" ("VI path")) -> (vi reference=w1806:refnum<vi>, error out=w1805:errorcluster)  [unwired: 1 in, 4 out]
            n856 = property class="VI"(reference=w1806, error in=w1805) -> (reference out=w1804:refnum<vi>, error out=w1803:errorcluster, "Front Panel Window:Open"=w1801:bool)
            n857 = local write "Show Results Space Analysis"(w1801) -> ()
            n858 = Close Reference(reference=w1804, error in (no error)=w1803) -> ()  [unwired: 1 out]
          }
        }
        n859 = Select(t="Save Setup", s="Save Setup", f=w1774) -> (s? t:f=w1771:string)
        n860 = Select(t="Choose Setup file", s="Load Setup", f=w1771) -> (s? t:f=w1764:string)
        n861 = Not Equal?(x=w1754, y=w1755) -> (x != y?=w1753:bool)
        n862 = And(x=w1753, y="Plot EnFlo Tunnel Display") -> (x .and. y?=w1752:bool)
        n863 = Or(x="Kill Point", y="Process Point") -> (x .or. y?=w1761:bool)
        n864 = Select(t="Process cursor point", s=w1761, f=w1764) -> (s? t:f=w1758:string)
        n865 = case shown="True" "Post Process Plotted Data" {
          tunnel: [w1786 "Full Res file manipulator" ("t")] -> w1757
          tunnel: w1758 -> [w1786 _]
          frame False {
          }
          frame True {
            n866 = local write "Plotted rows only?"(TRUE ("Plotted rows only?")) -> ()
            n867 = local write "Mode"(Plotter_Mode."Post Process Plotted Rows" ("Mode")) -> ()
          }
        }
        n868 = case shown="True" w1752 {
          tunnel: [w1782 "Full Res file manipulator" ("t")] -> w1756
          tunnel: w1757 -> [w1782 _]
          frame False {
          }
          frame True {
            n869 = local write "Plotted rows only?"(TRUE ("Plotted rows only?")) -> ()
            n870 = local write "Mode"(Plotter_Mode."Plot EnFlo Tunnel Display" ("Mode")) -> ()
          }
        }
      }
      frame "What to do next 4th?" {
        n871 = case shown="True" "Add Inlet Temperature offset" {
          tunnel: [w1820 "Full Res file manipulator" ("t")] -> w1814
          tunnel: "Time to save setup?" -> [w1820 _]
          frame False {
          }
          frame True {
            n872 = local write "Plotted rows only?"(TRUE ("Plotted rows only?")) -> ()
            n873 = local write "Mode"(Plotter_Mode."Add Inlet Temperature Offset" ("Mode")) -> ()
          }
        }
      }
      frame "Time to save setup?" {
        n874 = stacked-sequence {
          seq-local: [w1832 _] -> [_ w1872]
          seq-local: [w1831 _] -> [_ w1871]
          tunnel: [w1840 _] -> w1826
          tunnel: w1825 -> [w1830 _]
          frame #0 {
            n875 = while {
              shift-right: [w1862] -> _
              shift-left: _ -> [w1860]
              shift-right: [w1849] -> _
              shift-left: _ -> [w1857]
              tunnel: [w1849] -> w1839
              tunnel: [w1848] -> w1838
              shift-right: [w1850] -> _
              shift-left: _ -> [w1856]
              tunnel: [w1854] -> w1833
              tunnel: [w1851] -> w1834
              tunnel: [w1850] -> w1835
              tunnel: [w1847] -> w1831
              tunnel: w1830 -> [w1843]
              stop <- FALSE continue-if-true
              n876 = Get Date/Time In Seconds() -> (seconds since 1Jan1904=w1858:timestamp)
              n877 = To Double Precision Float(number=w1858) -> (double precision float=w1861:dbl)
              n878 = local read "Show Results Space Analysis"() -> (w1849:bool)
              n879 = local read "Show Plot Space Analysis"() -> (w1850:bool)
              n880 = Subtract(x=w1861, y=w1860) -> (x-y=w1863:dbl)
              n881 = Greater?(x=w1863, y="Save Setup Interval (s)") -> (0:w1845:bool)
              n882 = Greater?(x=w1843, y=300) -> (0:w1842:bool)
              n883 = And(x=w1845, y=w1842) -> (x .and. y?=w1844:bool)
              n884 = case shown="False" w1844 {
                tunnel: [w1864 w1870] -> w1862
                tunnel: w1861 -> [w1865 w1870]
                tunnel: w1860 -> [w1866 _]
                tunnel: ["Check modification dates?" "Save Setup"] -> w1853
                tunnel: w1842 -> [w1867 _]
                frame False {
                  n885 = Select(t=w1866, s=w1867, f=w1865) -> (s? t:f=w1864:dbl)
                }
                frame True {
                }
              }
              n886 = Not Equal?(x=w1850, y=w1856) -> (x != y?=w1851:bool)
              n887 = Not Equal?(x=w1849, y=w1857) -> (x != y?=w1848:bool)
              n888 = Compound Arithmetic op=AND(invert w1849, w1848) -> (w1847:bool)
              n889 = And(x=w1850, y=w1851) -> (x .and. y?=w1855:bool)
              n890 = Select(t="Analyse Plot Space", s=w1855, f=w1853) -> (s? t:f=w1854:string)
            }
            n891 = Compound Arithmetic op=AND(invert w1835, w1834) -> (w1832:bool)
            n892 = And(x=w1839, y=w1838) -> (x .and. y?=w1837:bool)
            n893 = Select(t="What is present?", s=w1837, f=w1833) -> (s? t:f=w1840:string)
          }
          frame #1 {
            n894 = case shown="True" w1871 {
              frame False {
              }
              frame True {
                n895 = Open VI Reference(vi path="Results_Space_Analysis.vi" ("VI path")) -> (vi reference=w1878:refnum<vi>, error out=w1877:errorcluster)  [unwired: 1 in, 4 out]
                n896 = property class="VI"(reference=w1878, error in=w1877, "Front Panel Window:Open"=FALSE) -> (reference out=w1876:refnum<vi>, error out=w1875:errorcluster)
                n897 = Close Reference(reference=w1876, error in (no error)=w1875) -> ()  [unwired: 1 out]
              }
            }
            n898 = case shown="True" w1872 {
              frame False {
              }
              frame True {
                n899 = Open VI Reference(vi path="Plot_Space_Analysis.vi" ("VI path")) -> (vi reference=w1884:refnum<vi>, error out=w1883:errorcluster)  [unwired: 1 in, 4 out]
                n900 = property class="VI"(reference=w1884, error in=w1883, "Front Panel Window:Open"=FALSE) -> (reference out=w1882:refnum<vi>, error out=w1881:errorcluster)
                n901 = Close Reference(reference=w1882, error in (no error)=w1881) -> ()  [unwired: 1 out]
              }
            }
          }
        }
      }
      frame "Check modification dates?" {
        n902 = while {
          shift-right: [w1903] -> _
          shift-left: _ -> [w1901]
          tunnel: [w1900] -> w1893
          stop <- FALSE continue-if-true
          n903 = Get Date/Time In Seconds() -> (seconds since 1Jan1904=w1898:timestamp)
          n904 = To Double Precision Float(number=w1898) -> (double precision float=w1902:dbl)
          n905 = Subtract(x=w1902, y=w1901) -> (x-y=w1906:dbl)
          n906 = Greater?(x=w1906, y=200.0) -> (0:w1904:bool)
          n907 = case shown="True" w1904 {
            tunnel: [w1908 w1911] -> w1903
            tunnel: w1902 -> [_ w1911]
            tunnel: w1901 -> [w1908 _]
            tunnel: [FALSE w1909] -> w1900
            frame False {
            }
            frame True {
              n908 = global read "Results_plotter_Global.vi" "First Loop"() -> (w1910:bool)
              n909 = Not(x=w1910) -> (.not. x?=w1909:bool)
            }
          }
        }
        n910 = Equal?(x="Tab Control", y=enum32{"Load ", "Plot ", "Save ", "Cursor"}."Cursor" ("Tab Control")) -> (x = y?=w1889:bool)
        n911 = Select(t="Read Cursor", s=w1889, f="Ordinate Selector Type") -> (s? t:f=w1887:string)
        n912 = Select(t="Files Modified?", s=w1893, f=w1887) -> (s? t:f=w1892:string)
      }
      frame "Files Modified?" {
        n913 = local read "nRows"() -> (w1915:i32)
        n914 = Less?(x=w1915, y=w1914) -> (x < y?=w1912:bool)
        n915 = case shown="True" w1912 {
          tunnel: [w1921 w1927] -> w1916
          tunnel: "Ordinate Selector Type" -> [w1921 w1922]
          frame False {
          }
          frame True {
            n916 = local read "Result files to read"() -> (w1926:path[])
            n917 = for {
              tunnel: w1926 -> [w1930] mode=indexing
              tunnel: [w1928] -> w1925 mode=indexing
              n918 = call "File_Modified_Since_Check.vi"("Pathname"=w1930, "Just Modified?"=TRUE) -> ("Modified?"=w1928:bool)
            }
            n919 = Or Array Elements(Boolean array=w1925) -> (logical OR=w1924:bool)
            n920 = Select(t="Initialise", s=w1924, f=w1922) -> (s? t:f=w1927:string)
          }
        }
      }
      frame "Read Cursor" {
        n921 = global read "Results_plotter_Global.vi" "Plot Index values"() -> (w1939:dbl[][])
        n922 = local read "Transpose"() -> (w1946:bool)
        n923 = property on="XY Plot" class="XYGraph (strict)"() -> ("Cursor.Cursor Position:Cursor X"=w1933:dbl, "Cursor.Cursor Position:Cursor Y"=w1932:dbl)  [unwired: 2 in, 2 out]
        n924 = case shown="True" w1946 {
          tunnel: [w1955 w1957] -> w1945
          tunnel: w1933 -> [w1955 w1956]
          tunnel: [w1954 w1956] -> w1944
          tunnel: w1932 -> [w1954 w1957]
          frame False {
          }
          frame True {
          }
        }
        n925 = Index Array(array=w1939, index (row)=1) -> (element=w1937:dbl[])  [unwired: 1 in]
        n926 = Index Array(array=w1939, index (row)=2) -> (element=w1936:dbl[])  [unwired: 1 in]
        n927 = Index Array(array=w1939, index (row)=0) -> (element=w1938:dbl[])  [unwired: 1 in]
        n928 = for {
          tunnel: w1945 -> [w1966]
          tunnel: w1944 -> [w1965]
          tunnel: [w1960] -> w1943 mode=indexing
          tunnel: w1938 -> [w1959] mode=indexing
          tunnel: w1937 -> [w1958] mode=indexing
          n929 = Subtract(x=w1966, y=w1959) -> (x-y=w1964:dbl)
          n930 = Subtract(x=w1965, y=w1958) -> (x-y=w1963:dbl)
          n931 = Multiply(x=w1963, y=w1963) -> (x*y=w1962:dbl)
          n932 = Multiply(x=w1964, y=w1964) -> (x*y=w1961:dbl)
          n933 = Add(x=w1961, y=w1962) -> (x+y=w1960:dbl)
        }
        n934 = Array Max & Min(array=w1943) -> (min index (indices)=w1935:i32)  [unwired: 3 out]
        n935 = Index Array(array=w1936, index=w1935) -> (element=w1934:dbl)
        n936 = To Long Integer(number=w1934) -> (32bit integer=w1931:i32)
        "Cursor index" <- w1931
        n937 = Index Array(array=w1952, index (row)=w1931) -> (element=w1948:string[])  [unwired: 1 in]
        n938 = for {
          tunnel: w1951 -> [w1974] mode=indexing
          tunnel: w1948 -> [w1967] mode=indexing
          tunnel: [w1973] -> w1947 mode=indexing
          n939 = while {
            shift-right: [w1986] -> _
            shift-left: w1967 -> [w1987]
            tunnel: [w1983] -> w1971
            tunnel: [w1982] -> w1969 mode=indexing
            i -> [w1983]
            stop <- w1984 continue-if-true
            n940 = Match Pattern(string=w1987, regular expression=":") -> (before substring=w1982:string, after substring=w1986:string, offset past match=w1985:i32)  [unwired: 2 out]
            n941 = Greater Than 0?(x=w1985) -> (x > 0?=w1984:bool)
          }
          n942 = Greater?(x=w1971, y=2) -> (0:w1970:bool)
          n943 = Reverse 1D Array(array=w1969) -> (reversed array=w1968:string[])
          n944 = case shown="True" w1970 {
            tunnel: w1974 -> [w1977 w1981]
            tunnel: [w1975 w1980] -> w1973
            tunnel: w1968 -> [_ w1979]
            tunnel: w1967 -> [w1976 w1978]
            frame False {
              n945 = Build Array(w1977, w1976) -> (w1975:string[])
            }
            frame True {
              n946 = Build Array (concatenate)(w1981, w1979, w1978) -> (w1980:string[])
            }
          }
        }
        "Table" <- w1947
      }
      frame "Process Cursor Point" {
        n947 = stacked-sequence {
          tunnel: [w2005] -> w1993
          tunnel: [TRUE] -> w1992
          tunnel: w1991 -> [w1996]
          tunnel: w1990 -> [w1998]
          tunnel: w1989 -> [w2006]
          frame #0 {
            n948 = local read "Kill Point"() -> (w2007:bool)
            n949 = global read "Results_plotter_Global.vi" "Row Reference"() -> (w2012:i32[][])
            n950 = local read "Cursor index"() -> (w2011:i32)
            n951 = Index Array(array=w2012, index (row)=w2011) -> (element=w2008:i32[])  [unwired: 1 in]
            n952 = local read "Result files to read"() -> (w2010:path[])
            n953 = Index Array(array=w2008) -> (element #1=w2009:i32, element #2=w1997:i32)  [unwired: 3 in, 1 out]
            "Selected Row" <- w1997
            n954 = Index Array(array=w1996, index (row)=w1997) -> (element=w1995:string[])  [unwired: 1 in]
            n955 = Index Array(array=w2010, index=w2009) -> (element=w2004:path)
            n956 = call "GetRawDataFilePaths.vi"("Results file or Folder"=w2004) -> ("RawDataFilePaths"=w2003:string[], "RowNumbers"=w2000:i32[])  [unwired: 9 in]
            n957 = Search 1D Array(1D array=w2000, element=w1997) -> (index of element=w1999:i32)  [unwired: 1 in]
            n958 = Index Array(array=w2003, index=w1999) -> (element=w2002:string)
            n959 = call "String_to_Pathname.vi"("Input String"=w2002) -> ("path"=w2001:path)
            n960 = case shown="True" w2007 {
              tunnel: w2004 -> [_ w2038]
              tunnel: w1997 -> [_ w2034]
              tunnel: w2006 -> [_ w2041]
              tunnel: ["What to do next?" ("t") w2040] -> w2005
              tunnel: w2001 -> [w2016 w2032]
              tunnel: w1998 -> [w2015 _]
              tunnel: w1995 -> [w2014 _]
              frame False {
                n961 = disable-structure shown="Enabled" {
                  disable-tunnel: w2016 -> [_ w2030]
                  disable-tunnel: w2015 -> [_ w2029]
                  disable-tunnel: w2014 -> [_ w2028]
                  frame Disabled {
                    n962 = local read "Table"() -> (w2027:string[][])
                    n963 = Index Array(array=w2027, index (col) #1=1 ("disabled index (col)"), index (col) #2=0 ("index (col)")) -> (element #1=w2020:string[], element #2=w2019:string[])  [unwired: 2 in]
                    n964 = Search 1D Array(1D array=w2019, element="Raw Data Filename") -> (index of element=w2023:i32)  [unwired: 1 in]
                    n965 = Index Array(array=w2020, index=w2023) -> (element=w2022:string)
                    n966 = call "String_to_Pathname.vi"("Input String"=w2022) -> ("path"=w2021:path)
                    n967 = call "Post_Process_Measurement.vi"("Raw data file"=w2021) -> ()  [unwired: 1 out]
                  }
                  frame Enabled {
                    n968 = call "Post_Process_Measurement.vi"("Channel Values"=w2028, "Raw data file"=w2030, "Channel Names"=w2029) -> ()  [unwired: 3 in]
                  }
                }
                n969 = local write "Process Point"(FALSE ("Kill Point")) -> ()
              }
              frame True {
                n970 = Strip Path(path=w2038) -> (name=w2033:string)  [unwired: 1 out]
                n971 = Strip Path(path=w2032) -> (name=w2031:string)  [unwired: 1 out]
                n972 = local read "nRows"() -> (w2043:i32)
                n973 = Format Into String(format string="Are you sure you want to remove the row in the results file \"%s\" generated from the raw data filename \"%s\"?", w2033, w2031) -> (resulting string=w2036:string)  [unwired: 2 in, 1 out]
                n974 = Less?(x=w2043, y=w2041) -> (x < y?=w2042:bool)
                n975 = Two Button Dialog(message=w2036) -> (T button?=w2035:bool)  [unwired: 2 out]
                n976 = case shown="True" w2042 {
                  tunnel: ["Create Selectors" "Initialise" ("t")] -> w2040
                  frame False {
                  }
                  frame True {
                  }
                }
                n977 = case shown="True" w2035 {
                  tunnel: w2038 -> [_ w2045]
                  tunnel: w2034 -> [_ w2044]
                  frame False {
                  }
                  frame True {
                    n978 = Build Array(w2044) -> (w2046:i32[])
                    n979 = call "Delete_unwanted_rows.vi"("Selected Rows"=w2046, "Filename"=w2045) -> ()  [unwired: 1 out]
                  }
                }
                n980 = local write "Kill Point"(FALSE ("Kill Point")) -> ()
              }
            }
          }
        }
      }
      frame "Edit template file" {
        n981 = stacked-sequence {
          frame #0 {
            n982 = local read "Template"() -> (w2055:path)
            n983 = call "Valid_Path.vi"("Filename"=w2055) -> ("Valid Path?"=w2054:bool)
            n984 = case shown="False" w2054 {
              tunnel: [T11."Edit Existing Template File" ("Mode") T11."Create New Template File" ("Mode")] -> w2058
              frame True {
              }
              frame False {
              }
            }
            n985 = local read "Results file"() -> (w2057:path)
            n986 = call "Edit_Template_File.vi"("Mode"=w2058, "Template Filename"=w2055, "Data Filename"=w2057) -> ("Template Filename Out"=w2056:path)  [unwired: 12 out]
            n987 = local write "Template"(w2056) -> ()
          }
          frame #1 {
            n988 = local read "Job Directory"() -> (w2061:path)
            n989 = Path To String(path=w2061) -> (string=w2064:string)
            n990 = call "Read_Write_Template.vi"("Mode"=Global_mode."Write Global to File", "Single Value In"=w2064, "Data type"="Log Folder Name" ("Variable name")) -> ()  [unwired: 5 in, 8 out]
            n991 = local write "Edit Template File"(FALSE ("Edit Template File")) -> ()
            n992 = Current VI's Path() -> (path=w2067:path)
            n993 = call "Open_Close_Front_Panel.ph.vi"("Front Panel Window:Open"=TRUE, "VI path"=w2067) -> ()  [unwired: 2 out]
          }
        }
      }
      frame "Save Plot Data" {
        n994 = global read "Results_plotter_Global.vi" "XY Graph Cluster"() -> (w2068:cluster{dbl[], dbl[]}[])
        n995 = local read "Tolerances"() -> (w2075:dbl[])
        n996 = local read "Absisca"() -> (w2074:u16)
        n997 = local read "Transpose"() -> (w2073:bool)
        n998 = local read "Multi Ordinate"() -> (w2072:i32[])
        n999 = global read "Results_plotter_Global.vi" "Precision"() -> (w2069:string[])
        n1000 = stacked-sequence {
          seq-local: [w2086 _ _ _ _ _ _ _ _] -> [_ w2111 _ w2149 _ _ _ _ _]
          seq-local: [_ w2107 _ _ _ _ _ _ _] -> [_ _ _ _ _ _ _ w2271 _]
          seq-local: [_ _ _ _ _ w2201 _ _ _] -> [_ _ _ _ _ _ _ w2270 _]
          seq-local: [_ _ _ _ _ w2203 _ _ _] -> [_ _ _ _ _ _ w2239 _ _]
          seq-local: [_ _ _ w2147 _ _ _ _ _] -> [_ _ _ _ _ _ w2240 _ _]
          seq-local: [_ _ _ _ w2170 _ _ _ _] -> [_ _ _ _ _ w2196 _ _ _]
          seq-local: [w2083 _ _ _ _ _ _ _ _] -> [_ _ _ _ _ _ _ _ w2276]
          seq-local: [w2082 _ _ _ _ _ _ _ _] -> [_ w2099 _ _ _ _ _ _ _]
          seq-local: [_ _ w2128 _ _ _ _ _ _] -> [_ _ _ w2148 _ _ w2241 _ _]
          seq-local: [_ _ _ _ _ _ w2237 _ _] -> [_ _ _ _ _ _ _ w2268 _]
          tunnel: [_ _ _ _ _ _ _ _ TRUE] -> w2081
          tunnel: [_ _ _ _ _ _ _ _ w2274] -> w2080
          tunnel: w2078 -> [_ _ _ _ _ w2199 _ _ _]
          tunnel: w2079 -> [_ w2104 _ _ _ w2202 _ _ _]
          tunnel: [_ _ _ _ _ w2202 _ _ _] -> w2077
          tunnel: [_ _ _ _ _ w2199 _ _ _] -> w2076
          tunnel: w2075 -> [w2088 _ _ _ w2175 w2200 _ _ _]
          tunnel: w2068 -> [w2087 _ _ w2151 _ _ _ _ _]
          tunnel: w2074 -> [w2085 w2121 _ _ w2177 _ _ _ _]
          tunnel: w2073 -> [w2084 _ _ w2150 _ _ _ _ _]
          tunnel: w2072 -> [_ _ _ _ w2174 _ _ _ _]
          tunnel: [_ _ _ w2145 _ _ _ _ _] -> w2071
          tunnel: w2070 -> [_ _ w2131 w2145 _ _ _ _ _]
          tunnel: w2069 -> [_ _ _ w2144 _ w2195 _ _ _]
          frame #0 {
            n1001 = local read "Save Surface Fit"() -> (w2083:bool)
            n1002 = Not(x=w2084) -> (.not. x?=w2091:bool)
            n1003 = for {
              tunnel: w2087 -> [w2098] mode=indexing
              tunnel: w2091 -> [w2095]
              shift-right: [w2093] -> w2089
              shift-left: dbl[] [] -> [w2094]
              n1004 = Unbundle(w2098) -> (w2097:dbl[], w2096:dbl[])
              n1005 = Select(t=w2097, s=w2095, f=w2096) -> (s? t:f=w2092:dbl[])
              n1006 = Build Array (concatenate)(w2094, w2092) -> (w2093:dbl[])
            }
            n1007 = Index Array(array=w2088, index=w2085) -> (element=w2082:dbl)
            n1008 = call "Numeric_bins.vi"("Values"=w2089, "Tolerance"=w2082) -> ("Bin Centres"=w2086:dbl[])  [unwired: 2 out]
          }
          frame #1 {
            n1009 = Index Array(array=w2104, index=w2121) -> (element=w2124:string)
            n1010 = Match Pattern(string=w2124, regular expression=":") -> (before substring=w2123:string, after substring=w2122:string)  [unwired: 3 out]
            n1011 = Concatenate Strings(w2123, " ", w2122, " =:" ("regular expression")) -> (w2106:string)
            n1012 = Greater?(x=w2099, y=0.4) -> (0:w2119:bool)
            n1013 = Greater?(x=w2099, y=0.09) -> (0:w2114:bool)
            n1014 = call <vilib>:"Trim Whitespace.vi"("string"=w2106) -> ("trimmed string"=w2105:string)  [unwired: 1 in]
            n1015 = Select(t=i16 0 ("precision (6)"), s=w2119, f=i16 2 ("precision (6)")) -> (s? t:f=w2115:i16)
            n1016 = Select(t=w2115, s=w2114, f=i16 3) -> (s? t:f=w2112:i16)
            n1017 = Number To Fractional String(number=w2111, precision (6)=w2112) -> (F-format string=w2110:string[])  [unwired: 2 out]
            n1018 = for {
              tunnel: w2105 -> [w2127]
              tunnel: w2110 -> [w2125] mode=indexing
              tunnel: [w2126] -> w2109 mode=indexing
              n1019 = Concatenate Strings(w2127, w2125) -> (w2126:string)
            }
            n1020 = Build Array (concatenate)("Plot:Legend:" ("Input Element"), w2109, "End of:Plot Series:" ("Input Element")) -> (w2107:string[])
          }
          frame #2 {
            n1021 = local read "Multi Ordinate?"() -> (w2130:bool)
            n1022 = global read "Results_plotter_Global.vi" "Legend"() -> (w2129:string[])
            n1023 = case shown="False" w2130 {
              tunnel: w2131 -> [w2135 _]
              tunnel: [w2132 w2143] -> w2128
              tunnel: w2129 -> [w2134 w2143]
              frame False {
                n1024 = local read "Multi Ordinate"() -> (w2138:i32[])
                n1025 = Index Array(array=w2138, index=0 ("Index")) -> (element=w2136:i32)
                n1026 = Index Array(array=w2135, index=w2136) -> (element=w2133:string)
                n1027 = for {
                  tunnel: w2134 -> [w2142] mode=indexing
                  tunnel: w2133 -> [w2141]
                  tunnel: [w2139] -> w2132 mode=indexing
                  n1028 = Format Into String(format string="; %s", initial string=w2141, w2142) -> (resulting string=w2139:string)  [unwired: 1 in, 1 out]
                }
              }
              frame True {
              }
            }
          }
          frame #3 {
            n1029 = call "Grid_Data.vi"("Transpose"=w2150, "XY Graph"=w2151, "Bin Centres"=w2149) -> ("Grided data"=w2146:dbl[][])  [unwired: 1 out]
            n1030 = for {
              tunnel: w2148 -> [w2158] mode=indexing
              tunnel: [w2160] -> w2147 mode=indexing
              tunnel: w2146 -> [w2159] mode=indexing
              tunnel: w2145 -> [w2154]
              tunnel: w2144 -> [w2153]
              n1031 = Match Pattern(string=w2158, regular expression=";") -> (before substring=w2155:string)  [unwired: 4 out]
              n1032 = Search 1D Array(1D array=w2154, element=w2155) -> (index of element=w2156:i32)  [unwired: 1 out]
              n1033 = Index Array(array=w2153, index=w2156) -> (element=w2152:string)
              n1034 = for {
                tunnel: w2152 -> [w2165]
                tunnel: [w2164] -> w2161 mode=indexing
                tunnel: w2159 -> [w2162] mode=indexing
                n1035 = Not A Number/Path/Refnum?(number/path/refnum=w2162) -> (NaN/Path/Refnum?=w2163:bool)
                n1036 = case shown="True" w2163 {
                  tunnel: w2165 -> [w2168 _]
                  tunnel: [w2167 ""] -> w2164
                  tunnel: w2162 -> [w2166 _]
                  frame False {
                    n1037 = call "Number_2_string.vi"("precision"=w2168, "number"=w2166) -> ("String"=w2167:string)
                  }
                  frame True {
                  }
                }
              }
              n1038 = Build Array (concatenate)(w2158, w2161) -> (w2160:string[])
            }
          }
          frame #4 {
            n1039 = Index Array(array=w2174, index=0 ("Index")) -> (element=w2172:i32)
            n1040 = global read "Results_plotter_Global.vi" "Summarise"() -> (w2171:string[])
            n1041 = for {
              shift-right: [w2184] -> w2170
              shift-left: i32[] [] -> [w2185]
              tunnel: w2177 -> [w2190]
              tunnel: w2172 -> [w2189]
              tunnel: w2175 -> [w2182] mode=indexing
              tunnel: w2171 -> [w2180] mode=indexing
              i -> [w2183]
              n1042 = Equal?(x=w2189, y=w2183) -> (x = y?=w2188:bool)
              n1043 = Not A Number/Path/Refnum?(number/path/refnum=w2182) -> (NaN/Path/Refnum?=w2181:bool)
              n1044 = Equal?(x=w2190, y=w2183) -> (x = y?=w2187:bool)
              n1045 = Equal?(x="FALSE", y=w2180) -> (x = y?=w2178:bool)
              n1046 = Compound Arithmetic op=OR(w2187, w2188, w2181, w2178) -> (w2186:bool)
              n1047 = case shown="False" w2186 {
                tunnel: w2185 -> [w2193 w2194]
                tunnel: [w2192 w2194] -> w2184
                tunnel: w2183 -> [w2191 _]
                frame False {
                  n1048 = Build Array (concatenate)(w2193, w2191) -> (w2192:i32[])
                }
                frame True {
                }
              }
            }
          }
          frame #5 {
            n1049 = local read "Plotted Series"() -> (w2198:bool[][])
            n1050 = for {
              tunnel: w2200 -> [w2214]
              tunnel: [w2213] -> w2203 mode=indexing
              tunnel: w2196 -> [w2212]
              tunnel: w2199 -> [w2211]
              tunnel: w2198 -> [w2210] mode=indexing
              tunnel: i32[] [] -> [w2208]
              tunnel: w2195 -> [w2207]
              n1051 = for {
                shift-right: [w2216] -> w2209
                shift-left: w2208 -> [w2217]
                tunnel: w2210 -> [w2215] mode=indexing
                i -> [w2218]
                n1052 = case shown="True" w2215 {
                  tunnel: w2218 -> [_ w2222]
                  tunnel: w2217 -> [w2219 w2221]
                  tunnel: [w2219 w2220] -> w2216
                  frame False {
                  }
                  frame True {
                    n1053 = Build Array (concatenate)(w2221, w2222) -> (w2220:i32[])
                  }
                }
              }
              n1054 = for {
                tunnel: w2214 -> [w2230]
                tunnel: [w2231] -> w2213 mode=indexing
                tunnel: w2212 -> [w2225] mode=indexing
                tunnel: w2211 -> [w2228]
                tunnel: w2209 -> [w2227]
                tunnel: w2207 -> [w2224]
                n1055 = for {
                  tunnel: w2227 -> [w2236] mode=indexing
                  tunnel: [w2235] -> w2232 mode=indexing
                  tunnel: w2225 -> [w2234]
                  tunnel: w2228 -> [w2233]
                  n1056 = Index Array(array=w2233, index (row)=w2236, index (col)=w2234) -> (element=w2235:string)
                }
                n1057 = Index Array(array=w2224, index=w2225) -> (element=w2226:string)
                n1058 = Index Array(array=w2230, index=w2225) -> (element=w2229:dbl)
                n1059 = call "Value_Occurence_Analysis.vi"("Average Numeric Values?"=FALSE, "Tolerance"=w2229, "Precision (3)"=w2226, "String Array"=w2232) -> ("Output String"=w2231:string)  [unwired: 2 out]
              }
            }
            n1060 = for {
              tunnel: w2196 -> [w2206] mode=indexing
              tunnel: w2202 -> [w2205]
              tunnel: [w2204] -> w2201 mode=indexing
              n1061 = Index Array(array=w2205, index=w2206) -> (element=w2204:string)
            }
          }
          frame #6 {
            n1062 = for {
              shift-right: [w2254] -> w2237
              shift-left: string[][] [] -> [w2255]
              shift-right: [w2250] -> _
              shift-left: _ -> [w2251]
              tunnel: w2241 -> [w2252] mode=indexing
              tunnel: w2240 -> [w2244] mode=indexing
              tunnel: w2239 -> [w2243] mode=indexing
              i -> [w2249]
              n1063 = Greater Than 0?(x=w2249) -> (x > 0?=w2248:bool)
              n1064 = Match Pattern(string=w2252, regular expression="; ") -> (before substring=w2250:string)  [unwired: 4 out]
              n1065 = Equal?(x=w2251, y=w2250) -> (x = y?=w2247:bool)
              n1066 = Build Array (concatenate)(w2244, "", w2243) -> (w2242:string[])
              n1067 = Compound Arithmetic op=AND(w2248, invert w2247) -> (w2246:bool)
              n1068 = case shown="True" w2246 {
                tunnel: w2255 -> [w2259 w2262]
                tunnel: [w2258 w2261] -> w2254
                tunnel: w2242 -> [w2257 w2260]
                frame True {
                  n1069 = Build Array (concatenate)(w2259, string[] [] ("array"), w2257) -> (w2258:string[][])
                }
                frame False {
                  n1070 = Build Array (concatenate)(w2262, w2260) -> (w2261:string[][])
                }
              }
            }
          }
          frame #7 {
            w2267 = TRUE  # Simple Save?
            n1071 = Build Array (concatenate)(w2271, w2270) -> (w2269:string[])
            n1072 = local read "Header"() -> (w2264:string)
            n1073 = call "Write_output_file.vi"("Output filename"="Output Filename", "Header"=w2264, "Channel Names"=w2269, "Data"=w2268, "Simple Save?"=w2267, "Summarise mode"=T12."No data summary") -> ("Output filename Out"=w2265:path)  [unwired: 6 in, 3 out]
            n1074 = local write "Output Filename"(w2265) -> ()
          }
          frame #8 {
            n1075 = local write "Save Plot data"(FALSE ("Save Plot data")) -> ()
            n1076 = local write "Header"("") -> ()
            n1077 = Select(t="Save Surface Fit data", s=w2276, f="Create Selectors") -> (s? t:f=w2274:string)
          }
        }
      }
      frame "What type of row averaging?" {
        n1078 = Two Button Dialog(message="Do you want to Combine rows with identical positions together?", 1:"Average Points in Series" ("F button name (\"Cancel\")"), 2:"Combine rows" ("T button name (\"OK\")")) -> (T button?=w2282:bool)
        n1079 = Select(t="Combine rows" ("T button name (\"OK\")"), s=w2282, f="Average Rows together") -> (s? t:f=w2279:string)
      }
      frame "Combine rows" {
        w2292 = TRUE  # Show panel ?
        n1080 = local read "Output Filename"() -> (w2291:path)
        n1081 = call "Combined_file_Panel.vi"("Show panel ?"=w2292, "Output filename"=w2291) -> ("Only Plotted data?"=w2293:bool, "Include Empty Rows? Out"=w2294:bool, "Give Audit Channels Out"=w2295:bool, "Output filename Out"=w2290:path)  [unwired: 5 out]
        n1082 = case shown="True" w2293 {
          tunnel: w2297 -> [w2306 w2309]
          tunnel: [w2306 w2307] -> w2296
          frame False {
          }
          frame True {
            n1083 = global read "Results_plotter_Global.vi" "Plot Index values"() -> (w2311:dbl[][])
            n1084 = Index Array(array=w2311, index (row)=2) -> (element=w2308:dbl[])  [unwired: 1 in]
            n1085 = for {
              tunnel: w2309 -> [w2314]
              tunnel: w2308 -> [w2313] mode=indexing
              tunnel: [w2312] -> w2307 mode=indexing
              n1086 = Index Array(array=w2314, index (row)=w2313) -> (element=w2312:string[])  [unwired: 1 in]
            }
          }
        }
        n1087 = local write "Save Averaged rows"(FALSE ("Save Plot data")) -> ()
        n1088 = local read "X Ch Name"() -> (w2301:u16)
        n1089 = local read "Y Ch Name"() -> (w2302:u16)
        n1090 = local read "Z Ch Name"() -> (w2303:u16)
        n1091 = call "Find_Rows_to_Combine.vi"("Include Empty Rows?"=w2294, "file path (dialog if empty)"=w2290, "Give Audit Channels"=w2295, "Full Channel Names"=w2300, "Data"=w2296, "Z Column Index"=w2303, "Y Column Index"=w2302, "X Column Index"=w2301) -> ()  [unwired: 4 out]
        n1092 = local write "Output Filename"(w2290) -> ()
      }
      frame "Average Rows together" {
        n1093 = local read "Tolerances"() -> (w2316:dbl[])
        n1094 = global read "Results_plotter_Global.vi" "XY Graph Cluster"() -> (w2318:cluster{dbl[], dbl[]}[])
        n1095 = local read "Absisca"() -> (w2315:u16)
        n1096 = local read "Transpose"() -> (w2321:bool)
        n1097 = global read "Results_plotter_Global.vi" "Summarise"() -> (w2319:string[])
        n1098 = stacked-sequence {
          seq-local: [_ w2347 _ _] -> [_ _ w2372 _]
          seq-local: [w2328 _ _ _] -> [_ _ w2371 _]
          tunnel: [_ _ _ TRUE] -> w2327
          tunnel: [_ _ _ "Create Selectors"] -> w2326
          tunnel: w2324 -> [_ w2350 _ w2397]
          tunnel: w2325 -> [w2329 _ _ w2396]
          tunnel: [_ _ _ w2396] -> w2323
          tunnel: [_ _ _ w2397] -> w2322
          tunnel: w2318 -> [_ w2353 _ _]
          tunnel: w2321 -> [_ w2352 _ _]
          tunnel: w2320 -> [_ w2351 _ _]
          tunnel: w2319 -> [w2330 _ _ _]
          tunnel: [_ w2351 _ _] -> w2317
          tunnel: w2316 -> [_ w2349 _ _]
          tunnel: w2315 -> [_ w2348 _ _]
          frame #0 {
            n1099 = for {
              tunnel: w2330 -> [w2335] mode=indexing
              shift-right: [w2331] -> w2328
              shift-left: w2329 -> [w2332]
              tunnel: w2329 -> [w2333] mode=indexing
              n1100 = Equal?(x="TRUE", y=w2335) -> (x = y?=w2334:bool)
              n1101 = case shown="False" w2334 {
                tunnel: w2333 -> [w2341 _]
                tunnel: w2332 -> [w2338 w2342]
                tunnel: [w2337 w2342] -> w2331
                frame False {
                  n1102 = Concatenate Strings(w2341, "St Dev") -> (w2339:string)
                  n1103 = Build Array (concatenate)(w2338, w2339) -> (w2337:string[])
                }
                frame True {
                }
              }
            }
          }
          frame #1 {
            n1104 = Not(x=w2352) -> (.not. x?=w2354:bool)
            n1105 = global read "Results_plotter_Global.vi" "Plot Index values"() -> (w2345:dbl[][])
            n1106 = Index Array(array=w2345, index (row)=2) -> (element=w2344:dbl[])  [unwired: 1 in]
            n1107 = for {
              tunnel: w2353 -> [w2368] mode=indexing
              tunnel: w2354 -> [w2365]
              tunnel: w2350 -> [w2364]
              tunnel: w2349 -> [w2363]
              tunnel: w2348 -> [w2362]
              tunnel: [w2361] -> w2347 mode=concatenating
              shift-right: [w2358] -> _
              shift-left: 0 -> [w2356]
              tunnel: w2344 -> [w2360]
              n1108 = Unbundle(w2368) -> (w2367:dbl[], w2366:dbl[])
              n1109 = Select(t=w2367, s=w2365, f=w2366) -> (s? t:f=w2359:dbl[])
              n1110 = Array Subset(array=w2360, index=w2356) -> (w2355:dbl[])  [unwired: 1 in]
              n1111 = call "Produce_averaged_Rows.vi"("Absisca"=w2362, "Row numbers"=w2355, "Tolerances"=w2363, "Array in"=w2359, "Data"=w2364) -> ("Array out"=w2361:string[][])  [unwired: 6 in]
              n1112 = Array Size(array=w2359) -> (size(s)=w2357:i32)
              n1113 = Add(x=w2357, y=w2356) -> (x+y=w2358:i32)
            }
          }
          frame #2 {
            n1114 = local read "Output Filename"() -> (w2370:path)
            n1115 = call "Does_file_exist_(simple).vi"("Pathname"=w2370) -> ("exists?"=w2369:bool)
            n1116 = case shown="False" w2369 {
              tunnel: w2372 -> [w2375 w2383]
              tunnel: w2371 -> [w2378 w2384]
              tunnel: w2370 -> [w2376 w2385]
              frame False {
                w2379 = FALSE  # Save Plotted rows only?
                w2381 = TRUE  # Simple Save?
                n1117 = Build Array (concatenate)(string[] [] ("array"), w2375) -> (w2374:string[][])
                n1118 = local read "Template"() -> (w2380:path)
                n1119 = call "Write_output_file.vi"("Output filename"=w2376, "Template Filename"=w2380, "Channel Names"=w2378, "Data"=w2374, "Simple Save?"=w2381, "Save Plotted rows only?"=w2379, "Summarise mode"=T12."No data summary") -> ("Output filename Out"=w2382:path)  [unwired: 5 in, 3 out]
                n1120 = local write "Output Filename"(w2382) -> ()
              }
              frame True {
                w2388 = FALSE  # Present Channels only
                w2390 = TRUE  # exists?
                n1121 = call "Check_and_rewrite_file.vi"("Filename"=w2385, "Present Channels only"=w2388, "Present Channels"=w2384) -> ("Merged Channels"=w2389:string[], "Merged?"=w2387:bool)  [unwired: 1 in, 10 out]
                n1122 = case shown="True" w2387 {
                  tunnel: w2383 -> [w2391 w2393]
                  tunnel: w2384 -> [_ w2394]
                  tunnel: [w2391 w2392] -> w2386
                  tunnel: w2389 -> [_ w2395]
                  frame False {
                  }
                  frame True {
                    n1123 = call "Merge_2D_values.vi"("Values In"=w2393, "Present Channels"=w2394, "Desired Channels"=w2395) -> ("Values Out"=w2392:string[][])
                  }
                }
                n1124 = call "Write_Ch_data_file.vi"("exists?"=w2390, "Channel Values"=w2386, "Channel names"=w2389, "Filename"=w2385) -> ()  [unwired: 4 in, 4 out]
              }
            }
          }
          frame #3 {
            n1125 = local write "Save Averaged rows"(FALSE ("Save Plot data")) -> ()
          }
        }
      }
      frame "Save Surface Fit data" {
        n1126 = local read "Transpose"() -> (w2401:bool)
        n1127 = local read "Tolerances"() -> (w2408:dbl[])
        n1128 = local read "Absisca"() -> (w2407:u16)
        n1129 = global read "Results_plotter_Global.vi" "Precision"() -> (w2404:string[])
        n1130 = stacked-sequence {
          seq-local: [w2415 _ _ _ _ _] -> [_ w2434 _ _ _ _]
          seq-local: [_ w2431 _ _ _ _] -> [_ _ _ _ w2518 _]
          seq-local: [_ _ w2457 _ _ _] -> [_ _ _ _ w2537 _]
          seq-local: [w2416 _ _ _ _ _] -> [_ _ w2458 _ _ _]
          seq-local: [_ _ w2453 _ _ _] -> [_ _ _ _ w2521 _]
          seq-local: [_ _ w2452 _ _ _] -> [_ _ _ w2488 _ _]
          seq-local: [_ _ _ w2483 _ _] -> [_ _ _ _ w2519 _]
          tunnel: [_ _ _ _ _ TRUE] -> w2412
          tunnel: [_ _ _ _ _ "Create Selectors"] -> w2411
          tunnel: w2409 -> [_ _ _ _ _ w2543]
          tunnel: w2410 -> [_ w2419 _ _ _ w2544]
          tunnel: w2408 -> [_ w2445 _ _ _ _]
          tunnel: w2407 -> [_ w2446 _ _ _ _]
          tunnel: [_ _ w2463 _ _ _] -> w2406
          tunnel: w2405 -> [_ w2422 w2463 _ _ _]
          tunnel: w2404 -> [_ _ w2459 _ _ _]
          tunnel: [_ _ _ _ _ w2544] -> w2403
          tunnel: [_ _ _ _ _ w2543] -> w2402
          tunnel: w2401 -> [_ _ _ w2482 _ _]
          frame #0 {
            n1131 = global read "Results_plotter_Global.vi" "X Values"() -> (w2415:dbl[])
            n1132 = global read "Results_plotter_Global.vi" "Raw Interpolation"() -> (w2413:dbl[][])
            n1133 = global read "Results_plotter_Global.vi" "Y Values"() -> (w2414:dbl[])
            n1134 = Insert Into Array(array=w2413, index (col)=0 ("disabled index (col)"), new element=w2414) -> (w2416:dbl[][])  [unwired: 1 in]
          }
          frame #1 {
            n1135 = global read "Results_plotter_Global.vi" "Y Axis Name"() -> (w2421:string)
            n1136 = Search 1D Array(1D array=w2422, element=w2421) -> (index of element=w2420:i32)  [unwired: 1 out]
            n1137 = Index Array(array=w2419, index=w2420) -> (element=w2418:string)
            n1138 = Match Pattern(string=w2418, regular expression=":") -> (before substring=w2448:string, after substring=w2447:string)  [unwired: 3 out]
            n1139 = Index Array(array=w2445, index=w2446) -> (element=w2436:dbl)
            n1140 = Concatenate Strings(w2448, " ", w2447, " =:" ("regular expression")) -> (w2430:string)
            n1141 = Greater?(x=w2436, y=0.9) -> (0:w2443:bool)
            n1142 = Greater?(x=w2436, y=0.09) -> (0:w2438:bool)
            n1143 = call <vilib>:"Trim Whitespace.vi"("string"=w2430) -> ("trimmed string"=w2429:string)  [unwired: 1 in]
            n1144 = Select(t=i16 0 ("precision (6)"), s=w2443, f=i16 2 ("precision (6)")) -> (s? t:f=w2439:i16)
            n1145 = Select(t=w2439, s=w2438, f=i16 3) -> (s? t:f=w2435:i16)
            n1146 = Number To Fractional String(number=w2434, precision (6)=w2435) -> (F-format string=w2433:string[])  [unwired: 2 out]
            n1147 = for {
              tunnel: w2429 -> [w2451]
              tunnel: w2433 -> [w2449] mode=indexing
              tunnel: [w2450] -> w2424 mode=indexing
              n1148 = Concatenate Strings(w2451, w2449) -> (w2450:string)
            }
            n1149 = Build Array (concatenate)("Channel:Values:Plotted" ("Input Element"), "Axis:Name:" ("Input Element"), "Axis:Values:" ("Input Element"), w2424) -> (w2431:string[])
          }
          frame #2 {
            n1150 = global read "Results_plotter_Global.vi" "X Axis Name"() -> (w2456:string)
            n1151 = Concatenate Strings(w2456, " =" ("string")) -> (w2454:string)
            n1152 = local read "Multi Ordinate"() -> (w2462:i32[])
            n1153 = Index Array(array=w2462, index=0 ("Index")) -> (element=w2460:i32)
            n1154 = Index Array(array=w2459, index=w2460) -> (element=w2452:string)
            n1155 = Index Array(array=w2463, index=w2460) -> (element=w2453:string)
            n1156 = for {
              tunnel: w2453 -> [w2465]
              tunnel: [w2468] -> w2457 mode=indexing
              tunnel: w2452 -> [w2467]
              tunnel: w2458 -> [w2466] mode=indexing
              tunnel: w2454 -> [w2464]
              n1157 = for {
                tunnel: w2466 -> [w2471] mode=indexing
                tunnel: [w2470] -> w2469 mode=indexing
                tunnel: w2467 -> [w2473]
                n1158 = Not A Number/Path/Refnum?(number/path/refnum=w2471) -> (NaN/Path/Refnum?=w2472:bool)
                n1159 = case shown="False" w2472 {
                  tunnel: w2473 -> [w2476 _]
                  tunnel: w2471 -> [w2475 _]
                  tunnel: [w2474 ""] -> w2470
                  frame False {
                    n1160 = call "Number_2_string.vi"("precision"=w2476, "number"=w2475) -> ("String"=w2474:string)
                  }
                  frame True {
                  }
                }
              }
              n1161 = Build Array (concatenate)(w2465, w2464, w2469) -> (w2468:string[])
            }
          }
          frame #3 {
            w2487 = "\t"
            n1162 = global read "Results_plotter_Global.vi" "Intensity Plot data in rows"() -> (w2489:dbl[][])
            n1163 = global read "Results_plotter_Global.vi" "Value plotted Name"() -> (w2486:string)
            n1164 = global read "Results_plotter_Global.vi" "X Axis Name"() -> (w2480:string)
            n1165 = global read "Results_plotter_Global.vi" "Y Axis Name"() -> (w2479:string)
            n1166 = case shown="False" w2482 {
              tunnel: [w2490 w2493] -> w2481
              tunnel: w2480 -> [w2491 w2493]
              tunnel: w2479 -> [w2490 w2492]
              tunnel: [w2491 w2492] -> w2478
              frame False {
              }
              frame True {
              }
            }
            n1167 = Concatenate Strings(w2481, w2487, w2478, w2487, w2486, "\r\n") -> (w2484:string)
            n1168 = for {
              tunnel: w2489 -> [w2499] mode=indexing
              tunnel: w2488 -> [w2504]
              shift-right: [w2498] -> w2483
              shift-left: w2484 -> [w2503]
              n1169 = Index Array(array=w2499, index=0) -> (element=w2495:dbl)
              n1170 = Index Array(array=w2499, index=1) -> (element=w2494:dbl)
              n1171 = Index Array(array=w2499, index=2) -> (element=w2497:dbl)
              n1172 = Not A Number/Path/Refnum?(number/path/refnum=w2497) -> (NaN/Path/Refnum?=w2496:bool)
              n1173 = case shown="False" w2496 {
                tunnel: w2504 -> [w2515 _]
                tunnel: w2503 -> [w2514 w2516]
                tunnel: w2497 -> [w2513 _]
                tunnel: [w2512 w2516] -> w2498
                tunnel: w2495 -> [w2511 _]
                tunnel: w2494 -> [w2510 _]
                frame False {
                  w2506 = "\t"
                  n1174 = call "Number_2_string.vi"("number"=w2511) -> ("String"=w2509:string)  [unwired: 1 in]
                  n1175 = call "Number_2_string.vi"("number"=w2510) -> ("String"=w2508:string)  [unwired: 1 in]
                  n1176 = call "Number_2_string.vi"("precision"=w2515, "number"=w2513) -> ("String"=w2507:string)
                  n1177 = Concatenate Strings(w2514, w2509, w2506, w2508, w2506, w2507, "\r\n") -> (w2512:string)
                }
                frame True {
                }
              }
            }
          }
          frame #4 {
            w2533 = TRUE  # append to file? (new file:F)
            n1178 = global read "Results_plotter_Global.vi" "Surface Integral"() -> (w2532:dbl)
            n1179 = global read "Results_plotter_Global.vi" "Surface Area"() -> (w2531:dbl)
            n1180 = Initialize Array("", 10 ("Dimension Size")) -> (w2542:string[])
            n1181 = Divide(x=w2532, y=w2531) -> (x/y=w2530:dbl)
            n1182 = call "Asterisk_header.vi"("Channel names"=w2542) -> ("Header string"=w2520:string)
            n1183 = call "Value_to_string.vi"("Value"=w2532, "Label for value"="Surface Integral") -> ("Output string"=w2527:string)  [unwired: 1 in]
            n1184 = call "Value_to_string.vi"("Value"=w2531, "Label for value"="Surface Area") -> ("Output string"=w2528:string)  [unwired: 1 in]
            n1185 = call "Value_to_string.vi"("Value"=w2530, "Label for value"="Surface Average") -> ("Output string"=w2526:string)  [unwired: 1 in]
            n1186 = Concatenate Strings(w2528, w2527, w2526) -> (w2523:string)
            n1187 = call "Ch_names_to_rows.vi"("Channel Names"=w2518) -> ("3 Row names"=w2517:string[][])
            n1188 = local read "Output Filename"() -> (w2534:path)
            n1189 = Build Array (concatenate)(w2517, w2537) -> (w2535:string[][])
            n1190 = Array To Spreadsheet String(array=w2535, 3:"%s" ("format string")) -> (spreadsheet string=w2522:string)  [unwired: 1 out]
            n1191 = Format Into String(format string="\n%s\n\n%s\n%s\n\n\nInterpolated Surface of %s\n%s\n%s\n%s\n\n\n%s", w2520, w2519, w2520, w2521, w2520, w2522, w2520, w2523) -> (resulting string=w2525:string)  [unwired: 2 in, 1 out]
            n1192 = call "Write_Characters_To_File.vi"("file path (dialog if empty)"=w2534, "character string"=w2525, "append to file? (new file:F)"=w2533) -> ()  [unwired: 2 in, 4 out]
          }
          frame #5 {
            n1193 = local write "Save Surface Fit"(FALSE ("Save Plot data")) -> ()
          }
        }
      }
      frame "Save Data in Rows" {
        w2559 = TRUE  # Show panel ?
        n1194 = local read "Output Filename"() -> (w2556:path)
        n1195 = local write "Save Data in Rows"(FALSE ("Save All data")) -> ()
        n1196 = call "Output_file_Panel.vi"("Show panel ?"=w2559, "Channel Names"=w2554, "Header"="Header", "Output filename"=w2556) -> ("Save Full Res Data?"=w2551:bool, "Desired Columns"=w2560:i32[], "Header Out"=w2558:string, "Output filename Out"=w2562:path, "Channels to Tabulate in header Out"=w2548:i32[], "Save Plotted rows only?"=w2549:bool, "Summarise mode"=w2557:T12, "Grouping info"=w2550:T20[])
        "Plotted rows only?" <- w2549
        n1197 = case shown="False" w2551 {
          tunnel: w2562 -> [w2578 w2580]
          tunnel: w2560 -> [w2577 _]
          tunnel: w2558 -> [w2576 _]
          tunnel: w2549 -> [w2575 _]
          tunnel: w2557 -> [w2574 _]
          tunnel: w2555 -> [w2573 _]
          tunnel: w2554 -> [w2572 _]
          tunnel: [w2571 w2580] -> w2553
          tunnel: ["Create Selectors" "Is Filename Empty?"] -> w2552
          tunnel: w2550 -> [w2567 _]
          tunnel: w2548 -> [w2566 _]
          frame False {
            w2569 = FALSE  # Simple Save?
            n1198 = local read "Template"() -> (w2570:path)
            n1199 = call "Write_output_file.vi"("Output filename"=w2578, "Header"=w2576, "Template Filename"=w2570, "Channel Names"=w2572, "Data"=w2573, "Desired Columns"=w2577, "Simple Save?"=w2569, "Save Plotted rows only?"=w2575, "Summarise mode"=w2574, "Grouping info"=w2567, "Channels to Tabulate in header"=w2566) -> ("Output filename Out"=w2571:path)  [unwired: 1 in, 3 out]
          }
          frame True {
            "Mode" <- Plotter_Mode."Save file" ("Mode")
          }
        }
        n1200 = local write "Output Filename"(w2553) -> ()
      }
      frame "Is Filename Empty?" {
        # "This Express VI is the reason we can't strip object code from ResultsFilePlotter; may be able to convert to standard VI"
        n1201 = call "File Dialog"("start path"="Full_Res_Results_Folder", "prompt"="Please select a new or existing folder to save the results files in") -> ("selected path"=w2584:path, "cancelled"=w2582:bool)  [unwired: 5 in, 7 out]
        n1202 = local write "Full_Res_Results_Folder"(w2584) -> ()
        n1203 = case shown="False" w2582 {
          tunnel: ["Full Res file manipulator" ("f") "Create Selectors" ("t")] -> w2586
          frame False {
          }
          frame True {
          }
        }
      }
      frame "Check for overwrite or append" {
        n1204 = local read "Output Filename"() -> (w2600:path)
        n1205 = Format Into String(format string="Do you want to append to the result file\n\"%s\"" ("message"), w2600) -> (resulting string=w2595:string)  [unwired: 2 in, 1 out]
        n1206 = call <vilib>:"Three Button Dialog.vi"("Window Title (\"\")"="Output File Dialog" ("Window Title (\"\")"), "Right Button Text (\"Cancel\")"="Cancel" ("Button 3 Name"), "Center Button Text (\"No\")"="Overwrite" ("F button name (\"Cancel\")"), "Left Button Text (\"Yes\")"="Append" ("T button name (\"OK\")"), "message"=w2595) -> ("Which Button?"=w2594:T15)  [unwired: 6 out]
        n1207 = case shown="\"Center Button\"" w2594 {
          tunnel: w2600 -> [_ w2607 _]
          tunnel: ["Full Res file manipulator" "Full Res file manipulator" "Create Selectors" ("t")] -> w2593
          frame "Left Button" {
          }
          frame "Center Button" {
            n1208 = call "Delete_with_Check.vi"("FilePath"=w2607) -> ()  [unwired: 1 out]
          }
          frame "Right Button", Default {
          }
        }
      }
      frame "Create Plot summary" {
        w2610 = i32[] []
        w2622 = TRUE  # Summarise All
        n1209 = global read "Results_plotter_Global.vi" "Plot Index values"() -> (w2625:dbl[][])
        n1210 = local read "Intensity Plot?"() -> (w2621:bool)
        n1211 = global read "Results_plotter_Global.vi" "Row Reference"() -> (w2617:i32[][])
        n1212 = Index Array(array=w2617, index (col)=0 ("disabled index (col)")) -> (element=w2616:i32[])  [unwired: 1 in]
        n1213 = Index Array(array=w2625, index (row)=2) -> (element=w2627:dbl[])  [unwired: 1 in]
        n1214 = Select(t="Save Intensity plot as jpg", s=w2621, f="Save XY plot as jpg") -> (s? t:f=w2613:string)
        n1215 = To Long Integer(number=w2627) -> (32bit integer=w2624:i32[])
        n1216 = for {
          tunnel: w2632 -> [w2649]
          tunnel: [w2648] -> w2623 mode=indexing if=w2639
          tunnel: w2624 -> [w2638] mode=indexing
          tunnel: w2616 -> [w2647]
          shift-right: [w2644] -> w2615
          shift-left: w2610 -> [w2645]
          shift-right: [w2641] -> _
          shift-left: w2610 -> [w2640]
          n1217 = Search 1D Array(1D array=w2640, element=w2638) -> (index of element=w2642:i32)  [unwired: 1 out]
          n1218 = Index Array(array=w2647, index=w2638) -> (element=w2643:i32)
          n1219 = Search 1D Array(1D array=w2645, element=w2643) -> (index of element=w2646:i32)  [unwired: 1 out]
          n1220 = Index Array(array=w2649, index (row)=w2638) -> (element=w2648:string[])  [unwired: 1 in]
          n1221 = case shown="-1" w2642 {
            tunnel: w2638 -> [_ w2655]
            tunnel: w2640 -> [w2651 w2654]
            tunnel: [w2651 w2653] -> w2641
            tunnel: [FALSE TRUE] -> w2639
            frame 0, Default {
            }
            frame -1 {
              n1222 = Build Array (concatenate)(w2654, w2655) -> (w2653:i32[])
            }
          }
          n1223 = case shown="-1" w2646 {
            tunnel: w2643 -> [_ w2659]
            tunnel: w2645 -> [w2656 w2658]
            tunnel: [w2656 w2657] -> w2644
            frame 0, Default {
            }
            frame -1 {
              n1224 = Build Array (concatenate)(w2658, w2659) -> (w2657:i32[])
            }
          }
        }
        n1225 = local read "Result files to read"() -> (w2614:path[])
        n1226 = for {
          tunnel: w2615 -> [w2637] mode=indexing
          tunnel: w2614 -> [w2636]
          tunnel: [w2633] -> w2612 mode=indexing
          n1227 = Index Array(array=w2636, index=w2637) -> (element=w2635:path)
          n1228 = Strip Path(path=w2635) -> (name=w2634:string)  [unwired: 1 out]
          n1229 = call "Add_filename_suffix.vi"("Filename"=w2634) -> ("Base name"=w2633:string)  [unwired: 1 in, 3 out]
        }
        n1230 = call "Value_Occurence_Analysis.vi"("String Array"=w2612) -> ("Output String"=w2611:string)  [unwired: 3 in, 2 out]
        n1231 = global write "Results_plotter_Global.vi" "Current Data Filenames"(w2611) -> ()
        n1232 = call "Summarise.vi"("Channel Names"=w2628, "Data"=w2623, "Summarise All"=w2622) -> ("Summary"=w2630:string[][])  [unwired: 2 in]
        n1233 = global write "Results_plotter_Global.vi" "Plot Summary"(w2630) -> ()
      }
      frame "Save Intensity plot as jpg" {
        n1234 = local read "Job Directory"() -> (w2666:path)
        n1235 = global read "Constants_global.vi" "EnFlo SW Folder"() -> (w2668:path)
        n1236 = Build Path(base path=w2668, name or relative path=path "Anemometry/Anemometry Sub Vis/Data_plotting_vis/Intensity Plot Vis") -> (appended path=w2662:path)
        n1237 = call "Remote_call_prep.vi"("Vi Name in"="Create picture Vi Name", "Job Directory In"=w2666, "VI Directory"=w2662) -> ("Vi Name out"=w2664:string, "Job Directory out"=w2661:path, "cancelled"=w2660:bool)
        n1238 = local write "Create picture Vi Name"(w2664) -> ()
        n1239 = local write "Job Directory"(w2661) -> ()
        n1240 = Build Path(base path=w2662, name or relative path=w2664) -> (appended path=w2663:path)
        n1241 = case shown="False" w2660 {
          tunnel: w2663 -> [w2677 _]
          tunnel: w2661 -> [w2676 _]
          frame False {
            n1242 = Open VI Reference(type specifier VI Refnum (for type only)="type specifier VI Refnum (for type only)", vi path=w2677) -> (vi reference=w2682:refnum<vi>, error out=w2681:errorcluster)  [unwired: 2 in, 2 out]
            n1243 = property class="VI Interface Type 0"(reference=w2682, error in=w2681, "Front Panel Window:Open"=TRUE) -> (reference out=w2678:refnum<vi>, error out=w2679:errorcluster)
            n1244 = local read "Intensity Graph"() -> (w2685:dbl[][])
            n1245 = local read "No of Contours"() -> (w2675:i32)
            n1246 = call-by-ref "?"(reference=w2678, error in=w2679, "No of Contours"=w2675, "Job Directory"=w2676, "Intensity Graph"=w2685) -> (reference out=w2684:refnum<vi>, error out=w2683:errorcluster)  [unwired: 3 in]
            n1247 = Close Reference(reference=w2684, error in (no error)=w2683) -> ()  [unwired: 1 out]
          }
          frame True {
          }
        }
        n1248 = local write "Save Plot as jpg"(FALSE ("Save All data")) -> ()
      }
      frame "Run Calculation Routine" {
        n1249 = stacked-sequence {
          seq-local: [w2694 _ _] -> [_ w2704 _]
          seq-local: [w2693 _ _] -> [_ w2705 _]
          tunnel: [_ w2703 _] -> w2688
          tunnel: w2687 -> [_ _ _]
          frame #0 {
            n1250 = global read "Constants_global.vi" "EnFlo SW Folder"() -> (w2700:path)
            n1251 = local read "Job Directory"() -> (w2696:path)
            n1252 = Build Path(base path=w2700, name or relative path=path "Anemometry/Anemometry Sub Vis/Data_plotting_vis/Calculation Vis") -> (appended path=w2697:path)
            n1253 = call "Remote_call_prep.vi"("Vi Name in"="...using routine", "Job Directory In"=w2696, "VI Directory"=w2697) -> ("Vi Name out"=w2698:string, "Job Directory out"=w2695:path, "cancelled"=w2694:bool)
            n1254 = local write "Job Directory"(w2695) -> ()
            n1255 = local write "...using routine"(w2698) -> ()
            n1256 = Build Path(base path=w2697, name or relative path=w2698) -> (appended path=w2693:path)
          }
          frame #1 {
            n1257 = case shown="False" w2704 {
              tunnel: w2705 -> [w2713 _]
              tunnel: [w2709 w2726] -> w2703
              tunnel: "What to do next?" -> [w2708 w2726]
              frame False {
                n1258 = Open VI Reference(type specifier VI Refnum (for type only)="VI Refnum Calculation", vi path=w2713) -> (vi reference=w2719:refnum<vi>, error out=w2718:errorcluster)  [unwired: 1 in, 3 out]
                n1259 = property class="VI Interface Type 1"(reference=w2719, error in=w2718, "Front Panel Window:Open"=TRUE) -> (reference out=w2715:refnum<vi>, error out=w2716:errorcluster)
                n1260 = call-by-ref "?"(reference=w2715, error in=w2716) -> (reference out=w2721:refnum<vi>, error out=w2720:errorcluster, "New Values In"=w2706:string[][], "New Chs In"=w2714:string[])  [unwired: 2 in]
                n1261 = for {
                  tunnel: w2714 -> [w2724] mode=indexing
                  tunnel: [w2723] -> w2707 mode=indexing
                  n1262 = call "Check_Ch_Name_colons.vi"("No of Colons"=2, "Ch Name in"=w2724) -> ("Ch Name out"=w2723:string)
                }
                n1263 = Empty String/Path?(string/path=w2707) -> (empty?=w2711:bool[])
                n1264 = Or Array Elements(Boolean array=w2711) -> (logical OR=w2710:bool)
                n1265 = Close Reference(reference=w2721, error in (no error)=w2720) -> ()  [unwired: 1 out]
                n1266 = Select(t=w2708, s=w2710, f="Input calculated values") -> (s? t:f=w2709:string)
                n1267 = global write "Results_plotter_Global.vi" "New Values In"(w2706) -> ()
                n1268 = global write "Results_plotter_Global.vi" "New Chs In"(w2707) -> ()
              }
              frame True {
              }
            }
          }
          frame #2 {
            n1269 = local write "Edit Raw Data Header Info"(FALSE ("Raw DF in Orig Pos?")) -> ()
            n1270 = local write "Calculate new metadata"(FALSE ("Save All data")) -> ()
            n1271 = local write "Plotted rows only?"(TRUE ("Plotted rows only?")) -> ()
            n1272 = local write "Mode"(Plotter_Mode."Edit values per row" ("Mode")) -> ()
          }
        }
      }
      frame "Input calculated values" {
        n1273 = local read "Result files to read"() -> (w2735:path[])
        n1274 = stacked-sequence {
          seq-local: [w2739 _ _ _] -> [_ w2752 w2762 _]
          seq-local: [_ w2749 _ _] -> [_ _ w2763 _]
          tunnel: [_ _ _ w2813] -> w2737
          tunnel: w2735 -> [_ _ w2764 _]
          tunnel: "Raw DF in Orig Pos?" -> [_ _ w2761 _]
          tunnel: w2732 -> [_ _ _ w2810]
          frame #0 {
            n1275 = global read "Results_plotter_Global.vi" "Plot Index values"() -> (w2742:dbl[][])
            n1276 = global read "Results_plotter_Global.vi" "Row Reference"() -> (w2743:i32[][])
            n1277 = Index Array(array=w2742, index (row)=2) -> (element=w2740:dbl[])  [unwired: 1 in]
            n1278 = for {
              tunnel: w2743 -> [w2747]
              tunnel: w2740 -> [w2746] mode=indexing
              tunnel: [w2745] -> w2739 mode=indexing
              n1279 = Index Array(array=w2747, index (row)=w2746) -> (element=w2745:i32[])  [unwired: 1 in]
            }
            n1280 = local write "Delete Plotted data from file"(FALSE ("Save All data")) -> ()
          }
          frame #1 {
            n1281 = Index Array(array=w2752, index (col)=0 ("disabled index (col)")) -> (element=w2748:i32[])  [unwired: 1 in]
            n1282 = for {
              shift-right: [w2754] -> w2749
              shift-left: i32[] [] -> [w2755]
              tunnel: w2748 -> [w2753] mode=indexing
              n1283 = Search 1D Array(1D array=w2755, element=w2753) -> (index of element=w2756:i32)  [unwired: 1 out]
              n1284 = case shown="-1" w2756 {
                tunnel: w2755 -> [w2757 w2760]
                tunnel: [w2757 w2759] -> w2754
                tunnel: w2753 -> [_ w2758]
                frame 0, Default {
                }
                frame -1 {
                  n1285 = Build Array (concatenate)(w2760, w2758) -> (w2759:i32[])
                }
              }
            }
          }
          frame #2 {
            n1286 = for {
              tunnel: w2764 -> [w2769]
              tunnel: w2763 -> [w2766] mode=indexing
              tunnel: w2762 -> [w2767]
              tunnel: w2761 -> [w2765]
              # "New Values"
              # "Row in file"
              n1287 = Index Array(array=w2769, index=w2766) -> (element=w2768:path)
              n1288 = stacked-sequence {
                seq-local: [w2774 _] -> [_ w2808]
                seq-local: [w2772 _] -> [_ w2804]
                tunnel: w2768 -> [_ w2809]
                tunnel: w2767 -> [w2776 _]
                tunnel: w2766 -> [w2775 _]
                tunnel: w2765 -> [_ w2807]
                frame #0 {
                  n1289 = global read "Results_plotter_Global.vi" "New Values In"() -> (w2770:string[][])
                  n1290 = for {
                    tunnel: w2775 -> [w2787]
                    tunnel: w2776 -> [w2783] mode=indexing
                    shift-right: [w2781] -> w2774
                    shift-left: i32[] [] -> [w2782]
                    shift-right: [w2780] -> w2772
                    shift-left: string[][] [] -> [w2779]
                    tunnel: w2770 -> [w2778]
                    i -> [w2777]
                    n1291 = Index Array(array=w2783, index=0) -> (element=w2785:i32)
                    n1292 = Equal?(x=w2785, y=w2787) -> (x = y?=w2784:bool)
                    n1293 = case shown="True" w2784 {
                      tunnel: w2783 -> [_ w2793]
                      tunnel: w2782 -> [w2789 w2798]
                      tunnel: [w2789 w2796] -> w2781
                      tunnel: w2779 -> [w2788 w2794]
                      tunnel: [w2788 w2795] -> w2780
                      tunnel: w2778 -> [_ w2791]
                      tunnel: w2777 -> [_ w2790]
                      frame False {
                      }
                      frame True {
                        n1294 = Index Array(array=w2791, index (row)=w2790) -> (element=w2792:string[])  [unwired: 1 in]
                        n1295 = Build Array (concatenate)(w2794, w2792) -> (w2795:string[][])
                        n1296 = Index Array(array=w2793, index=1) -> (element=w2797:i32)
                        n1297 = Build Array (concatenate)(w2798, w2797) -> (w2796:i32[])
                      }
                    }
                  }
                }
                frame #1 {
                  w2803 = FALSE  # Edit all Rows?
                  w2805 = FALSE  # Edit Raw Data Header Info
                  w2806 = FALSE  # Value  Constant?
                  n1298 = local read "Edit Raw Data Files?"() -> (w2800:bool)
                  n1299 = local read "Job Directory"() -> (w2802:path)
                  n1300 = global read "Results_plotter_Global.vi" "New Chs In"() -> (w2801:string[])
                  n1301 = call "Add_Update_Values.vi"("Filename"=w2809, "Value  Constant?"=w2806, "Edit Raw data files?"=w2800, "New Chs In"=w2801, "Edit Raw Data Header Info"=w2805, "New Values In"=w2804, "Selected Rows"=w2808, "Edit all Rows?"=w2803, "Raw DF in Orig Pos?"=w2807, "Job Directory"=w2802) -> ()  [unwired: 1 in, 5 out]
                }
              }
            }
          }
          frame #3 {
            n1302 = local read "nRows"() -> (w2812:i32)
            n1303 = Less?(x=w2812, y=w2810) -> (x < y?=w2811:bool)
            n1304 = Current VI's Path() -> (path=w2814:path)
            n1305 = case shown="True" w2811 {
              tunnel: ["Create Selectors" "Initialise" ("t")] -> w2813
              frame False {
              }
              frame True {
              }
            }
            n1306 = call "Bring_to_front.vi"("path"=w2814) -> ()
          }
        }
      }
      frame "Save XY plot as jpg" {
        n1307 = local read "Create picture Vi Name"() -> (w2821:string)
        n1308 = local read "Job Directory"() -> (w2824:path)
        n1309 = global read "Constants_global.vi" "EnFlo SW Folder"() -> (w2826:path)
        n1310 = Build Path(base path=w2826, name or relative path=path "Anemometry/Anemometry Sub Vis/Data_plotting_vis/XY Plot Vis") -> (appended path=w2822:path)
        n1311 = call "Remote_call_prep.vi"("Vi Name in"=w2821, "Job Directory In"=w2824, "VI Directory"=w2822) -> ("Vi Name out"=w2823:string, "Job Directory out"=w2819:path, "cancelled"=w2818:bool)
        n1312 = local write "Create picture Vi Name"(w2823) -> ()
        n1313 = local write "Job Directory"(w2819) -> ()
        n1314 = Build Path(base path=w2822, name or relative path=w2823) -> (appended path=w2820:path)
        n1315 = case shown="False" w2818 {
          tunnel: [w2839 FALSE ("Saved Automatically?")] -> w2829
          tunnel: [w2838 path "" ("Plot data file")] -> w2828
          tunnel: [w2837 "" ("Tex Info String")] -> w2827
          tunnel: w2820 -> [w2836 _]
          tunnel: w2819 -> [w2835 _]
          frame False {
            n1316 = Open VI Reference(type specifier VI Refnum (for type only)="type specifier VI Refnum (for type only) 2", vi path=w2836) -> (vi reference=w2846:refnum<vi>, error out=w2845:errorcluster)  [unwired: 1 in, 3 out]
            n1317 = property class="VI Interface Type 2"(reference=w2846, error in=w2845, "Front Panel Window:Open"=TRUE) -> (reference out=w2842:refnum<vi>, error out=w2843:errorcluster)
            n1318 = global read "Results_plotter_Global.vi" "XY Graph Cluster"() -> (w2840:cluster{dbl[], dbl[]}[])
            n1319 = call-by-ref "?"(reference=w2842, error in=w2843, "Plot Array"=w2840, "Template"=w2835) -> (reference out=w2848:refnum<vi>, error out=w2847:errorcluster, "Saved Automatically?"=w2839:bool, "Tex Info String"=w2837:string, "Plot data file"=w2838:path)
            n1320 = Close Reference(reference=w2848, error in (no error)=w2847) -> ()  [unwired: 1 out]
          }
          frame True {
          }
        }
        n1321 = local write "Save Plot as jpg"(FALSE ("Save All data")) -> ()
        n1322 = case shown="True" w2829 {
          tunnel: w2828 -> [_ w2860]
          tunnel: [w2852 "Save Plot Data"] -> w2817
          tunnel: w2827 -> [_ w2858]
          frame False {
            n1323 = global read "Results_plotter_Global.vi" "New Chs In"() -> (w2857:string[])
            n1324 = Array Size(array=w2857) -> (size(s)=w2856:i32)
            n1325 = Greater Than 0?(x=w2856) -> (x > 0?=w2855:bool)
            n1326 = Select(t="Input calculated values", s=w2855, f="Create Selectors") -> (s? t:f=w2852:string)
          }
          frame True {
            n1327 = local write "Output Filename"(w2860) -> ()
            n1328 = local write "Header"(w2858) -> ()
          }
        }
      }
      frame "Full Res file manipulator" {
        n1329 = local read "Result files to read"() -> (w2870:path[])
        n1330 = local read "Output Filename"() -> (w2868:path)
        n1331 = local read "Mode"() -> (w2869:T7)
        n1332 = local read "Raw DF in Orig Pos?"() -> (w2861:bool)
        n1333 = global read "Results_plotter_Global.vi" "New Values In"() -> (w2863:string[][])
        n1334 = local read "Plotted rows only?"() -> (w2862:bool)
        n1335 = global read "Results_plotter_Global.vi" "New Chs In"() -> (w2864:string[])
        n1336 = stacked-sequence {
          seq-local: [w2875 _ _ _ _] -> [_ w2903 w2956 _ _]
          seq-local: [_ w2902 _ _ _] -> [_ _ w2939 _ _]
          seq-local: [_ w2898 _ _ _] -> [_ _ w2948 _ _]
          seq-local: [_ _ w2946 _ _] -> [_ _ _ w3200 _]
          seq-local: [_ _ w2945 _ _] -> [_ _ _ w3199 _]
          seq-local: [_ _ w2940 _ _] -> [_ _ _ w3196 _]
          tunnel: [_ _ _ w3203 _] -> w2872
          tunnel: w2870 -> [_ _ w2957 _ _]
          tunnel: w2869 -> [_ w2900 w2955 w3201 _]
          tunnel: w2868 -> [_ _ w2954 _ _]
          tunnel: w2862 -> [w2874 _ w2953 _ _]
          tunnel: w2864 -> [_ _ w2952 _ _]
          tunnel: w2867 -> [_ _ w2951 w3197 _]
          tunnel: w2866 -> [_ _ w2950 w3198 _]
          tunnel: w2861 -> [_ _ w2949 _ _]
          tunnel: w2865 -> [_ _ _ w3202 _]
          tunnel: w2863 -> [_ _ w2942 _ _]
          frame #0 {
            n1337 = global read "Results_plotter_Global.vi" "Row Reference"() -> (w2876:i32[][])
            n1338 = case shown="True" w2874 {
              tunnel: w2876 -> [w2878 w2879]
              tunnel: [w2878 w2880] -> w2875
              frame False {
              }
              frame True {
                n1339 = local read "Plotted Series"() -> (w2882:bool[][])
                n1340 = for {
                  tunnel: w2882 -> [w2889]
                  shift-right: [w2883] -> w2880
                  shift-left: i32[][] [] -> [w2885]
                  tunnel: w2879 -> [w2884] mode=indexing
                  i -> [w2888]
                  n1341 = Index Array(array=w2889, index (col)=w2888) -> (element=w2887:bool[])  [unwired: 1 in]
                  n1342 = Or Array Elements(Boolean array=w2887) -> (logical OR=w2886:bool)
                  n1343 = case shown="True" w2886 {
                    tunnel: w2885 -> [w2890 w2893]
                    tunnel: w2884 -> [_ w2892]
                    tunnel: [w2890 w2891] -> w2883
                    frame False {
                    }
                    frame True {
                      n1344 = Build Array (concatenate)(w2893, w2892) -> (w2891:i32[][])
                    }
                  }
                }
              }
            }
            n1345 = local write "Delete Plotted data from file"(FALSE ("Save All data")) -> ()
          }
          frame #1 {
            n1346 = local read "Job Directory"() -> (w2899:path)
            n1347 = case shown="\"Edit Raw Data file header\"" w2900 {
              tunnel: [FALSE FALSE FALSE w2920 w2923 w2926 w2929 w2932] -> w2901
              tunnel: [w2912 w2914 w2916 w2918 w2921 w2924 w2927 w2930] -> w2898
              tunnel: w2899 -> [w2912 w2914 w2916 w2919 w2922 w2925 w2928 w2931]
              tunnel: [w2912 w2914 w2916 w2918 w2921 w2924 w2927 w2930] -> w2897
              frame "Post Process Plotted Rows" {
              }
              frame "Save file" {
              }
              frame "Plot EnFlo Tunnel Display" {
              }
              frame "Delete unwanted rows" {
                n1348 = call "Remote_call_prep.vi"("Job Directory In"=w2919) -> ("Job Directory out"=w2918:path)  [unwired: 2 in, 2 out]
                n1349 = local write "Job Directory"(w2918) -> ()
                n1350 = Not Equal?(x=w2919, y=w2918) -> (x != y?=w2920:bool)
              }
              frame "Add Inlet Temperature Offset" {
                n1351 = call "Remote_call_prep.vi"("Job Directory In"=w2922) -> ("Job Directory out"=w2921:path)  [unwired: 2 in, 2 out]
                n1352 = local write "Job Directory"(w2921) -> ()
                n1353 = Not Equal?(x=w2922, y=w2921) -> (x != y?=w2923:bool)
              }
              frame "Edit Values with constants" {
                n1354 = call "Remote_call_prep.vi"("Job Directory In"=w2925) -> ("Job Directory out"=w2924:path)  [unwired: 2 in, 2 out]
                n1355 = local write "Job Directory"(w2924) -> ()
                n1356 = Not Equal?(x=w2925, y=w2924) -> (x != y?=w2926:bool)
              }
              frame "Edit values per row" {
                n1357 = call "Remote_call_prep.vi"("Job Directory In"=w2928) -> ("Job Directory out"=w2927:path)  [unwired: 2 in, 2 out]
                n1358 = local write "Job Directory"(w2927) -> ()
                n1359 = Not Equal?(x=w2928, y=w2927) -> (x != y?=w2929:bool)
              }
              frame "Edit Raw Data file header" {
                n1360 = call "Remote_call_prep.vi"("Job Directory In"=w2931) -> ("Job Directory out"=w2930:path)  [unwired: 2 in, 2 out]
                n1361 = local write "Job Directory"(w2930) -> ()
                n1362 = Not Equal?(x=w2931, y=w2930) -> (x != y?=w2932:bool)
              }
            }
            n1363 = Index Array(array=w2903, index (col)=0 ("disabled index (col)")) -> (element=w2895:i32[])  [unwired: 1 in]
            n1364 = for {
              shift-right: [w2905] -> w2902
              shift-left: i32[] [] -> [w2906]
              tunnel: w2895 -> [w2904] mode=indexing
              n1365 = Search 1D Array(1D array=w2906, element=w2904) -> (index of element=w2907:i32)  [unwired: 1 out]
              n1366 = case shown="-1" w2907 {
                tunnel: w2906 -> [w2908 w2911]
                tunnel: [w2908 w2910] -> w2905
                tunnel: w2904 -> [_ w2909]
                frame 0, Default {
                }
                frame -1 {
                  n1367 = Build Array (concatenate)(w2911, w2909) -> (w2910:i32[])
                }
              }
            }
            n1368 = case shown="True" w2901 {
              tunnel: w2897 -> [_ w2934]
              frame False {
              }
              frame True {
                n1369 = local read "Template"() -> (w2933:path)
                n1370 = Path To String(path=w2934) -> (string=w2937:string)
                n1371 = call "Read_Write_Template.vi"("Template File"=w2933, "Mode"=Global_mode."Write Global to File", "Single Value In"=w2937, "Data type"="Log Folder Name" ("Variable name")) -> ()  [unwired: 4 in, 8 out]
              }
            }
          }
          frame #2 {
            w2944 = path[] []
            n1372 = Array Size(array=w2939) -> (size(s)=w2938:i32)
            n1373 = local read "Full_Res_Results_Folder"() -> (w2943:path)
            n1374 = for {
              tunnel: w2957 -> [w2981]
              tunnel: w2939 -> [w2978] mode=indexing
              tunnel: w2956 -> [w2979]
              tunnel: w2955 -> [w2977]
              tunnel: w2954 -> [w2976]
              tunnel: w2953 -> [w2975]
              tunnel: w2952 -> [w2974]
              tunnel: w2951 -> [w2973]
              tunnel: w2950 -> [w2972]
              tunnel: w2949 -> [w2971]
              tunnel: w2948 -> [w2970]
              shift-right: [w2969] -> _
              shift-left: FALSE -> [w2968]
              shift-right: [w2966] -> w2946
              shift-left: w2944 -> [w2967]
              shift-right: [w2964] -> w2945
              shift-left: w2944 -> [w2965]
              tunnel: w2943 -> [w2963]
              tunnel: w2942 -> [w2962]
              shift-right: [w2960] -> w2940
              shift-left: i32[] [] -> [w2961]
              tunnel: w2938 -> [w2958]
              i -> [w2959]
              # "Row No in file"
              # "Row No in plotter"
              n1375 = Index Array(array=w2981, index=w2978) -> (element=w2980:path)
              n1376 = stacked-sequence {
                seq-local: [w2986 _ _ _] -> [_ w3022 w3078 _]
                seq-local: [_ w3020 _ _] -> [_ _ w3077 _]
                seq-local: [w2982 _ _ _] -> [_ _ w3070 w3194]
                tunnel: w2980 -> [_ w3021 w3079 _]
                tunnel: w2979 -> [w2996 _ _ _]
                tunnel: w2978 -> [w2989 _ _ _]
                tunnel: w2977 -> [_ w3019 w3076 _]
                tunnel: w2976 -> [_ _ w3075 _]
                tunnel: w2975 -> [_ _ w3074 _]
                tunnel: w2974 -> [_ _ w3073 _]
                tunnel: w2973 -> [_ _ w3072 _]
                tunnel: w2972 -> [_ _ w3071 _]
                tunnel: w2971 -> [_ _ w3069 _]
                tunnel: w2970 -> [_ _ w3068 _]
                tunnel: [_ w3018 _ _] -> w2969
                tunnel: w2968 -> [_ w3017 _ _]
                tunnel: w2967 -> [_ _ w3067 _]
                tunnel: [_ _ w3066 _] -> w2966
                tunnel: w2965 -> [_ _ w3065 _]
                tunnel: [_ _ w3064 _] -> w2964
                tunnel: w2963 -> [_ _ w3063 _]
                tunnel: w2962 -> [_ _ w3062 _]
                tunnel: w2961 -> [_ _ _ w3195]
                tunnel: [_ _ _ w3193] -> w2960
                tunnel: w2959 -> [_ _ w3061 _]
                tunnel: w2958 -> [_ _ w3060 _]
                frame #0 {
                  w2995 = i32[] []
                  # "10/30/13\n#optimation"
                  n1377 = global read "Results_plotter_Global.vi" "Row Reference"() -> (w2994:i32[][])
                  n1378 = local read "Cursor index"() -> (w2993:i32)
                  n1379 = for {
                    tunnel: w2989 -> [w3005]
                    tunnel: w2996 -> [w3001] mode=indexing
                    shift-right: [w2999] -> w2987
                    shift-left: w2995 -> [w3000]
                    shift-right: [w2998] -> w2983
                    shift-left: w2995 -> [w2997]
                    n1380 = Index Array(array=w3001, index=0) -> (element=w3003:i32)
                    n1381 = Equal?(x=w3003, y=w3005) -> (x = y?=w3002:bool)
                    n1382 = case shown="True" w3002 {
                      tunnel: w3001 -> [_ w3009]
                      tunnel: w3000 -> [w3007 w3015]
                      tunnel: [w3007 w3013] -> w2999
                      tunnel: w2997 -> [w3006 w3011]
                      tunnel: [w3006 w3012] -> w2998
                      frame False {
                      }
                      frame True {
                        n1383 = Index Array(array=w3009, index=2) -> (element=w3008:i32)
                        n1384 = Build Array (concatenate)(w3011, w3008) -> (w3012:i32[])
                        n1385 = Index Array(array=w3009, index=1) -> (element=w3014:i32)
                        n1386 = Build Array (concatenate)(w3015, w3014) -> (w3013:i32[])
                      }
                    }
                  }
                  n1387 = Index Array(array=w2994, index (row)=w2993) -> (element=w2991:i32[])  [unwired: 1 in]
                  n1388 = local read "Selected Row?"() -> (w2984:bool)
                  n1389 = Index Array(array=w2991, index #1=0 ("index"), index #2=1 ("index")) -> (element #2=w2988:i32)  [unwired: 1 out]
                  n1390 = Build Array(w2988) -> (w2985:i32[])
                  n1391 = Select(t=w2985, s=w2984, f=w2983) -> (s? t:f=w2982:i32[])
                  n1392 = Select(t=w2985, s=w2984, f=w2987) -> (s? t:f=w2986:i32[])
                }
                frame #1 {
                  n1393 = case shown="\"Add Inlet Temperature Offset\"" w3019 {
                    tunnel: w3022 -> [_ _ _ _ _ _ _ w3043]
                    tunnel: w3021 -> [_ _ _ _ _ _ _ w3041]
                    tunnel: [TRUE ("T button?") TRUE ("T button?") TRUE ("T button?") TRUE ("T button?") TRUE ("T button?") TRUE ("T button?") TRUE ("T button?") w3040] -> w3020
                    tunnel: [w3023 w3025 w3028 w3030 w3032 w3034 w3036 w3039] -> w3018
                    tunnel: w3017 -> [w3023 w3025 w3028 w3030 w3032 w3034 w3036 w3038]
                    frame "Save file" {
                    }
                    frame "Add Inlet Temperature Offset" {
                    }
                    frame "Plot EnFlo Tunnel Display" {
                      n1394 = local read "Index when last plotted"() -> (→"Index when last displayed":i32)
                    }
                    frame "Edit values per row" {
                    }
                    frame "Edit Values with constants" {
                    }
                    frame "Edit Raw Data file header" {
                    }
                    frame "Post Process Plotted Rows" {
                    }
                    frame "Delete unwanted rows" {
                      n1395 = Array Size(array=w3043) -> (size(s)=w3042:i32)
                      n1396 = case shown="False" w3038 {
                        tunnel: w3042 -> [w3052 _]
                        tunnel: w3041 -> [w3051 _]
                        tunnel: [w3046 w3059] -> w3040
                        tunnel: [w3045 w3059] -> w3039
                        frame False {
                          n1397 = Format Into String(format string="Remove %d rows from \"%s\"", w3052, w3051) -> (resulting string=w3049:string)  [unwired: 2 in, 1 out]
                          n1398 = call <vilib>:"Three Button Dialog.vi"("Allow user to close window? (TRUE)"=TRUE, "Right Button Text (\"Cancel\")"="Yes To All Files" ("Right Button Text (\"Cancel\")"), "message"=w3049) -> ("Which Button?"=w3047:T15)  [unwired: 3 in, 5 out]
                          n1399 = case shown="\"Left Button\"" w3047 {
                            tunnel: [TRUE TRUE w3057 w3058] -> w3046
                            tunnel: [FALSE TRUE w3057 w3058] -> w3045
                            frame "Left Button" {
                            }
                            frame "Right Button" {
                            }
                            frame "Center Button" {
                              w3057 = FALSE
                            }
                            frame "Window Close" {
                              w3058 = FALSE
                            }
                          }
                        }
                        frame True {
                          w3059 = TRUE
                        }
                      }
                    }
                  }
                }
                frame #2 {
                  n1400 = case shown="True" w3077 {
                    tunnel: w3079 -> [_ w3100]
                    tunnel: w3078 -> [_ w3099]
                    tunnel: w3076 -> [_ w3098]
                    tunnel: w3075 -> [_ w3097]
                    tunnel: w3074 -> [_ w3096]
                    tunnel: w3073 -> [_ w3095]
                    tunnel: w3072 -> [_ w3094]
                    tunnel: w3071 -> [_ w3093]
                    tunnel: w3070 -> [_ w3092]
                    tunnel: w3069 -> [_ w3091]
                    tunnel: w3068 -> [_ w3090]
                    tunnel: w3067 -> [w3081 w3089]
                    tunnel: [w3081 w3088] -> w3066
                    tunnel: w3065 -> [w3080 w3087]
                    tunnel: [w3080 w3086] -> w3064
                    tunnel: w3063 -> [_ w3085]
                    tunnel: w3062 -> [_ w3084]
                    tunnel: w3061 -> [_ w3083]
                    tunnel: w3060 -> [_ w3082]
                    frame False {
                    }
                    frame True {
                      n1401 = case shown="\"Edit Values with constants\"" w3098 {
                        tunnel: w3100 -> [w3106 w3112 w3130 w3137 w3143 w3164 w3181]
                        tunnel: w3099 -> [w3109 w3119 w3129 w3136 w3144 w3163 w3180]
                        tunnel: w3097 -> [_ _ _ _ _ _ _]
                        tunnel: w3096 -> [_ _ _ _ _ w3161 w3178]
                        tunnel: w3095 -> [_ _ _ _ _ w3159 w3176]
                        tunnel: w3094 -> [_ _ _ _ w3142 _ w3175]
                        tunnel: w3093 -> [_ _ _ _ w3145 _ w3173]
                        tunnel: w3092 -> [_ _ _ _ w3146 _ w3172]
                        tunnel: w3091 -> [_ _ _ _ _ w3158 w3170]
                        tunnel: w3090 -> [_ _ _ _ _ w3157 w3169]
                        tunnel: w3089 -> [w3108 w3116 w3128 w3139 w3148 w3155 w3167]
                        tunnel: [w3108 w3117 w3128 w3139 w3148 w3155 w3167] -> w3088
                        tunnel: w3087 -> [w3107 w3115 w3127 w3138 w3147 w3154 w3166]
                        tunnel: [w3107 w3113 w3127 w3138 w3147 w3154 w3166] -> w3086
                        tunnel: w3085 -> [w3105 _ _ _ _ _ _]
                        tunnel: w3084 -> [_ _ _ _ _ w3153 _]
                        tunnel: w3083 -> [_ _ _ w3132 _ _ _]
                        tunnel: w3082 -> [_ _ _ w3134 _ _ _]
                        frame "Save file" {
                          n1402 = Strip Path(path=w3106) -> (name=w3103:string)  [unwired: 1 out]
                          n1403 = call "Add_filename_suffix.vi"("Filename"=w3103, "Suffix to add"=".xls") -> ("Filename out"=w3101:string)  [unwired: 3 out]
                          n1404 = Build Path(base path=w3105, name or relative path=w3101) -> (appended path=w3104:path)
                          n1405 = call "Save_full_Res_rows.vi"("Selected Rows"=w3109, "Filename to write"=w3104, "Filename Orig"=w3106) -> ()  [unwired: 2 out]
                        }
                        frame "Edit Raw Data file header", Default {
                          n1406 = call "GetRawDataFilePaths.vi"("Results file or Folder"=w3112) -> ("RawDataFilePaths"=w3110:string[], "RowNumbers"=w3111:i32[])  [unwired: 9 in]
                          n1407 = for {
                            tunnel: w3110 -> [w3126]
                            tunnel: w3119 -> [w3120] mode=indexing
                            tunnel: [w3124] -> w3118 mode=indexing
                            tunnel: [w3123] -> w3114 mode=indexing
                            tunnel: w3112 -> [w3123]
                            tunnel: w3111 -> [w3122]
                            n1408 = Search 1D Array(1D array=w3122, element=w3120) -> (index of element=w3121:i32)  [unwired: 1 in]
                            n1409 = Index Array(array=w3126, index=w3121) -> (element=w3125:string)
                            n1410 = call "String_to_Pathname.vi"("Input String"=w3125) -> ("path"=w3124:path)
                          }
                          n1411 = Build Array (concatenate)(w3115, w3114) -> (w3113:path[])
                          n1412 = Build Array (concatenate)(w3116, w3118) -> (w3117:path[])
                        }
                        frame "Delete unwanted rows" {
                          n1413 = call "Delete_unwanted_rows.vi"("Selected Rows"=w3129, "Filename"=w3130) -> ()  [unwired: 1 out]
                        }
                        frame "Plot EnFlo Tunnel Display" {
                          n1414 = Decrement(x=w3134) -> (x-1=w3133:i32)
                          n1415 = Equal To 0?(x=w3132) -> (x = 0?=w3135:bool)
                          n1416 = Equal?(x=w3133, y=w3132) -> (x = y?=w3131:bool)
                          n1417 = call "Get_requested_rows_from_files.vi"("Last File"=w3131, "First file"=w3135, "Filename"=w3137, "Selected Rows"=w3136) -> ()  [unwired: 3 in]
                        }
                        frame "Add Inlet Temperature Offset" {
                          n1418 = for {
                            tunnel: w3146 -> [w3151] mode=indexing
                            tunnel: w3145 -> [w3150]
                            tunnel: [w3149] -> w3141 mode=indexing
                            n1419 = Index Array(array=w3150, index (row)=w3151) -> (element=w3149:string[])  [unwired: 1 in]
                          }
                          n1420 = local read "Job Directory"() -> (w3140:path)
                          n1421 = call "Get_Inlet_temps_from_files.vi"("Templated Plotted channels"=w3141, "Job Directory"=w3140, "Templated Channel Names"=w3142, "Filename"=w3143, "Selected Rows"=w3144) -> ()  [unwired: 7 in]
                        }
                        frame "Edit Values with constants" {
                          w3162 = TRUE  # Value  Constant?
                          n1422 = local read "Edit Raw Data Header Info"() -> (w3156:bool)
                          n1423 = Not(x=w3161) -> (.not. x?=w3160:bool)
                          n1424 = call "Add_Update_Values.vi"("Filename"=w3164, "Value  Constant?"=w3162, "Edit Raw data files?"="Edit Raw Data Files?", "New Chs In"=w3159, "Edit Raw Data Header Info"=w3156, "New Values In"=w3153, "Selected Rows"=w3163, "Edit all Rows?"=w3160, "Raw DF in Orig Pos?"=w3158, "Job Directory"=w3157) -> ()  [unwired: 1 in, 5 out]
                        }
                        frame "Edit values per row" {
                          w3168 = FALSE  # Edit Raw Data Header Info
                          w3179 = FALSE  # Value  Constant?
                          n1425 = for {
                            tunnel: w3176 -> [w3192] mode=indexing
                            tunnel: w3175 -> [w3191]
                            tunnel: [w3190] -> w3174 mode=indexing
                            n1426 = Search 1D Array(1D array=w3191, element=w3192) -> (index of element=w3190:i32)  [unwired: 1 out]
                          }
                          n1427 = for {
                            tunnel: w3174 -> [w3186]
                            tunnel: w3173 -> [w3185]
                            tunnel: w3172 -> [w3183] mode=indexing
                            tunnel: [w3182] -> w3171 mode=indexing
                            n1428 = Index Array(array=w3185, index (row)=w3183) -> (element=w3184:string[])  [unwired: 1 in]
                            n1429 = for {
                              tunnel: w3186 -> [w3189] mode=indexing
                              tunnel: w3184 -> [w3188]
                              tunnel: [w3187] -> w3182 mode=indexing
                              n1430 = Index Array(array=w3188, index=w3189) -> (element=w3187:string)
                            }
                          }
                          n1431 = local read "Edit Raw Data Files?"() -> (w3165:bool)
                          n1432 = Not(x=w3178) -> (.not. x?=w3177:bool)
                          n1433 = call "Add_Update_Values.vi"("Filename"=w3181, "Value  Constant?"=w3179, "Edit Raw data files?"=w3165, "New Chs In"=w3176, "Edit Raw Data Header Info"=w3168, "New Values In"=w3171, "Selected Rows"=w3180, "Edit all Rows?"=w3177, "Raw DF in Orig Pos?"=w3170, "Job Directory"=w3169) -> ()  [unwired: 1 in, 5 out]
                        }
                      }
                    }
                  }
                }
                frame #3 {
                  n1434 = Build Array (concatenate)(w3195, w3194) -> (w3193:i32[])
                }
              }
            }
          }
          frame #3 {
            n1435 = case shown="\"Post Process Plotted Rows\"" w3201 {
              tunnel: ["Create Selectors" "Create Selectors" w3212 "Initialise" ("t") w3246 w3252 w3259 w3265] -> w3203
              tunnel: w3202 -> [_ _ _ _ w3243 w3249 w3256 w3262]
              tunnel: w3200 -> [w3204 _ w3211 _ _ _ _ _]
              tunnel: w3199 -> [_ _ w3210 _ _ _ _ _]
              tunnel: w3198 -> [_ _ w3209 _ _ _ _ _]
              tunnel: w3197 -> [_ _ w3208 _ _ _ _ _]
              tunnel: w3196 -> [_ _ w3207 _ _ _ _ _]
              frame "Edit Raw Data file header" {
                n1436 = call "Edit_Raw_DF_Header.vi"("Selected files"=w3204) -> ()  [unwired: 15 out]
              }
              frame "Plot EnFlo Tunnel Display" {
              }
              frame "Post Process Plotted Rows" {
                n1437 = stacked-sequence {
                  seq-local: [_ w3215 _] -> [_ _ w3238]
                  tunnel: [_ _ "Create Selectors"] -> w3212
                  tunnel: w3211 -> [_ _ w3240]
                  tunnel: w3210 -> [_ _ w3239]
                  tunnel: w3209 -> [_ w3217 _]
                  tunnel: w3208 -> [_ _ w3236]
                  tunnel: w3207 -> [_ w3214 _]
                  frame #0 {
                    n1438 = local write "Post Process Plotted Data"(FALSE ("Post Process Plotted Data")) -> ()
                  }
                  frame #1 {
                    n1439 = global read "Results_plotter_Global.vi" "Precision"() -> (w3216:string[])
                    n1440 = for {
                      tunnel: w3217 -> [w3219]
                      tunnel: w3216 -> [w3222]
                      tunnel: [w3221] -> w3215 mode=indexing
                      tunnel: w3214 -> [w3220] mode=indexing
                      n1441 = Index Array(array=w3219, index (row)=w3220) -> (element=w3218:string[])  [unwired: 1 in]
                      n1442 = for {
                        tunnel: w3218 -> [w3224] mode=indexing
                        tunnel: w3222 -> [w3223] mode=indexing
                        tunnel: [w3226] -> w3221 mode=indexing
                        n1443 = Fract/Exp String To Number(string=w3224) -> (offset past number=w3230:i32, number=w3227:dbl)  [unwired: 3 out]
                        n1444 = String Length(string=w3224) -> (length=w3231:i32)
                        n1445 = Equal?(x=w3231, y=w3230) -> (x = y?=w3228:bool)
                        n1446 = Empty String/Path?(string/path=w3224) -> (empty?=w3229:bool)
                        n1447 = Compound Arithmetic op=AND(invert w3229, w3228) -> (w3225:bool)
                        n1448 = case shown="True" w3225 {
                          tunnel: w3223 -> [_ w3234]
                          tunnel: w3227 -> [_ w3235]
                          tunnel: [w3232 w3233] -> w3226
                          tunnel: w3224 -> [w3232 _]
                          frame False {
                          }
                          frame True {
                            n1449 = call "Number_2_string.vi"("precision"=w3234, "number"=w3235) -> ("String"=w3233:string)
                          }
                        }
                      }
                    }
                  }
                  frame #2 {
                    n1450 = Build Array (concatenate)(w3236, w3238) -> (w3237:string[][])
                    n1451 = call "Post_Process_Profile_Remote.vi"("Results Plotter Rows"=w3237, "Raw Data files to PP"=w3240, "Current Results filenames"=w3239) -> ()  [unwired: 1 out]
                  }
                }
              }
              frame "Delete unwanted rows" {
              }
              frame "Edit Values with constants" {
                n1452 = local read "nRows"() -> (w3245:i32)
                n1453 = Less?(x=w3245, y=w3243) -> (x < y?=w3244:bool)
                n1454 = case shown="True" w3244 {
                  tunnel: ["Create Selectors" "Initialise" ("t")] -> w3246
                  frame False {
                  }
                  frame True {
                  }
                }
              }
              frame "Edit values per row" {
                n1455 = local read "nRows"() -> (w3251:i32)
                n1456 = Less?(x=w3251, y=w3249) -> (x < y?=w3250:bool)
                n1457 = case shown="True" w3250 {
                  tunnel: ["Create Selectors" "Initialise" ("t")] -> w3252
                  frame False {
                  }
                  frame True {
                  }
                }
              }
              frame "Add Inlet Temperature Offset" {
                n1458 = local read "nRows"() -> (w3258:i32)
                n1459 = Less?(x=w3258, y=w3256) -> (x < y?=w3257:bool)
                n1460 = case shown="True" w3257 {
                  tunnel: ["Create Selectors" "Initialise" ("t")] -> w3259
                  frame False {
                  }
                  frame True {
                  }
                }
                n1461 = local write "Add Inlet Temperature offset"(FALSE ("Add Inlet Temperature offset")) -> ()
              }
              frame "Save file" {
                n1462 = local read "nRows"() -> (w3264:i32)
                n1463 = Less?(x=w3264, y=w3262) -> (x < y?=w3263:bool)
                n1464 = case shown="True" w3263 {
                  tunnel: ["Create Selectors" "Initialise" ("t")] -> w3265
                  frame False {
                  }
                  frame True {
                  }
                }
              }
            }
          }
          frame #4 {
            n1465 = Current VI's Path() -> (path=w3268:path)
            n1466 = call "Bring_to_front.vi"("path"=w3268) -> ()
          }
        }
      }
      frame "Empty Results file array" {
        n1467 = local read "Template"() -> (w3270:path)
        n1468 = call "Valid_Path.vi"("Filename"=w3270) -> ("Valid Path?"=w3269:bool)
        n1469 = case shown="False" w3269 {
          tunnel: w3271 -> [w3280 _]
          frame False {
            n1470 = local write "Template"(w3280) -> ()
          }
          frame True {
          }
        }
        n1471 = property on="Result files to read" class="Arr (strict)"("Index Values"=u32[] [0] ("Write Attribute")) -> ()  [unwired: 2 in, 2 out]
        n1472 = local write "Result files to read"(path[] [] ("Result files to read")) -> ()
        n1473 = local write "Empty"(FALSE ("Empty")) -> ()
      }
      frame "Save Setup" {
        n1474 = local read "Create picture Vi Name"() -> (w3307:string)
        n1475 = local read "Additional X Values"() -> (w3313:dbl[])
        n1476 = local read "Additional Y Values"() -> (w3312:dbl[])
        n1477 = local read "Result files to read"() -> (w3315:path[])
        n1478 = local read "Output Filename"() -> (w3308:path)
        n1479 = local read "Multi Ordinate?"() -> (w3305:bool)
        n1480 = local read "Multi Ordinate"() -> (w3301:i32[])
        n1481 = local read "Intensity Plot?"() -> (w3306:bool)
        n1482 = local read "Filter Bins 1"() -> (w3303:i32[])
        n1483 = local read "Filter Bins 2"() -> (w3302:i32[])
        n1484 = local read "Filter Array"() -> (w3309:u16[])
        n1485 = local read "Transpose"() -> (w3314:bool)
        n1486 = local read "Template"() -> (w3287:path)
        n1487 = local read "Ordinate"() -> (w3311:u16)
        n1488 = local read "Absisca"() -> (w3310:u16)
        n1489 = call "Read_Write_Plot_Setup.vi"("Mode"=enum16{"Load", "Save"}."Load", "Setup filename"=w3296) -> ("Cluster 2"=w3316:T14)  [unwired: 1 in, 1 out]
        n1490 = Bundle By Name(cluster=w3316, "Result files to read"=w3315, "Template"=w3287, "Transpose"=w3314, "Additional X Values"=w3313, "Additional Y Values"=w3312, "Ordinate"=w3311, "Absisca"=w3310, "Filter Array"=w3309, "color and symbol"=TRUE, "Output Filename"=w3308, "Jpg Vi Name"=w3307, "Intensity Plot?"=w3306, "Multi Ordinate?"=w3305, "Filter Bins 1"=w3303, "Filter Bins 2"=w3302, "Multi Ordinate"=w3301) -> (w3304:T14)
        n1491 = global read "Trav_pos_global.vi" "Estimated Completion time"() -> (w3298:string)
        n1492 = local read "stop"() -> (w3295:bool)
        n1493 = feedback-in #1(w3287) -> ()
        n1494 = feedback #1() -> (w3286:path)  [unwired: 1 in]
        n1495 = call "Read_Write_Plot_Setup.vi"("Mode"=enum16{"Load", "Save"}."Save", "Setup filename"=w3296, "Cluster"=w3304) -> ()  [unwired: 2 out]
        n1496 = Equal?(x=w3287, y=w3286) -> (x = y?=w3282:bool)
        n1497 = Empty String/Path?(string/path=w3298) -> (empty?=w3292:bool)
        n1498 = Compound Arithmetic op=OR(w3295, invert w3292) -> (w3293:bool)
        n1499 = feedback #2() -> (w3285:path)  [unwired: 1 in]
        n1500 = feedback-in #2("Job Directory") -> ()
        n1501 = Equal?(x=w3285, y="Job Directory") -> (x = y?=w3283:bool)
        n1502 = And(x=w3282, y=w3283) -> (x .and. y?=w3281:bool)
        n1503 = local read "Save Setup"() -> (w3297:bool)
        n1504 = Select(t="End", s=w3293, f="Check modification dates?") -> (s? t:f=w3288:string)
        n1505 = case shown="False" w3281 {
          tunnel: w3287 -> [w3323 _]
          tunnel: "Job Directory" -> [w3322 _]
          frame False {
            n1506 = call "Path_2_String.vi"("Real Path"=w3322) -> ("Path String"=w3324:string)
            n1507 = call "Read_Write_Template.vi"("Template File"=w3323, "Mode"=Global_mode."Write Global to File", "Single Value In"=w3324, "Data type"="Log Folder Name" ("Variable name")) -> ()  [unwired: 4 in, 8 out]
          }
          frame True {
          }
        }
        n1508 = Select(t="Save to named setup file", s=w3297, f=w3288) -> (s? t:f=w3289:string)
      }
      frame "Save to named setup file" {
        w3328 = TRUE  # Save New File?
        n1509 = call "Save_current_setup.vi"("Save New File?"=w3328, "Setup File Type"=Setup_Filetype."Results File Plotter Setups") -> ()  [unwired: 4 out]
        n1510 = local write "Save Setup"(FALSE ("Save Setup")) -> ()
      }
      frame "End" {
        n1511 = local read "Template"() -> (w3339:path)
        n1512 = local read "Empty"() -> (w3340:bool)
        n1513 = call "Valid_Path.vi"("Filename"=w3339) -> ("Valid Path?"=w3338:bool)
        n1514 = case shown="True" w3340 {
          frame False {
          }
          frame True {
            n1515 = property on="Result files to read" class="Arr (strict)"("Index Values"=u32[] [0] ("Write Attribute")) -> ()  [unwired: 2 in, 2 out]
            n1516 = local write "Result files to read"(path[] [] ("Result files to read")) -> ()
            n1517 = local write "Empty"(FALSE ("Empty")) -> ()
          }
        }
        n1518 = case shown="False" w3338 {
          tunnel: w3341 -> [w3349 _]
          frame False {
            n1519 = local write "Template"(w3349) -> ()
          }
          frame True {
          }
        }
        n1520 = global write "Results_plotter_Global.vi" "Plot EnFlo Tunnel Display"(FALSE ("Plot EnFlo Tunnel Display")) -> ()
        n1521 = property on="stop" class="Bool (strict)"("Val(Sgnl)"=TRUE) -> ()  [unwired: 2 in, 2 out]
      }
    }
    n1522 = Wait (ms)(milliseconds to wait=u32 50) -> ()  [unwired: 1 out]
    "Current" <- w17
  }
  n1523 = while {
    tunnel: FALSE -> [w3351]
    stop <- w3350 stop-if-true
    # "Event structure wrapper"
    n1524 = local write "stop"(w3351) -> ()
    n1525 = event shown="[5] \"TinyPoints?\", \"InterpolationStyle\": Value Change" {
      selector: _ -> [_ _ _ _ _ _]
      dyn-events: _ -> [_ _ _ _ _ _]
      timeout: _ -> [_ _ _ _ _ _]
      tunnel: [_ _ w3370 _ _ _] -> w3350
      event Timeout {
        n1526 = event-data() -> ()  [unwired: 1 in, 3 out]
      }
      event Panel Resize {
        # "Code to resize the \"Red\" and Green Multiselects as window grows"
        # "Ajust the multi-selector sizes with the panel"
        n1527 = event-data() -> ("VIRef"=w3359:refnum<vi>, "NewBnds"=w3358:T21)  [unwired: 1 in, 6 out]
        n1528 = property class="VI"(reference=w3359) -> ("Minimum Panel Size"=w3365:T22)  [unwired: 1 in, 2 out]
        n1529 = Unbundle By Name(w3358) -> ("Right"=w3357:i16, "Left"=w3356:i16)
        n1530 = Unbundle By Name(w3365) -> ("Horizontal"=w3364:i16)
        n1531 = Subtract(x=w3357, y=w3356) -> (x-y=w3355:i16)
        n1532 = Subtract(x=w3355, y=w3364) -> (x-y=w3353:i16)
        n1533 = Add(x=w3353, y=i16 98) -> (x+y=w3361:i16)
        n1534 = expression code="x*2/3"(w3353) -> (w3354:i16)
        n1535 = expression code="x*1/3"(w3353) -> (w3352:i16)
        n1536 = property on="Single Series" class="LstBox (strict)"("Width"=w3361) -> ()  [unwired: 2 in, 2 out]
        n1537 = Add(x=w3352, y=i16 274) -> (x+y=w3366:i16)
        n1538 = Add(x=w3354, y=i16 302) -> (x+y=w3362:i16)
        n1539 = Add(x=w3352, y=281) -> (x+y=w3368:i32)
        n1540 = property on="Filter Bins 2" class="LstBox (strict)"("Width"=w3362, "Left"=w3368) -> ()  [unwired: 2 in, 2 out]
        n1541 = property on="Filter Bins 1" class="LstBox (strict)"("Width"=w3366) -> ()  [unwired: 2 in, 2 out]
      }
      event "stop": Value Change {
        n1542 = event-data() -> ("NewVal"=w3370:bool)  [unwired: 1 in, 5 out]
      }
      event Panel Close {
        n1543 = event-data() -> ()  [unwired: 1 in, 4 out]
        n1544 = local write "stop"(TRUE ("stop")) -> ()
      }
      event "ShowPix": Mouse Up {
        # "Retrieve path for Raw Data File; use to retrieve matching webcam pictures"
        n1545 = event-data() -> ()  [unwired: 1 in, 8 out]
        n1546 = local read "Result files to read"() -> (w3375:path[])
        n1547 = global read "Results_plotter_Global.vi" "Row Reference"() -> (w3373:i32[][])
        n1548 = local read "Cursor index"() -> (w3374:i32)
        n1549 = Index Array(array=w3373, index (row)=w3374) -> (element=w3378:i32[])  [unwired: 1 in]
        n1550 = Index Array(array=w3378, index #1=0 ("index"), index #2=1 ("index")) -> (element #1=w3376:i32, element #2=w3385:i32)
        n1551 = Index Array(array=w3375, index=w3376) -> (element=w3379:path)
        n1552 = call "GetRawDataFilePaths.vi"("Results file or Folder"=w3379) -> ("RawDataFilePaths"=w3380:string[], "RowNumbers"=w3383:i32[])  [unwired: 9 in]
        n1553 = Search 1D Array(1D array=w3383, element=w3385) -> (index of element=w3384:i32)  [unwired: 1 in]
        n1554 = Index Array(array=w3380, index=w3384) -> (element=w3381:string)
        n1555 = call "String_to_Pathname.vi"("Input String"=w3381) -> ("path"=w3372:path)
        n1556 = call "RetrievePix.vi"("RawDataFile"=w3372) -> ()  [unwired: 11 in]
      }
      event "TinyPoints?", "InterpolationStyle": Value Change {
        n1557 = event-data() -> ()  [unwired: 1 in, 6 out]
        n1558 = global write "Results_plotter_Global.vi" "InterpolationStyle"("InterpolationStyle") -> ()
        n1559 = global write "Results_plotter_Global.vi" "TinyPoints?"("TinyPoints?") -> ()
      }
    }
  }
